vi "H2O_DIAL_NCAR_4CH_v4.10.vi"() -> ()   [LabVIEW 2012]
uses:
  C:/Users/H2ODial/Desktop/Shared Telescope WV DIAL Code/Libraries and VIs/PowerMeterCommands.dll
  Shared Telescope WV DIAL Code/Libraries and VIs/PowerMeterCommands.dll
  <vilib>/DAQmx/write.llb/DAQmx Write (Digital 1D Bool NChan 1Samp 1Line).vi
  <vilib>/DAQmx/miscellaneous.llb/DAQmx Fill In Error Info.vi
  <vilib>/Analysis/baseanly.llb/Mean (DBL).vi
  AMCS_Data.vi
  Libraries and VIs/Scalar_Data.vi
  <vilib>/Analysis/NI_AALBase.lvlib
  Libraries and VIs/Scalar_Data_2.vi
  Libraries and VIs/Scalar_Data_4.vi
  Libraries and VIs/Scalar_Data_3.vi
  Shared Telescope WV DIAL Code/bristol/CLDevIFace.dll
panel:
  out "FileHour":i32=21
  out "L_Count":i32=670
  out "sigma_off_total":dbl[](array[numeric])=[5.545093346002325e-25, 5.513698314781969e-25, 5.482392638165798e-25, 5.45117700346153e-25, 5.420052094490138e-25, 5.389018591101994e-25, 5.35807716859337e-25, 5.327228497243776e-25, 5.296473241817102e-25, 5.265812061058967e-25, 5.235245607190952e-25, 5.204774525540416e-25, 5.17439945396719e-25, 5.144121022534048e-25, 5.11393985302133e-25, 5.083856558516785e-25, 5.053871743064082e-25, 5.023986001219567e-25, 4.994199917728618e-25, 4.964514067155941e-25, 4.9349290135305775e-25, 4.90544531006438e-25, 4.876063498767343e-25, 4.846784110224529e-25, 4.817607663241581e-25, 4.788534664693006e-25, 4.759565609097595e-25, 4.730700978566929e-25, 4.70194124242593e-25, 4.673286857118099e-25, 4.644738265927707e-25, 4.616295898870687e-25, 4.587960172474658e-25, 4.5597314896431265e-25, 4.531610239560122e-25, 4.503596797514039e-25, 4.47569152481693e-25, 4.447894768684054e-25, 4.420206862206039e-25, 4.392628124203261e-25, 4.365158859275847e-25, 4.337799357659035e-25, 4.310549895246989e-25, 4.283410733576763e-25, 4.256382119799841e-25, 4.2294642867403195e-25, 4.202657452853169e-25, 4.175961822281299e-25, 4.149377584922389e-25, 4.1229049164465202e-25, 4.096543978372992e-25, 4.0702949181683236e-25, 4.0441578692843654e-25, 4.0181329512767607e-25, 3.992220269942415e-25, 3.96641991736463e-25, 3.9407319720804376e-25, 3.915156499210381e-25, 3.8896935505642936e-25, 3.8643431648416273e-25, 3.8391053677102475e-25, 3.813980172052376e-25, 3.788967578068652e-25, 3.764067573453576e-25, 3.7392801336269163e-25, 3.7146052218886312e-25, 3.6900427895717113e-25, 3.6655927763183676e-25, 3.6412551102130396e-25, 3.6170297080280375e-25, 3.592916475433481e-25, 3.568915307165587e-25, 3.5450260873191323e-25, 3.5212486894953557e-25, 3.49758297708119e-25, 3.4740288034404592e-25, 3.4505860121784583e-25, 3.427254437338488e-25, 3.4040339036361268e-25, 3.3809242267276765e-25, 3.3579252134124988e-25, 3.3350366619025945e-25, 3.312258362003964e-25, 3.2895900954264883e-25, 3.2670316359662337e-25, 3.2445827497597403e-25, 3.2222431955291055e-25, 3.2000127248258437e-25, 3.1778910822374647e-25, 3.155878005644869e-25, 3.133973226455684e-25, 3.1121764698225313e-25, 3.0904874548876633e-25, 3.0689058950047053e-25, 3.0474314979719436e-25, 3.0260639662437082e-25, 3.0048029971594525e-25, 2.9836482831758435e-25, 2.962599512058786e-25, 2.9416563671167466e-25, 2.9208185274060903e-25, 2.90008566793984e-25, 2.879457459893465e-25, 2.8589335708021117e-25, 2.8385136647823233e-25, 2.818197402689904e-25, 2.7979844423464204e-25, 2.7778744387231733e-25, 2.757867044107587e-25, 2.737961908312855e-25, 2.718158678842996e-25, 2.6984570010800424e-25, 2.6788565184392253e-25, 2.659356872568504e-25, 2.639957703488535e-25, 2.620658649780614e-25, 2.6014593487307293e-25, 2.582359436501918e-25, 2.5633585482778302e-25, 2.5444563184328377e-25, 2.5256523806624473e-25, 2.506946368147788e-25, 2.488337913696908e-25, 2.4698266498768704e-25, 2.4514122091801807e-25, 2.4330942241302343e-25, 2.4148723274426624e-25, 2.396746152144881e-25, 2.3787153317177266e-25, 2.360779500217858e-25, 2.3429382923989676e-25, 2.3251913438553717e-25, 2.30753829112614e-25, 2.289978771825043e-25, 2.272512424756057e-25, 2.25513889003242e-25, 2.2378578091878363e-25, 2.220668825283397e-25, 2.2035715830323156e-25, 2.1865657288915057e-25, 2.169650911171393e-25, 2.1528267801378837e-25, 2.1360929881158006e-25, 2.1194491895763e-25, 2.102895041236874e-25, 2.0864302021492868e-25, 2.070054333784623e-25, 2.0537671001224436e-25, 2.0375681677230244e-25, 2.0214572058106931e-25, 2.0054338863372052e-25, 1.989497884059814e-25, 1.9736488765949925e-25, 1.9578865444868876e-25, 1.9422105712539158e-25, 1.9266206434388185e-25, 1.9111164506623173e-25, 1.8956976856478284e-25, 1.8803640442671668e-25, 1.8651152255647924e-25, 1.8499509317774677e-25, 1.8348708683587619e-25, 1.8198747439799888e-25, 1.8049622705463732e-25, 1.7901331631884819e-25, 1.775387140257627e-25, 1.7607239233152573e-25, 1.7461432371095203e-25, 1.7316448095559218e-25, 1.717228371700267e-25, 1.7028936576867277e-25, 1.6886404047118466e-25, 1.6744683529761906e-25, 1.660377245632093e-25, 1.6463668287207736e-25, 1.632436851109196e-25, 1.618587064418851e-25, 1.604817222950476e-25, 1.5911270836042792e-25, 1.5775164057945997e-25, 1.56398495136209e-25, 1.5505324844802238e-25, 1.5371587715593366e-25, 1.5238635811467746e-25, 1.510646683824263e-25, 1.4975078521023343e-25, 1.4844468603128529e-25, 1.4714634844992623e-25, 1.4585575023049792e-25, 1.4457286928608944e-25, 1.4329768366725881e-25, 1.4203017155042415e-25, 1.407703112267118e-25, 1.3951808109034195e-25, 1.3827345962734493e-25, 1.3703642540430184e-25, 1.3580695705732947e-25, 1.3458503328084848e-25, 1.3337063281714564e-25, 1.3216373444562365e-25, 1.3096431697251984e-25, 1.2977235922113967e-25, 1.2858784002202707e-25, 1.2741073820391008e-25, 1.262410325845275e-25, 1.2507870196238964e-25, 1.2392372510878126e-25, 1.2277608076014726e-25, 1.2163574761105352e-25, 1.2050270430775917e-25, 1.193769294421569e-25, 1.182584015463539e-25, 1.1714709908803334e-25, 1.1604300046571814e-25, 1.1494608400603252e-25, 1.1385632795946503e-25, 1.1277371049919547e-25, 1.1169820971849576e-25, 1.1062980362989263e-25, 1.0956847016453476e-25, 1.0851418717240022e-25, 1.0746693242300533e-25, 1.0642668360671284e-25, 1.0539341833638053e-25, 1.0436711415027306e-25, 1.0334774851444859e-25, 1.0233529882683514e-25, 1.01329742420825e-25, 1.0033105656977957e-25, 9.93392184918038e-26, 9.835420535448986e-26, 9.737599428132508e-26, 9.640456235622354e-26, 9.543988662985507e-26, 9.44819441258607e-26, 9.353071184649082e-26, 9.258616677861991e-26, 9.164828590007729e-26, 9.071704618481929e-26, 8.979242460918443e-26, 8.887439815711605e-26, 8.79629438247936e-26, 8.705803862565375e-26, 8.615965959431582e-26, 8.526778379078846e-26, 8.438238830295678e-26, 8.350345024925896e-26, 8.263094678112063e-26, 8.176485508356415e-26, 8.090515237617101e-26, 8.0051815912957e-26, 7.920482298141068e-26, 7.836415090070007e-26, 7.752977702020669e-26, 7.67016787158364e-26, 7.587983338670006e-26, 7.506421845116342e-26, 7.425481134179741e-26, 7.345158949991444e-26, 7.265453037023949e-26, 7.186361139388167e-26, 7.107881000268466e-26, 7.030010361112887e-26, 6.95274696098591e-26, 6.876088535839326e-26, 6.800032817697419e-26, 6.724577533923724e-26, 6.64972040650064e-26, 6.575459151231174e-26, 6.501791477027899e-26, 6.428715085196855e-26, 6.356227668734542e-26, 6.284326911690598e-26, 6.213010488505251e-26, 6.142276063456507e-26, 6.072121290089713e-26, 6.002543810738931e-26]
  out "sigma_on_total":dbl[](array[numeric])=[3.742206868641341e-23, 3.7429612618018996e-23, 3.7434726015285955e-23, 3.743740073660256e-23, 3.743762939303223e-23, 3.7435405357585175e-23, 3.743072276917427e-23, 3.742357654081436e-23, 3.7413962365246194e-23, 3.7401876719276805e-23, 3.738731686678352e-23, 3.737028086692236e-23, 3.735076757163706e-23, 3.732877663344878e-23, 3.7304308504649446e-23, 3.7277364438773654e-23, 3.724794649375737e-23, 3.721605752921234e-23, 3.7181701208374216e-23, 3.7144881996422916e-23, 3.710560515815649e-23, 3.70638767581906e-23, 3.70197036542659e-23, 3.6973093497816675e-23, 3.6924054726011473e-23, 3.6872596563618015e-23, 3.681872900813485e-23, 3.67624628345753e-23, 3.67038095801539e-23, 3.664278154392267e-23, 3.6579391774321e-23, 3.6513654065279726e-23, 3.6445582944273624e-23, 3.637519366398915e-23, 3.6302502195208586e-23, 3.622752521321382e-23, 3.6150280088780594e-23, 3.6070784875244904e-23, 3.598905830029354e-23, 3.590511974858799e-23, 3.581898925616457e-23, 3.573068749038446e-23, 3.5640235739972726e-23, 3.5547655901165024e-23, 3.54529704616676e-23, 3.5356202489615237e-23, 3.525737561411073e-23, 3.515651401168645e-23, 3.505364239248806e-23, 3.494878598162465e-23, 3.4841970503851443e-23, 3.473322216892923e-23, 3.462256765124002e-23, 3.4510034074664904e-23, 3.4395648998215893e-23, 3.427944039316459e-23, 3.416143662923538e-23, 3.404166645697518e-23, 3.3920158987192733e-23, 3.37969436777507e-23, 3.367205030906827e-23, 3.354550897358153e-23, 3.3417350052058163e-23, 3.328760419548489e-23, 3.315630231166496e-23, 3.302347554430607e-23, 3.2889155251170917e-23, 3.27533729936037e-23, 3.261616051196446e-23, 3.247754971153086e-23, 3.23375726447253e-23, 3.2196261488718373e-23, 3.205364853547713e-23, 3.19097661668077e-23, 3.176464684282408e-23, 3.1618323081121953e-23, 3.1470827443725446e-23, 3.1322192516661925e-23, 3.117245089355038e-23, 3.102163516320947e-23, 3.086977788993837e-23, 3.071691160162447e-23, 3.0563068767728277e-23, 3.0408281792659305e-23, 3.0252582994336664e-23, 3.009600459155118e-23, 2.9938578690686444e-23, 2.9780337272750084e-23, 2.962131217604643e-23, 2.946153508575282e-23, 2.930103752101369e-23, 2.9139850820520734e-23, 2.897800613217805e-23, 2.8815534400324565e-23, 2.865246635517646e-23, 2.848883249985849e-23, 2.8324663100586776e-23, 2.8159988178125756e-23, 2.799483749410663e-23, 2.782924054415838e-23, 2.7663226547735467e-23, 2.749682443924372e-23, 2.733006285954302e-23, 2.7162970146927096e-23, 2.6995574332980244e-23, 2.682790312890641e-23, 2.6659983923935745e-23, 2.649184377777944e-23, 2.632350941081864e-23, 2.6155007202662802e-23, 2.5986363183953e-23, 2.581760303295213e-23, 2.5648752067227738e-23, 2.5479835244432992e-23, 2.5310877152951883e-23, 2.5141902012463274e-23, 2.497293366703312e-23, 2.480399558458463e-23, 2.4635110851539856e-23, 2.446630217375111e-23, 2.4297591870097065e-23, 2.4129001874018873e-23, 2.3960553731103502e-23, 2.3792268595329617e-23, 2.362416723389737e-23, 2.3456270019069583e-23, 2.3288596933533007e-23, 2.312116756693998e-23, 2.295400111844486e-23, 2.2787116395407354e-23, 2.262053181239011e-23, 2.2454265396775957e-23, 2.2288334785005983e-23, 2.212275722623987e-23, 2.195754958303483e-23, 2.1792728333801465e-23, 2.1628309573890534e-23, 2.146430901613271e-23, 2.130074199768713e-23, 2.113762347784294e-23, 2.097496804215243e-23, 2.0812789905176965e-23, 2.0651102914863584e-23, 2.0489920552598092e-23, 2.0329255938621748e-23, 2.016912183458992e-23, 2.0009530646282707e-23, 1.985049442932356e-23, 1.969202488994444e-23, 1.9534133391617796e-23, 1.937683095535943e-23, 1.922012826792432e-23, 1.906403568161712e-23, 1.890856322259072e-23, 1.8753720591546555e-23, 1.859951716803023e-23, 1.844596201948617e-23, 1.8293063898166304e-23, 1.81408312516416e-23, 1.7989272225213907e-23, 1.7838394664456345e-23, 1.7688206124341635e-23, 1.7538713867286325e-23, 1.7389924874884766e-23, 1.7241845847336097e-23, 1.7094483209391532e-23, 1.6947843116875922e-23, 1.6801931457577e-23, 1.6656753860882517e-23, 1.6512315696862732e-23, 1.6368622085850145e-23, 1.622567790001357e-23, 1.6083487768030452e-23, 1.594205608268292e-23, 1.580138700130045e-23, 1.566148445332034e-23, 1.5522352143670054e-23, 1.5383993557319484e-23, 1.5246411964932193e-23, 1.5109610424520557e-23, 1.4973591789856755e-23, 1.483835871096439e-23, 1.470391364184852e-23, 1.457025884208284e-23, 1.44373963827773e-23, 1.4305328150829033e-23, 1.4174055852080033e-23, 1.4043581016048575e-23, 1.3913905000586885e-23, 1.3785028995441017e-23, 1.3656954025283766e-23, 1.3529680956771185e-23, 1.3403210498416435e-23, 1.3277543207535687e-23, 1.3152679493069243e-23, 1.3028619619372588e-23, 1.2905363708994922e-23, 1.2782911748783776e-23, 1.2661263590622749e-23, 1.2540418956938074e-23, 1.242037744419567e-23, 1.2301138524969977e-23, 1.2182701552755436e-23, 1.2065065763949493e-23, 1.1948230282970344e-23, 1.1832194124132028e-23, 1.171695619484919e-23, 1.1602515299217322e-23, 1.1488870141083616e-23, 1.1376019326638179e-23, 1.1263961367813471e-23, 1.1152694685187567e-23, 1.1042217610009625e-23, 1.0932528389069634e-23, 1.0823625183746822e-23, 1.0715506077604429e-23, 1.0608169074156257e-23, 1.0501612102692001e-23, 1.039583301959786e-23, 1.0290829611229029e-23, 1.018659959594753e-23, 1.0083140626506824e-23, 9.9804502923851e-24, 9.878526122803352e-24, 9.777365587462413e-24, 9.676966100565002e-24, 9.577325021108697e-24, 9.478439656066443e-24, 9.380307262054806e-24, 9.282925047322609e-24, 9.186290174719204e-24, 9.090399760827992e-24, 8.99525088092127e-24, 8.900840569368358e-24, 8.807165820741605e-24, 8.714223592542418e-24, 8.622010806858814e-24, 8.530524351028378e-24, 8.43976108083452e-24, 8.349717820452325e-24, 8.260391364300474e-24, 8.17177847944076e-24, 8.083875906074953e-24, 7.996680359550302e-24, 7.910188530523382e-24, 7.82439708778345e-24, 7.739302679216129e-24, 7.654901931897875e-24, 7.571191454764531e-24, 7.488167838924493e-24, 7.405827658820855e-24, 7.324167473632377e-24, 7.243183828892898e-24, 7.162873255914744e-24, 7.08323227444656e-24, 7.004257393111837e-24, 6.92594510985425e-24, 6.84829191340583e-24, 6.771294284440056e-24, 6.694948695438127e-24, 6.61925161305231e-24, 6.5441994969420865e-24, 6.4697888027984255e-24, 6.396015981633993e-24, 6.322877480321177e-24, 6.250369743511404e-24, 6.178489213846078e-24, 6.107232331951147e-24, 6.036595538022163e-24, 5.9665752719973e-24, 5.897167974177331e-24, 5.828370086040087e-24, 5.760178050379199e-24, 5.692588312506595e-24, 5.625597320140846e-24, 5.559201524349974e-24, 5.493397379632804e-24]
  out "background start":u32=254
  in  "Tab Control 2":enum32{"WV ND narrow", "WV ND wide"}(tab)
  out "Water Vapor Number Density":dbl[][](graph)=[[1.2680479768439454, 1.3202516042203751, 1.2466197496175317, 1.2280093642600212, 1.215511773831901, 1.2105348281548287, 1.1395916012495166, 1.1067305037507909, 1.211680908117416, 1.1150520225241658, 0.9028509210070665, 0.999626740977495, 1.112519764094604, 1.0830051168590646, 1.1051016673343605, 1.0340014362362413, 0.9563318394019998, 0.8749899424248817, 0.6569427688166435, 0.6911306332585765, 0.9740975157789693, 0.8232451423116774, 0.4613358705650464, 0.5860350146191723, 0.7679146881331571, 0.6131055096448335, 0.5406940297681296, 0.5910374292314619, 0.6029116153592544, 0.6723771780478576, 0.5630576348126207, 0.27607446961895976, -0.01749521453207282, 0.05134104113894712, 0.38351694299457634, 0.31210340997150815, 0.5192660615667869, 0.3207502256246291, -0.5590638052858358, -0.19697175770808104, 0.290357801039229, 0.16997930227003574, 0.000565181425378715, 0.0777213720937388, 0.274413165706268, 0.22510786287864673, -0.03845493871274266, -0.01605108282141462, 0.20633781823881467, 0.04881741410965022, -0.04443222318813732, -0.1089065022769752, -0.13825380158949244, -0.195301928265506, -0.22841320864777703, -0.08789814039251888, -0.04911045471784868, -0.072053321499755, -0.1968438465853121, -0.1998200071916392, -0.34986328825729346, -0.07010646858360935, 0.004304911523472427, 0.09052944764014838, 0.6215372104587141, 0.2941766634729199, 0.13991908499406433, -0.09203647571773214, -0.43227440566149583, -0.18040901758326136, 0.1782000737791896, 0.28005188575082535, 0.8108049724719859, 0.9886103743450474, -0.30450896593774773, -0.456648818442852, -0.34182283513136774, -0.18537698516526777, 0.13525439428794223, 0.6719346065503385, 0.3369271024917734, -0.8212424706652944, -0.9185562874058523, -1.1507398852810957, -0.3049493711015754, 0.3698350068691422, 1.1772451365022465, 0.8428766659407354, 0.12818206437996593, -0.07094223815860062, 0.00805112352099952, 1.9525104698991527, 1.8576939577738627, -0.20658341078205697, -1.0904217576731, -0.5956468415233594, -0.5361531690334466, 0.5065001034620401, 2.9223505977863335, -0.1590587924697388, -0.6977580324857603, -1.150962383264831, -1.2170741124511153, 0.34690530103660205, 0.1733156353344592, 0.7684461900098062, -0.35416839232868624, -1.7263646552930005, 0.3621897789864032, 3.911100862551616, 0.8827863232756602, -1.017863455538243, -1.568063599658714, -0.22143032701187537, 1.242140967336172, -1.7268635429439803, 4.318958272485017, 2.064266232491873, -5.138194943835686, -5.40050193955499, -0.8895907950074605, -0.0162589252743628, 1.2642304881281694, 0.7410742796899519, 1.2285669310528016, 1.4331306918159583, -5.255004500798236, -1.954853692912569, 2.836859970643854, -0.3825909568082915, -2.428808674724871, -0.6206490502008231, -3.072824589959584, -3.0156166810939213, 5.376685838015374, 1.8132825198697586, 3.199752163267548, 3.5982866207249726, 1.4372215750905868, 3.60159507262911, 2.4435493248522477, 5.732224101200824, -0.24267757376801943, 0.6995422479855475, -0.21941327361205695, 11.621368511899782, -0.469972836003239, -5.804494817088179, -3.9716503700697317, -1.6398902133792508, -0.9586761554681651, -6.53457831663424, 2.772826250479864, 8.285755900638716, -11.086655577826983, -20.179919389211467, -8.368187418155868, -6.187458659564273, -3.1495433870624834, -1.6880188755098007, -2.41353736064144, 0.01477257735327296, 1.6274176320141638, -12.373453685636173, -0.37762438880298493, 3.3941243963967023, 6.728621633863314, 5.231280947377627, -3.2144676126386447, -10.093015424640182, -4.715847190164767, -3.527085021913163, -9.029971019551189, -1.0775786965773437, -0.2819156559857283, 0.8887576511862656, 1.499231811180272, 5.751283944699657, 6.186996432812196, 8.277394619269115, 3.5769758637090696, 8.744771202825868, 29.120235453359292, 3.114770818118839, 12.472711004967778, -0.6782934808279238, -8.581919813701292, 0.06596070683683264, 7.143821402458832, 2.1122302652281464, -1.2518869274439604, -5.918847062855048, -20.91762678432696, -11.572753850675706, -16.107993427906084, -22.021331252948098, -18.855175785746727, -28.35127359851436, -23.789277328398402, -7.38066480445351, -6.141605428675346, -1.7494212965347764, -21.137182078484393, 8.438381904160616, -0.8668390473239731, 11.829857128415734, 0.6826069125989869, 19.390806237590642, 7.969851920856497, 3.6613743164352948, 5.272661567115853, -0.41839368418776063, 14.868408915627047, 2.6767649073664153, 27.194917292609798, 5.294936128814359, 39.159305766395754, 11.475877642573526, 10.784829043961636, -7.5493135625502665, -7.289818504429609, 3.045057720742738, 12.434231506844423, -1.3677186641655195, -55.84861365452638, -10.099313020245248, -23.661623534891607, 2.59830573667955, -6.047291442635215, 10.15408041486899, 7.942595814581642, -5.915727747545152, -21.440412560127914, 4.551305232194775, 31.58931023941637, 6.061070485298637, 14.768953740359345, 1.853148102107566, -2.9222857829048805, -13.592186426951734, -21.423927313606022, -7.557110869802428, -6.16054913360661, -15.048295573119812, -26.837852249947648, -5.038109934424471, -16.65592286915807, -16.111921389113977, -2.787680794471786, 12.424779838783403, 24.879798152296868, 5.217385569325811, -1.1912340210717631, 32.712750276387524, 17.557582831701776, 18.022182963633615, -0.672807757576144, -7.671489186294683, -7.180011210333791, 3.8262308661908904, -19.548083734662818, -25.27246595618939, 15.881625911713707, -33.320141524743505, 1.3645434721760537, -48.34566107163499, 31.284470159209235, 9.768200503630595, 46.20057355060547, 37.57677416116322, 1.7480979349121049, 14.933958458615255, -14.305607378854123, -3.847555802912635, -6.126399007920727, 26.579745674967977, 0.0, 0.0, 0.0, 0.0]]
  out "Water Vapor Number Density 2":dbl[][](graph)=[[nan, nan, nan, nan, nan, nan, nan, nan, nan, nan, nan, nan, nan, nan, nan, nan, nan, nan, nan, nan, nan, nan, nan, nan, nan, nan, nan, nan, nan, nan, nan, nan, nan, nan, nan, nan, nan, nan, nan, nan, nan, nan, nan, nan, nan, nan, nan, nan, nan, nan, nan, nan, nan, nan, nan, nan, nan, nan, nan, nan, nan, nan, nan, nan, nan, nan, nan, nan, nan, nan, nan, nan, nan, nan, nan, nan, nan, nan, nan, nan, nan, nan, nan, nan, nan, nan, nan, nan, nan, nan, nan, nan, nan, nan, nan, nan, nan, nan, nan, nan, nan, nan, nan, nan, nan, nan, nan, nan, nan, nan, nan, nan, nan, nan, nan, nan, nan, nan, nan, nan, nan, nan, nan, nan, nan, nan, nan, nan, nan, nan, nan, nan, nan, nan, nan, nan, nan, nan, nan, nan, nan, nan, nan, nan, nan, nan, nan, nan, nan, nan, nan, nan, nan, nan, nan, nan, nan, nan, nan, nan, nan, nan, nan, nan, nan, nan, nan, nan, nan, nan, nan, nan, nan, nan, nan, nan, nan, nan, nan, nan, nan, nan, nan, nan, nan, nan, nan, nan, nan, nan, nan, nan, nan, nan, nan, nan, nan, nan, nan, nan, nan, nan, nan, nan, nan, nan, nan, nan, nan, nan, nan, nan, nan, nan, nan, nan, nan, nan, nan, nan, nan, nan, nan, nan, nan, nan, nan, nan, nan, nan, nan, nan, nan, nan, nan, nan, nan, nan, nan, nan, nan, nan, nan, nan, nan, nan, nan, nan, nan, nan, nan, nan, nan, nan, nan, nan, nan, nan, nan, nan, nan, nan, nan, nan, nan, nan, nan, nan, nan, nan, nan, nan, nan, nan, nan, nan, 0.0, 0.0, 0.0, 0.0]] caption="Water Vapor Number Density"
  out "RingBuffer offline near":dbl[][](array[numeric])
  out "RingBuffer aerosol near":dbl[][](array[numeric])
  in  "?":T1(tab)
  out "NRB":dbl[][](graph)=[[9.51278879590776e-05, 0.00036736222385929344, 0.0009696039747746865, 0.0021843657130871177, 0.004359654548929603, 0.007802864741874353, 0.013014703836101467, 0.02060533051224256, 0.03146060795429024, 0.046959030807481726, 0.0678048687499723, 0.09342168584581641, 0.12281616662413099, 0.1575367235865086, 0.2014933941807303, 0.2548433715326564, 0.3015968571725113, 0.3193646395873207, 0.3004191432597648, 0.26013290449992643, 0.22798346806755207, 0.21943400296813875, 0.2275771783765998, 0.2372234376509649, 0.24429560064081607, 0.24512412482417928, 0.24536717125801213, 0.24762951835386865, 0.2498067954541109, 0.25738204608441556, 0.2650184438269311, 0.266505665307847, 0.25954174788940604, 0.25147217747349476, 0.24866712029890656, 0.25203609405791444, 0.2574262780526806, 0.2577333879318053, 0.2620666032227746, 0.26635167704466667, 0.2674145941970921, 0.26990645707287164, 0.26911303199251146, 0.2604148011286556, 0.23669053453564673, 0.2179862244041704, 0.2066933370358258, 0.19576119211317636, 0.19133101650711362, 0.18485294608172922, 0.18128198319409594, 0.17576664659048485, 0.165238972396633, 0.17136897606019946, 0.17953548683561496, 0.17334622829639615, 0.17648140922465796, 0.17420168410020678, 0.16803952854530627, 0.1576993176913969, 0.15475730101058932, 0.1595121046589469, 0.15709966319713814, 0.1595123603337601, 0.15779489746433006, 0.1485422555586342, 0.15130820351537683, 0.1549906493075145, 0.156097548274157, 0.16231039870313946, 0.15326148073543255, 0.13990101196195603, 0.1274117713860531, 0.12753497683743673, 0.12593798393644068, 0.12986071621501788, 0.1378627148502252, 0.14671916993215134, 0.14277488070748326, 0.13199922308008497, 0.11931334905407015, 0.10006969869077414, 0.10885979306717863, 0.10223011044380045, 0.08868056856494021, 0.11118102471153075, 0.11889495211014338, 0.10682138087472741, 0.10792519144207921, 0.10413226475778514, 0.10490525589365854, 0.1089706144353422, 0.0922016249640525, 0.10845418738267291, 0.12364482791870392, 0.10239643656944038, 0.09871453530122709, 0.10616675750936692, 0.09234449068084331, 0.08483751630681531, 0.09228504737773939, 0.07381893444587825, 0.09677235292828874, 0.12342089685181161, 0.09911888479643274, 0.08436035978343479, 0.095841515137535, 0.07641212555367932, 0.08429861208683964, 0.11400554405042382, 0.06152825263759745, 0.0718210215497355, 0.09946406686193539, 0.08586974505477675, 0.07572010602640725, 0.07022587117206305, 0.08454111862274616, 0.07580339899918805, 0.0654027741936649, 0.06407494109068737, 0.03630357753414599, 0.028528411599848726, 0.07838940518302631, 0.05630101319037285, 0.02349922835465965, 0.06379145345992414, 0.0796366522569814, 0.06306598691540219, 0.04625832484110327, 0.04856370830629811, 0.03546859566700341, 0.017705206303777293, 0.03456856936898238, 0.039133076923510444, 0.04826789097673306, 0.08715921764673557, 0.08633272667273073, 0.05508200085803232, 0.016007835132029746, 0.014032597012615059, 0.035868185285051514, 0.06399632015792558, 0.07257433906314756, 0.052972856864475094, 0.06436207197855372, 0.05525441837763387, 0.05114870967825508, 0.03664121279090114, 0.008813753598525542, 0.03890464836677183, 0.024880149196757902, 6.935515359034072e-05, 0.05848376936627277, 0.08327911093385978, 0.05821969500268925, 0.0183365076503128, 0.03013390699399059, 0.04129163228994843, -0.015576404175476122, 0.006801043432157407, 0.029257308744871542, 0.02765232858871801, 0.051922229609615726, 0.027834695886394725, -0.009112412120185228, -0.031453841311389535, -0.0020092571921666888, -0.03168680942222466, -0.023491631287369676, -0.009673047209305898, 0.0017336085630241021, -0.011567115235992173, -0.07178334421930371, 0.01713180099525608, 0.0023902384135706914, -0.017341798105605398, 0.04182710983456895, 0.04586780207586087, 0.017529386436691215, 0.0712200416507646, 0.11627013164691559, 0.0007208956386353457, 0.015180007111357833, 0.03313199560294472, 0.003955451555402569, 0.02671622124135212, 0.03487727978386048, -0.0012201268762939408, -0.016647362604973827, 0.02516844995689965, 0.042545403079511025, -0.009572147374501794, -0.046710987385968024, -0.003417591357927953, -0.012727253291828954, 0.0022775659709700045, -0.05376402241926917, -0.03151005181564948, 0.06550191997733727, -0.021643389359619365, 0.016039118018739265, 0.05524267519564321, -0.018431836946977913, -0.03110635327998249, 0.09158874792328617, 0.03277053892351768, -0.06739986672528231, -0.001493536927794845, 0.003409240951614078, 0.05474055580423485, 0.0260276884957026, 0.04482611634893263, 0.006094585634350449, -0.06602103908536458, 0.04957283704791029, 0.17521330970544094, 0.09202325530080904, 0.0010342906753564236, 0.033437784719746934, 0.07188312690625626, -0.006267752708116765, -0.06642628935118662, 0.039335453238188586, 0.07922784529542683, 0.060940273775269865, -0.01613725395431167, -0.011446543232621436, -0.02422654734349428, -0.08937474017950266, 0.040851199666653, 0.0031636088550846117, 0.018338523155800972, 0.16619036982847582, 0.18713975921775372, 0.1255373780157112, -0.03954072939155353, -0.06095277001319983, -0.13798346059336897, -0.1820112578708726, -0.0960058821617835, -0.08264182808569707, -0.004219231173654489, 0.08991465995387495, -0.09364789062420142, -0.08428174273311403, 0.07284664904265148, -0.0639157506852364, -0.10597462419587435, -0.08705626540934279, -0.0279548110652071, -0.018722909667535502, 0.009722170841312864, 0.0482290235942173, 0.05950500732234233, 0.05509450497193836, 0.013721964583500218, 0.017546957720725162, -0.12718149187333866, -0.04888191803092092, 0.10927695246621658, -0.04069339630537961, -0.14660977899121705, -0.07895306828521932, 0.04989876945873567, 0.14514201565848814, 0.06791537793275075, 0.03766415714739259, 0.04468455712188757, -0.13282729576268232, -0.027135617164868838, 0.13249813367131774, -0.01643464950847608, 0.10509635757812334, 0.1058677044041271, -0.16435741370453516, -0.0769470368819275, 0.014625993003182968, 0.0, 0.0, 0.0]] caption="Water Vapor Number Density"
  out "NRB 2":dbl[][](graph) caption="Water Vapor Number Density"
  out "raw counts":dbl[][](graph)=[[82.92, 64.92, 95.92, 112.92, 117.92, 189.92000000000002, 214.92000000000002, 260.92, 300.92, 381.92, 437.92, 522.92, 596.92, 721.92, 743.92, 839.92, 938.92, 945.92, 900.92, 728.92, 486.92, 466.92, 421.92, 423.92, 382.92, 406.92, 325.92, 325.92, 279.92, 255.92000000000002, 258.92, 232.92000000000002, 258.92, 234.92000000000002, 198.92000000000002, 164.92000000000002, 174.92000000000002, 153.92000000000002, 172.92000000000002, 165.92000000000002, 148.92000000000002, 132.92000000000002, 158.92000000000002, 131.92000000000002, 120.92, 105.92, 111.92, 55.92, 51.92, 66.92, 68.92, 67.92, 41.92, 62.92, 57.92, 51.92, 32.92, 66.92, 22.92, 40.92, 37.92, 62.92, 21.92, 33.92, 15.920000000000002, 28.92, 20.92, 31.92, 25.92, 26.92, 30.92, 19.92, 10.920000000000002, 32.92, 8.920000000000002, 9.920000000000002, 20.92, 14.920000000000002, 31.92, 28.92, 23.92, 6.920000000000002, 9.920000000000002, 6.920000000000002, 24.92, 14.920000000000002, 10.920000000000002, 8.920000000000002, 7.920000000000002, -2.0799999999999983, 10.920000000000002, -10.079999999999998, -3.0799999999999983, -0.0799999999999983, 22.92, -2.0799999999999983, 18.92, 22.92, 10.920000000000002, 36.92, -9.079999999999998, 24.92, 8.920000000000002, 14.920000000000002, 13.920000000000002, 19.92, 3.9200000000000017, 5.920000000000002, -3.0799999999999983, 13.920000000000002, 12.920000000000002, -12.079999999999998, 6.920000000000002, 5.920000000000002, 5.920000000000002, -3.0799999999999983, 11.920000000000002, 19.92, -7.079999999999998, 23.92, -13.079999999999998, -1.0799999999999983, -7.079999999999998, -8.079999999999998, 5.920000000000002, -5.079999999999998, 7.920000000000002, -3.0799999999999983, 9.920000000000002, 1.9200000000000017, 18.92, -8.079999999999998, 7.920000000000002, -2.0799999999999983, 13.920000000000002, -9.079999999999998, 5.920000000000002, -5.079999999999998, -6.079999999999998, -1.0799999999999983, -3.0799999999999983, -0.0799999999999983, -4.079999999999998, 12.920000000000002, -1.0799999999999983, 20.92, -17.08, -0.0799999999999983, 2.9200000000000017, 5.920000000000002, 12.920000000000002, 9.920000000000002, -5.079999999999998, 0.9200000000000017, -9.079999999999998, 1.9200000000000017, -11.079999999999998, 1.9200000000000017, -7.079999999999998, -15.079999999999998, -1.0799999999999983, -1.0799999999999983, -5.079999999999998, 9.920000000000002, 18.92, 1.9200000000000017, -2.0799999999999983, -4.079999999999998, 14.920000000000002, -5.079999999999998, 7.920000000000002, -10.079999999999998, -7.079999999999998, -14.079999999999998, 8.920000000000002, 7.920000000000002, -6.079999999999998, 1.9200000000000017, 10.920000000000002, -5.079999999999998, 1.9200000000000017, -0.0799999999999983, -19.08, -0.0799999999999983, 13.920000000000002, -0.0799999999999983, 13.920000000000002, 9.920000000000002, -7.079999999999998, -12.079999999999998, 4.920000000000002, 17.92, -2.0799999999999983, -9.079999999999998, 8.920000000000002, 5.920000000000002, 7.920000000000002, -10.079999999999998, 3.9200000000000017, 15.920000000000002, 2.9200000000000017, -0.0799999999999983, 10.920000000000002, 2.9200000000000017, -6.079999999999998, -1.0799999999999983, -10.079999999999998, -2.0799999999999983, 4.920000000000002, -3.0799999999999983, -1.0799999999999983, 2.9200000000000017, 1.9200000000000017, -11.079999999999998, 7.920000000000002, 8.920000000000002, 11.920000000000002, 5.920000000000002, -1.0799999999999983, -9.079999999999998, 12.920000000000002, 7.920000000000002, 4.920000000000002, 8.920000000000002, -2.0799999999999983, -1.0799999999999983, -7.079999999999998, -3.0799999999999983, -5.079999999999998, -6.079999999999998, -7.079999999999998, -16.08, -8.079999999999998, 7.920000000000002, -0.0799999999999983, 11.920000000000002, 1.9200000000000017, 2.9200000000000017, -7.079999999999998, 0.9200000000000017, 0.9200000000000017, -2.0799999999999983, 1.9200000000000017, 12.920000000000002, -11.079999999999998, -12.079999999999998, -0.0799999999999983, -19.08, 1.9200000000000017, -20.08, -11.079999999999998, -14.079999999999998, 12.920000000000002, -10.079999999999998, 8.920000000000002, 1.9200000000000017, -1.0799999999999983, 3.9200000000000017, -14.079999999999998, -8.079999999999998, 6.920000000000002, -5.079999999999998, -4.079999999999998, -0.0799999999999983, 4.920000000000002, -6.079999999999998, 10.920000000000002, 9.920000000000002, -7.079999999999998, -9.079999999999998, 16.92, 8.920000000000002, 8.920000000000002, -1.0799999999999983, -6.079999999999998, -14.079999999999998, 0.9200000000000017, -6.079999999999998, -1.0799999999999983, 0.0]] caption="Water Vapor Number Density"
  out "raw counts near":dbl[][](graph) caption="Water Vapor Number Density"
  out "Aerosol Smoothed 2":dbl[](array[numeric])
  out "Off-Line Smoothed 2":dbl[](array[numeric])
  out "Off-Line Bin Readings 2":dbl[](array[numeric])
  out "On-Line Smoothed 2":dbl[](array[numeric])
  out "On-Line Bin Readings 2":dbl[](array[numeric])
  in  "stop":bool
  in  "Reset Average":bool=TRUE
  in  "Save Data?":bool=TRUE
  in  "Collect Data?":bool=TRUE
  in  "ILX Address":i32=6 min=0 step=1
  in  "Lambda On DBR Current":dbl=171.13999999999868
  in  "Lambda Off DBR Current":dbl=172.9499999999997
  in  "Tab Control":T2(tab)=enum."NRB"
  out "Water Vapor Number Density  2":cluster{"Y":dbl[], "Y":dbl[]}[](graph)=[{"Y"=array[276 elements], "Y"=array[280 elements]}, {"Y"=[nan, nan, nan, nan, nan, nan, nan, nan, nan, nan, nan, nan, nan, nan, nan, nan, nan, nan, nan, nan, nan, nan, nan, nan, nan, nan, nan, nan, nan, nan, nan, nan, nan, nan, nan, nan, nan, nan, nan, nan, nan, nan, nan, nan, nan, nan, nan, nan, nan, nan, nan, nan, nan, nan, nan, nan, nan, nan, nan, nan, nan, nan, nan, nan, nan, nan, nan, nan, nan, nan, nan, nan, nan, nan, nan, nan, nan, nan, nan, nan, nan, nan, nan, nan, nan, nan, nan, nan, nan, nan, nan, nan, nan, nan, nan, nan, nan, nan, nan, nan, nan, nan, nan, nan, nan, nan, nan, nan, nan, nan, nan, nan, nan, nan, nan, nan, nan, nan, nan, nan, nan, nan, nan, nan, nan, nan, nan, nan, nan, nan, nan, nan, nan, nan, nan, nan, nan, nan, nan, nan, nan, nan, nan, nan, nan, nan, nan, nan, nan, nan, nan, nan, nan, nan, nan, nan, nan, nan, nan, nan, nan, nan, nan, nan, nan, nan, nan, nan, nan, nan, nan, nan, nan, nan, nan, nan, nan, nan, nan, nan, nan, nan, nan, nan, nan, nan, nan, nan, nan, nan, nan, nan, nan, nan, nan, nan, nan, nan, nan, nan, nan, nan, nan, nan, nan, nan, nan, nan, nan, nan, nan, nan, nan, nan, nan, nan, nan, nan, nan, nan, nan, nan, nan, nan, nan, nan, nan, nan, nan, nan, nan, nan, nan, nan, nan, nan, nan, nan, nan, nan, nan, nan, nan, nan, nan, nan, nan, nan, nan, nan, nan, nan, nan, nan, nan, nan, nan, nan, nan, nan, nan, nan, nan, nan, nan, nan, nan, nan, nan, nan, nan, nan, nan, nan, nan, nan], "Y"=array[280 elements]}]
  out "Absolute Humidity":cluster{"Y":dbl[], "Y":dbl[]}[](graph)=[{"Y"=array[276 elements], "Y"=array[280 elements]}, {"Y"=[nan, nan, nan, nan, nan, nan, nan, nan, nan, nan, nan, nan, nan, nan, nan, nan, nan, nan, nan, nan, nan, nan, nan, nan, nan, nan, nan, nan, nan, nan, nan, nan, nan, nan, nan, nan, nan, nan, nan, nan, nan, nan, nan, nan, nan, nan, nan, nan, nan, nan, nan, nan, nan, nan, nan, nan, nan, nan, nan, nan, nan, nan, nan, nan, nan, nan, nan, nan, nan, nan, nan, nan, nan, nan, nan, nan, nan, nan, nan, nan, nan, nan, nan, nan, nan, nan, nan, nan, nan, nan, nan, nan, nan, nan, nan, nan, nan, nan, nan, nan, nan, nan, nan, nan, nan, nan, nan, nan, nan, nan, nan, nan, nan, nan, nan, nan, nan, nan, nan, nan, nan, nan, nan, nan, nan, nan, nan, nan, nan, nan, nan, nan, nan, nan, nan, nan, nan, nan, nan, nan, nan, nan, nan, nan, nan, nan, nan, nan, nan, nan, nan, nan, nan, nan, nan, nan, nan, nan, nan, nan, nan, nan, nan, nan, nan, nan, nan, nan, nan, nan, nan, nan, nan, nan, nan, nan, nan, nan, nan, nan, nan, nan, nan, nan, nan, nan, nan, nan, nan, nan, nan, nan, nan, nan, nan, nan, nan, nan, nan, nan, nan, nan, nan, nan, nan, nan, nan, nan, nan, nan, nan, nan, nan, nan, nan, nan, nan, nan, nan, nan, nan, nan, nan, nan, nan, nan, nan, nan, nan, nan, nan, nan, nan, nan, nan, nan, nan, nan, nan, nan, nan, nan, nan, nan, nan, nan, nan, nan, nan, nan, nan, nan, nan, nan, nan, nan, nan, nan, nan, nan, nan, nan, nan, nan, nan, nan, nan, nan, nan, nan, nan, nan, nan, nan, nan, nan], "Y"=array[280 elements]}]
  out "NRB plot":cluster{"Y":dbl[], "Y":dbl[]}[](graph)
  in  "background length":i32=25
  out "Correction":cluster{"Y":dbl[], "Y":dbl[]}[](graph)=[{"Y"=array[277 elements], "Y"=array[280 elements]}, {"Y"=[1.0, 1.0, 1.0, 1.0, 1.0, 1.0, 1.0, 1.0, 1.0, 1.0, 1.0, 1.0, 1.0, 1.0, 1.0, 1.0, 1.0, 1.0, 1.0, 1.0, 1.0, 1.0, 1.0, 1.0, 1.0, 1.0, 1.0, 1.0, 1.0, 1.0, 1.0, 1.0, 1.0, 1.0, 1.0, 1.0, 1.0, 1.0, 1.0, 1.0, 1.0, 1.0, 1.0, 1.0, 1.0, 1.0, 1.0, 1.0, 1.0, 1.0, 1.0, 1.0, 1.0, 1.0, 1.0, 1.0, 1.0, 1.0, 1.0, 1.0, 1.0, 1.0, 1.0, 1.0, 1.0, 1.0, 1.0, 1.0, 1.0, 1.0, 1.0, 1.0, 1.0, 1.0, 1.0, 1.0, 1.0, 1.0, 1.0, 1.0, 1.0, 1.0, 1.0, 1.0, 1.0, 1.0, 1.0, 1.0, 1.0, 1.0, 1.0, 1.0, 1.0, 1.0, 1.0, 1.0, 1.0, 1.0, 1.0, 1.0, 1.0, 1.0, 1.0, 1.0, 1.0, 1.0, 1.0, 1.0, 1.0, 1.0, 1.0, 1.0, 1.0, 1.0, 1.0, 1.0, 1.0, 1.0, 1.0, 1.0, 1.0, 1.0, 1.0, 1.0, 1.0, 1.0, 1.0, 1.0, 1.0, 1.0, 1.0, 1.0, 1.0, 1.0, 1.0, 1.0, 1.0, 1.0, 1.0, 1.0, 1.0, 1.0, 1.0, 1.0, 1.0, 1.0, 1.0, 1.0, 1.0, 1.0, 1.0, 1.0, 1.0, 1.0, 1.0, 1.0, 1.0, 1.0, 1.0, 1.0, 1.0, 1.0, 1.0, 1.0, 1.0, 1.0, 1.0, 1.0, 1.0, 1.0, 1.0, 1.0, 1.0, 1.0, 1.0, 1.0, 1.0, 1.0, 1.0, 1.0, 1.0, 1.0, 1.0, 1.0, 1.0, 1.0, 1.0, 1.0, 1.0, 1.0, 1.0, 1.0, 1.0, 1.0, 1.0, 1.0, 1.0, 1.0, 1.0, 1.0, 1.0, 1.0, 1.0, 1.0, 1.0, 1.0, 1.0, 1.0, 1.0, 1.0, 1.0, 1.0, 1.0, 1.0, 1.0, 1.0, 1.0, 1.0, 1.0, 1.0, 1.0, 1.0, 1.0, 1.0, 1.0, 1.0, 1.0, 1.0, 1.0, 1.0, 1.0, 1.0, 1.0, 1.0, 1.0, 1.0, 1.0, 1.0, 1.0, 1.0, 1.0, 1.0, 1.0, 1.0, 1.0, 1.0, 1.0, 1.0, 1.0, 1.0, 1.0, 1.0, 1.0, 1.0, 1.0, 1.0, 1.0, 1.0, 1.0, 1.0, 1.0, 1.0, 1.0, 1.0, 1.0, 1.0, 1.0, 1.0, 1.0, 1.0, 1.0, 1.0, 1.0, 1.0, 1.0, 1.0, 1.0], "Y"=array[280 elements]}]
  in  "dead time":dbl=3.7e-08
  out "Optical Depth":cluster{"Y":dbl[], "Y":dbl[]}[](graph) caption="XY Graph"
  out "RingBuffer offline far":dbl[][](array[numeric])
  out "RingBuffer aerosol far":dbl[][](array[numeric])
  in  "Weather":T3(tab)=enum."Pulse Energy (Micro Joule)"
  out "Temperature (C)":dbl(graph)=15.103479853479854
  out "Pressure (mb)":dbl(graph)=844.848901098901
  out "Relative Humdity (%)":dbl(graph)=39.287240537240535
  out "Pulse Energy (Micro Joule)":T4(graph)={"Online Pulse Energy"=4.393014285714285, "Pulse Energy Offline"=4.401922857142857}
  out "?":cluster{"mean":dbl, "mean":dbl}(graph)={"mean"=16816.0, "mean"=0.0}
  out "Index":i32=141
  out "Aerosol Smoothed":dbl[](array[numeric])=[84.45266666666667, 81.536, 95.63600000000001, 121.16933333333333, 154.736, 192.26933333333335, 235.536, 285.4026666666666, 344.1526666666666, 415.8693333333334, 495.96933333333345, 573.8693333333335, 642.5026666666668, 710.2526666666668, 790.8693333333334, 878.5693333333334, 920.7360000000001, 869.9860000000001, 735.2360000000001, 575.2526666666668, 457.68600000000004, 401.55266666666665, 381.086, 364.8693333333333, 346.33599999999996, 321.3526666666666, 298.336, 280.00266666666664, 263.35266666666666, 253.56933333333336, 244.53600000000003, 230.8026666666667, 211.38600000000002, 192.96933333333337, 180.086, 172.536, 166.836, 158.36933333333332, 152.88599999999997, 147.71933333333334, 141.1693333333333, 135.78599999999997, 129.16933333333333, 119.386, 103.75266666666667, 91.45266666666669, 83.06933333333333, 75.436, 70.75266666666667, 65.65266666666666, 61.885999999999996, 57.71933333333333, 52.236, 52.186, 52.702666666666666, 49.086, 48.236, 45.98599999999999, 42.86933333333333, 38.90266666666666, 36.93599999999999, 36.852666666666664, 35.15266666666666, 34.586, 33.16933333333333, 30.285999999999994, 29.935999999999996, 29.76933333333333, 29.11933333333333, 29.419333333333334, 27.002666666666663, 23.969333333333324, 21.23599999999999, 20.685999999999993, 19.885999999999996, 19.96933333333333, 20.65266666666666, 21.419333333333327, 20.319333333333333, 18.319333333333333, 16.152666666666665, 13.219333333333333, 14.036, 12.869333333333332, 10.902666666666665, 13.352666666666664, 13.952666666666666, 12.252666666666666, 12.102666666666664, 11.419333333333332, 11.252666666666666, 11.436, 9.469333333333331, 10.902666666666665, 12.169333333333332, 9.86933333333333, 9.319333333333333, 9.819333333333333, 8.369333333333332, 7.535999999999998, 8.035999999999998, 6.302666666666665, 8.102666666666664, 10.135999999999997, 7.985999999999999, 6.6693333333333324, 7.435999999999998, 5.819333333333332, 6.302666666666665, 8.36933333333333, 4.435999999999999, 5.0859999999999985, 6.919333333333332, 5.8693333333333335, 5.086, 4.636, 5.485999999999999, 4.836, 4.102666666666667, 3.9526666666666674, 2.2026666666666674, 1.702666666666667, 4.602666666666667, 3.252666666666667, 1.3360000000000003, 3.5693333333333337, 4.386, 3.419333333333334, 2.469333333333334, 2.552666666666667, 1.8360000000000003, 0.9026666666666672, 1.7360000000000007, 1.9360000000000004, 2.352666666666667, 4.186, 4.086, 2.5693333333333337, 0.7360000000000005, 0.6360000000000005, 1.6026666666666671, 2.8193333333333337, 3.1526666666666667, 2.269333333333334, 2.7193333333333336, 2.302666666666667, 2.102666666666667, 1.4860000000000004, 0.3526666666666671, 1.5360000000000005, 0.9693333333333338, 0.002666666666667039, 2.2193333333333336, 3.1193333333333335, 2.152666666666667, 0.6693333333333338, 1.0860000000000005, 1.4693333333333338, -0.5473333333333329, 0.23600000000000054, 1.0026666666666673, 0.9360000000000003, 1.7360000000000002, 0.9193333333333338, -0.2973333333333329, -1.0139999999999996, -0.06399999999999956, -0.997333333333333, -0.7306666666666662, -0.2973333333333329, 0.052666666666667084, -0.3473333333333328, -2.130666666666666, 0.5026666666666672, 0.06933333333333391, -0.49733333333333285, 1.1860000000000004, 1.2860000000000005, 0.4860000000000004, 1.9526666666666666, 3.1526666666666667, 0.019333333333333758, 0.40266666666666706, 0.8693333333333337, 0.10266666666666707, 0.6860000000000004, 0.8860000000000005, -0.030666666666666287, -0.41399999999999965, 0.6193333333333337, 1.0360000000000005, -0.23066666666666624, -1.1139999999999997, -0.08066666666666626, -0.2973333333333329, 0.052666666666667084, -1.2306666666666664, -0.7139999999999996, 1.4693333333333338, -0.4806666666666663, 0.35266666666666713, 1.2026666666666672, -0.3973333333333329, -0.6639999999999996, 1.9360000000000004, 0.6859999999999999, -1.3973333333333333, -0.03066666666666626, 0.06933333333333375, 1.1026666666666671, 0.5193333333333338, 0.8860000000000005, 0.11933333333333374, -1.2806666666666664, 0.952666666666667, 3.3360000000000003, 1.7360000000000007, 0.019333333333333758, 0.6193333333333337, 1.3193333333333337, -0.11399999999999966, -1.197333333333333, 0.7026666666666671, 1.4026666666666672, 1.0693333333333337, -0.28066666666666623, -0.19733333333333292, -0.4139999999999996, -1.5139999999999996, 0.6860000000000004, 0.052666666666667084, 0.3026666666666671, 2.7193333333333336, 3.0359999999999996, 2.0193333333333334, -0.6306666666666663, -0.9639999999999995, -2.1639999999999997, -2.830666666666666, -1.4806666666666661, -1.2639999999999996, -0.06399999999999961, 1.3526666666666671, -1.397333333333333, -1.2473333333333332, 1.0693333333333337, -0.9306666666666662, -1.5306666666666662, -1.2473333333333327, -0.39733333333333287, -0.26399999999999957, 0.13600000000000045, 0.6693333333333338, 0.8193333333333338, 0.7526666666666672, 0.18600000000000042, 0.2360000000000004, -1.697333333333333, -0.647333333333333, 1.4360000000000004, -0.5306666666666663, -1.8973333333333329, -1.0139999999999996, 0.6360000000000003, 1.8360000000000003, 0.8526666666666671, 0.4693333333333337, 0.5526666666666671, -1.6306666666666663, -0.3306666666666662, 1.6026666666666671, -0.19733333333333286, 1.252666666666667, 1.252666666666667, -1.9306666666666663, -0.8973333333333331, 0.16933333333333372]
  out "Off-Line  Bin Readings":dbl[](array[numeric])=[167.0, 149.0, 180.0, 197.0, 202.0, 274.0, 299.0, 345.0, 385.0, 466.0, 522.0, 607.0, 681.0, 806.0, 828.0, 924.0, 1023.0, 1030.0, 985.0, 813.0, 571.0, 551.0, 506.0, 508.0, 467.0, 491.0, 410.0, 410.0, 364.0, 340.0, 343.0, 317.0, 343.0, 319.0, 283.0, 249.0, 259.0, 238.0, 257.0, 250.0, 233.0, 217.0, 243.0, 216.0, 205.0, 190.0, 196.0, 140.0, 136.0, 151.0, 153.0, 152.0, 126.0, 147.0, 142.0, 136.0, 117.0, 151.0, 107.0, 125.0, 122.0, 147.0, 106.0, 118.0, 100.0, 113.0, 105.0, 116.0, 110.0, 111.0, 115.0, 104.0, 95.0, 117.0, 93.0, 94.0, 105.0, 99.0, 116.0, 113.0, 108.0, 91.0, 94.0, 91.0, 109.0, 99.0, 95.0, 93.0, 92.0, 82.0, 95.0, 74.0, 81.0, 84.0, 107.0, 82.0, 103.0, 107.0, 95.0, 121.0, 75.0, 109.0, 93.0, 99.0, 98.0, 104.0, 88.0, 90.0, 81.0, 98.0, 97.0, 72.0, 91.0, 90.0, 90.0, 81.0, 96.0, 104.0, 77.0, 108.0, 71.0, 83.0, 77.0, 76.0, 90.0, 79.0, 92.0, 81.0, 94.0, 86.0, 103.0, 76.0, 92.0, 82.0, 98.0, 75.0, 90.0, 79.0, 78.0, 83.0, 81.0, 84.0, 80.0, 97.0, 83.0, 105.0, 67.0, 84.0, 87.0, 90.0, 97.0, 94.0, 79.0, 85.0, 75.0, 86.0, 73.0, 86.0, 77.0, 69.0, 83.0, 83.0, 79.0, 94.0, 103.0, 86.0, 82.0, 80.0, 99.0, 79.0, 92.0, 74.0, 77.0, 70.0, 93.0, 92.0, 78.0, 86.0, 95.0, 79.0, 86.0, 84.0, 65.0, 84.0, 98.0, 84.0, 98.0, 94.0, 77.0, 72.0, 89.0, 102.0, 82.0, 75.0, 93.0, 90.0, 92.0, 74.0, 88.0, 100.0, 87.0, 84.0, 95.0, 87.0, 78.0, 83.0, 74.0, 82.0, 89.0, 81.0, 83.0, 87.0, 86.0, 73.0, 92.0, 93.0, 96.0, 90.0, 83.0, 75.0, 97.0, 92.0, 89.0, 93.0, 82.0, 83.0, 77.0, 81.0, 79.0, 78.0, 77.0, 68.0, 76.0, 92.0, 84.0, 96.0, 86.0, 87.0, 77.0, 85.0, 85.0, 82.0, 86.0, 97.0, 73.0, 72.0, 84.0, 65.0, 86.0, 64.0, 73.0, 70.0, 97.0, 74.0, 93.0, 86.0, 83.0, 88.0, 70.0, 76.0, 91.0, 79.0, 80.0, 84.0, 89.0, 78.0, 95.0, 94.0, 77.0, 75.0, 101.0, 93.0, 93.0, 83.0, 78.0, 70.0, 85.0, 78.0, 83.0]
  out "Off-Line Smoothed":dbl[](array[numeric])=[82.75690140845076, 81.55971830985922, 94.35901408450708, 116.56323943661974, 145.31676056338029, 180.99633802816902, 224.20760563380284, 276.24281690140845, 337.3730985915492, 406.00338028168994, 485.929436619718, 567.1160563380279, 638.4752112676053, 706.7428169014082, 767.3167605633801, 815.1547887323942, 819.5878873239435, 748.6407042253519, 624.7392957746476, 502.59140845070397, 423.1935211267604, 387.91887323943644, 374.90830985915477, 363.697042253521, 347.32028169014075, 326.01746478873235, 304.03507042253517, 285.04563380281684, 268.64774647887316, 255.55619718309862, 245.5597183098592, 232.48225352112678, 215.77450704225356, 200.05619718309862, 184.57028169014086, 172.20056338028166, 164.93295774647885, 159.60549295774643, 154.51042253521126, 147.50338028169017, 140.75338028169017, 136.2604225352113, 129.81323943661974, 119.82028169014086, 106.11605633802819, 92.86957746478876, 83.69704225352118, 77.96816901408455, 72.78154929577468, 66.42591549295777, 62.49633802816902, 58.947042253521126, 54.302676056338015, 52.31676056338027, 51.425915492957735, 49.30971830985914, 48.214647887323935, 46.42239436619717, 43.48577464788731, 40.74985915492957, 39.08788732394365, 37.07380281690139, 35.242816901408425, 35.34492957746477, 34.41183098591547, 31.950563380281675, 30.394225352112667, 30.006901408450698, 29.665352112676054, 28.88718309859155, 27.19352112676056, 25.228732394366197, 22.644225352112677, 21.415352112676054, 20.598450704225353, 19.99985915492958, 19.76042253521127, 19.13366197183099, 18.186478873239437, 17.05619718309859, 15.915352112676054, 15.503380281690138, 16.274507042253514, 15.813239436619712, 14.211126760563381, 13.651267605633805, 13.422394366197185, 13.182957746478875, 12.978732394366201, 11.749859154929577, 12.151267605633805, 12.28154929577465, 11.020985915492957, 11.207605633802817, 11.267464788732394, 9.848450704225352, 9.14774647887324, 9.809718309859155, 9.351971830985915, 8.65830985915493, 9.05267605633803, 8.616056338028171, 8.443521126760565, 8.665352112676057, 7.690000000000003, 7.337887323943664, 7.943521126760567, 6.475211267605637, 6.063239436619721, 6.799154929577467, 5.718169014084507, 6.190000000000001, 6.013943661971831, 4.869577464788733, 5.123098591549297, 5.848450704225353, 5.859014084507044, 4.989295774647888, 4.3061971830985915, 4.4540845070422534, 4.1336619718309855, 4.4857746478873235, 5.2569014084507035, 4.028028169014083, 3.7005633802816895, 4.154788732394366, 4.658309859154931, 4.489295774647888, 3.9716901408450704, 4.087887323943662, 3.5843661971830976, 3.3695774647887315, 3.9681690140845065, 3.3026760563380275, 3.1583098591549295, 3.8871830985915485, 2.901267605633801, 2.9928169014084487, 3.049154929577463, 2.3907042253521116, 2.5385915492957736, 2.9822535211267596, 2.587887323943661, 2.2780281690140836, 2.302676056338027, 2.9892957746478874, 3.218169014084507, 2.0808450704225345, 1.788591549295774, 1.894225352112675, 1.394225352112675, 0.7850704225352113, 1.0773239436619721, 0.9505633802816902, 1.1723943661971827, 1.5033802816901396, 1.3907042253521118, 2.0350704225352105, 1.964647887323943, 1.4576056338028163, 1.4892957746478865, 1.2146478873239435, 0.6371830985915494, 0.6794366197183093, 1.0632394366197175, 0.5385915492957744, 0.7533802816901405, 0.9540845070422534, 1.207605633802817, 1.6407042253521118, 1.3026760563380273, 0.6970422535211267, 0.3590140845070423, 0.8167605633802817, 0.968169014084507, 0.6301408450704226, 0.904788732394366, 1.0280281690140842, 0.7146478873239438, 0.9012676056338029, 0.8942253521126763, 0.9611267605633799, 1.1371830985915488, 0.5209859154929579, 0.5033802816901406, 1.133661971830985, 0.9892957746478871, 0.978732394366197, 1.0738028169014078, 0.7076056338028167, 1.0597183098591547, 1.2252112676056333, 0.7111267605633802, 0.7885915492957749, 0.6301408450704229, 0.8695774647887318, 0.5421126760563375, 0.792112676056338, 1.0984507042253522, 0.07732394366197216, 0.2569014084507045, 0.0033802816901409294, -0.01422535211267606, -0.02830985915492945, 0.1723943661971833, 0.6442253521126764, 0.3061971830985919, -0.4930985915492958, 0.042112676056337395, 1.2498591549295768, 0.6230985915492957, -0.17971830985915477, 0.013943661971830779, -0.40154929577464865, -0.6797183098591554, 0.4435211267605636, 0.4611267605633806, -0.1797183098591546, 0.3695774647887322, 1.1477464788732392, 1.0245070422535207, 0.3273239436619714, 0.4998591549295772, 1.0843661971830985, 0.43647887323943696, -0.3381690140845067, 0.27098591549295753, 0.3132394366197181, -0.23957746478873204, 0.7181690140845072, 0.0033802816901404853, -0.3769014084507043, 0.6900000000000002, 0.6407042253521129, 0.2850704225352114, -0.5564788732394367, -0.8980281690140846, -0.38042253521126745, -0.2607042253521126, -1.003661971830986, -0.8804225352112678, 0.46464788732394363, 0.9857746478873239, -0.31000000000000005, -0.7149295774647888, 0.16887323943661997, -0.09521126760563357, -0.18676056338028152, 0.15830985915493, 0.24985915492957794, -0.014225352112675824, 0.24985915492957775, 0.37661971830985946, -0.41915492957746514, -0.2747887323943666, 0.6794366197183099, 0.29563380281690155, -0.6233802816901406, 0.1371830985915493, 0.8378873239436619, 0.3026760563380284, -0.36633802816901384, -0.39450704225352085, 0.1371830985915496, 0.38366197183098616, 0.4223943661971833, 0.045633802816901575, -0.038873239436619536, -0.5283098591549295, -0.3733802816901407, 0.6266197183098594, -0.021267605633802533, -0.5388732394366197, -0.4966197183098592, -0.34169014084507027, -0.23957746478873215, 0.17239436619718307]
  out "On-Line  Smoothed":dbl[](array[numeric])=[70.56915492957748, 65.24169014084511, 69.9318309859155, 80.56915492957745, 93.81915492957748, 109.20647887323943, 126.53042253521124, 145.7733802816901, 167.8332394366197, 189.55154929577463, 211.40718309859156, 234.04802816901412, 251.38253521126774, 261.16422535211285, 267.17126760563394, 267.27690140845084, 252.61140845070435, 219.016338028169, 173.29802816901406, 133.53042253521124, 109.20647887323945, 95.5269014084507, 86.93535211267606, 81.82971830985915, 76.56915492957745, 68.79802816901409, 61.63253521126762, 56.25929577464788, 51.343802816901416, 47.29802816901409, 43.95647887323945, 40.002253521126775, 36.340281690140856, 33.41070422535211, 31.143098591549297, 28.60084507042254, 26.70647887323944, 25.63605633802817, 23.66774647887324, 22.893098591549297, 22.88253521126761, 21.597323943661973, 20.12549295774648, 17.660704225352113, 15.357887323943661, 13.403661971830985, 11.62549295774648, 11.442394366197185, 11.139577464788735, 9.893098591549299, 8.794507042253525, 8.301549295774649, 8.572676056338029, 7.773380281690141, 6.699436619718311, 6.942394366197185, 6.857887323943663, 7.195915492957749, 7.12549295774648, 6.692394366197185, 6.178309859154931, 5.467042253521125, 5.692394366197182, 5.445915492957745, 4.967042253521125, 4.977605633802815, 5.146619718309859, 4.815633802816902, 4.843802816901409, 4.533943661971831, 3.185352112676056, 3.234647887323943, 3.4107042253521125, 3.442394366197183, 3.653661971830986, 3.3895774647887316, 3.0656338028169, 2.688873239436619, 2.030422535211267, 1.688873239436619, 2.160704225352111, 2.459999999999999, 2.8578873239436615, 2.75225352112676, 2.350845070422535, 1.6994366197183095, 1.78394366197183, 2.667746478873238, 2.2029577464788725, 1.97056338028169, 1.9001408450704225, 1.6607042253521123, 1.1571830985915486, 1.3473239436619717, 1.7522535211267605, 1.2733802816901405, 1.2170422535211263, 0.8578873239436615, 0.7205633802816898, 1.5550704225352106, 2.192394366197182, 1.484647887323943, 1.1184507042253515, 0.854366197183098, 0.3649295774647884, 1.0057746478873242, 1.3860563380281692, 0.9107042253521123, 0.776901408450704, 1.048028169014084, 1.2487323943661965, 0.7804225352112671, 0.9107042253521123, 0.9423943661971828, -0.2266197183098595, -0.184366197183099, 0.7170422535211262, 1.0092957746478868, 0.9776056338028167, 0.7346478873239435, 0.555070422535211, 1.0515492957746475, 0.16774647887323924, -0.3604225352112679, 1.0621126760563375, 0.9529577464788728, 0.7874647887323939, 0.8966197183098586, 0.5691549295774644, 0.5198591549295771, 0.31915492957746444, 0.47056338028168976, 0.8050704225352108, 0.5867605633802813, 0.343802816901408, 0.9811267605633798, 1.0691549295774643, 0.7205633802816898, 1.1783098591549293, 0.8121126760563376, 0.04450704225352073, -0.2407042253521131, 0.1923943661971826, 0.13253521126760515, 0.16422535211267586, 0.2416901408450702, -0.5223943661971835, -0.0857746478873243, 0.6642253521126757, 0.47408450704225313, -0.02943661971831026, 0.0022535211267601662, 0.09028169014084472, 0.287464788732394, 0.25577464788732357, 0.19239436619718267, 0.28042253521126725, 0.5339436619718307, 0.31211267605633786, -0.03647887323943691, 0.6747887323943658, 0.9740845070422529, 0.5128169014084502, 1.0092957746478866, 0.5339436619718301, -0.1139436619718314, 0.2909859154929573, -0.25478873239436667, 0.13605633802816863, 1.0797183098591545, 0.6466197183098586, -0.23366197183098641, -0.05408450704225401, 0.30859154929577426, 0.9987323943661965, 1.4776056338028165, 1.0550704225352112, 0.6501408450704222, 0.7205633802816899, 0.7557746478873236, 0.48464788732394315, 0.2804225352112671, 0.13957746478873195, 0.0585915492957741, 0.1290140845070417, 0.3930985915492954, 0.49169014084507, 0.09380281690140801, 0.0022535211267601107, 0.269859154929577, -0.040000000000000424, -0.3780281690140849, -0.4871830985915497, -0.08929577464788782, 0.03746478873239388, 0.18183098591549218, 0.301549295774647, -0.24070422535211314, -0.17732394366197224, 0.2452112676056334, 0.23112676056337994, -0.061126760563380664, 0.298028169014084, 0.6430985915492953, 0.9635211267605631, 0.6149295774647885, -0.5716901408450707, -0.24774647887323983, -0.33577464788732414, -0.9590140845070425, -0.7336619718309862, -0.38507042253521157, -0.21605633802816943, 0.3121126760563376, 0.945915492957746, 0.2487323943661967, -0.3674647887323948, -0.10690140845070463, -0.24774647887323975, -0.6069014084507046, -0.01887323943662017, 0.2839436619718306, 0.016338028169013682, 0.14309859154929536, 0.10788732394366163, -0.5259154929577468, -0.5576056338028172, -0.11394366197183144, -0.02591549295774695, 0.4283098591549292, -0.17732394366197202, -1.2477464788732395, -0.740704225352113, 0.07267605633802769, 0.17830985915492906, -0.21957746478873302, -0.606901408450705, -0.31816901408450765, -0.5223943661971837, -0.36042253521126827, 0.621971830985915, 0.6254929577464784, 0.16774647887323899, -0.03295774647887369, -0.6209859154929581, -0.33929577464788774, 0.769859154929577, 0.371971830985915, -0.589295774647888, -0.5400000000000007, -0.20901408450704279, -0.5963380281690146, -0.49774647887323986, -0.34281690140845106, 0.3578873239436618, 0.3790140845070421, 0.15718309859154894, 0.713521126760563, 0.5269014084507038, 0.06563380281690101, -0.5928169014084512, -0.1350704225352118, 0.5269014084507038, -0.23366197183098636, -0.9449295774647892, -0.17380281690140897, 0.15718309859154886, -0.4484507042253525, -0.43084507042253556, 0.7769014084507038, 1.065633802816901, 0.6325352112676053, 0.05154929577464751, -0.3709859154929582, 0.01633802816901366, -0.004788732394366599, -0.43788732394366237]
  out "On-Line Bin Readings":dbl[](array[numeric])=[179.0, 138.0, 160.0, 161.0, 181.0, 186.0, 206.0, 221.0, 249.0, 254.0, 284.0, 295.0, 320.0, 360.0, 330.0, 383.0, 401.0, 404.0, 342.0, 265.0, 209.0, 164.0, 180.0, 174.0, 153.0, 149.0, 141.0, 144.0, 153.0, 154.0, 120.0, 135.0, 137.0, 117.0, 113.0, 118.0, 126.0, 115.0, 117.0, 95.0, 110.0, 128.0, 75.0, 104.0, 100.0, 95.0, 93.0, 101.0, 94.0, 93.0, 89.0, 90.0, 92.0, 85.0, 94.0, 87.0, 75.0, 81.0, 79.0, 118.0, 83.0, 97.0, 96.0, 91.0, 97.0, 83.0, 91.0, 78.0, 95.0, 100.0, 94.0, 69.0, 87.0, 93.0, 85.0, 100.0, 68.0, 88.0, 71.0, 85.0, 70.0, 84.0, 77.0, 100.0, 95.0, 87.0, 74.0, 99.0, 96.0, 76.0, 73.0, 84.0, 85.0, 81.0, 83.0, 89.0, 70.0, 86.0, 89.0, 91.0, 74.0, 97.0, 85.0, 81.0, 71.0, 70.0, 78.0, 80.0, 80.0, 89.0, 91.0, 84.0, 88.0, 85.0, 84.0, 76.0, 105.0, 88.0, 86.0, 93.0, 83.0, 78.0, 91.0, 97.0, 101.0, 86.0, 81.0, 84.0, 82.0, 88.0, 82.0, 85.0, 79.0, 77.0, 87.0, 87.0, 66.0, 99.0, 72.0, 80.0, 84.0, 93.0, 85.0, 80.0, 75.0, 67.0, 85.0, 76.0, 76.0, 93.0, 89.0, 80.0, 84.0, 81.0, 97.0, 85.0, 79.0, 74.0, 83.0, 99.0, 84.0, 75.0, 96.0, 96.0, 97.0, 101.0, 89.0, 89.0, 75.0, 85.0, 87.0, 77.0, 86.0, 79.0, 94.0, 76.0, 91.0, 80.0, 72.0, 92.0, 102.0, 104.0, 96.0, 84.0, 85.0, 94.0, 84.0, 88.0, 82.0, 64.0, 75.0, 79.0, 91.0, 97.0, 93.0, 77.0, 81.0, 81.0, 72.0, 80.0, 86.0, 76.0, 89.0, 95.0, 90.0, 82.0, 72.0, 72.0, 79.0, 93.0, 93.0, 88.0, 83.0, 70.0, 89.0, 92.0, 80.0, 84.0, 76.0, 96.0, 72.0, 64.0, 74.0, 88.0, 81.0, 77.0, 83.0, 80.0, 87.0, 84.0, 83.0, 85.0, 66.0, 90.0, 84.0, 82.0, 81.0, 88.0, 94.0, 89.0, 74.0, 82.0, 86.0, 88.0, 87.0, 88.0, 85.0, 91.0, 100.0, 77.0, 87.0, 88.0, 74.0, 83.0, 85.0, 90.0, 87.0, 73.0, 83.0, 67.0, 87.0, 95.0, 81.0, 81.0, 81.0, 86.0, 72.0, 82.0, 75.0, 76.0, 99.0, 63.0, 94.0, 91.0, 82.0, 83.0, 96.0, 90.0, 71.0]
  out "Range Corrected Altitude Array":dbl[](array[numeric])=[5625.0, 22500.0, 50625.0, 90000.0, 140625.0, 202500.0, 275625.0, 360000.0, 455625.0, 562500.0, 680625.0, 810000.0, 950625.0, 1102500.0, 1265625.0, 1440000.0, 1625625.0, 1822500.0, 2030625.0, 2250000.0, 2480625.0, 2722500.0, 2975625.0, 3240000.0, 3515625.0, 3802500.0, 4100625.0, 4410000.0, 4730625.0, 5062500.0, 5405625.0, 5760000.0, 6125625.0, 6502500.0, 6890625.0, 7290000.0, 7700625.0, 8122500.0, 8555625.0, 9000000.0, 9455625.0, 9922500.0, 10400625.0, 10890000.0, 11390625.0, 11902500.0, 12425625.0, 12960000.0, 13505625.0, 14062500.0, 14630625.0, 15210000.0, 15800625.0, 16402500.0, 17015625.0, 17640000.0, 18275625.0, 18922500.0, 19580625.0, 20250000.0, 20930625.0, 21622500.0, 22325625.0, 23040000.0, 23765625.0, 24502500.0, 25250625.0, 26010000.0, 26780625.0, 27562500.0, 28355625.0, 29160000.0, 29975625.0, 30802500.0, 31640625.0, 32490000.0, 33350625.0, 34222500.0, 35105625.0, 36000000.0, 36905625.0, 37822500.0, 38750625.0, 39690000.0, 40640625.0, 41602500.0, 42575625.0, 43560000.0, 44555625.0, 45562500.0, 46580625.0, 47610000.0, 48650625.0, 49702500.0, 50765625.0, 51840000.0, 52925625.0, 54022500.0, 55130625.0, 56250000.0, 57380625.0, 58522500.0, 59675625.0, 60840000.0, 62015625.0, 63202500.0, 64400625.0, 65610000.0, 66830625.0, 68062500.0, 69305625.0, 70560000.0, 71825625.0, 73102500.0, 74390625.0, 75690000.0, 77000625.0, 78322500.0, 79655625.0, 81000000.0, 82355625.0, 83722500.0, 85100625.0, 86490000.0, 87890625.0, 89302500.0, 90725625.0, 92160000.0, 93605625.0, 95062500.0, 96530625.0, 98010000.0, 99500625.0, 101002500.0, 102515625.0, 104040000.0, 105575625.0, 107122500.0, 108680625.0, 110250000.0, 111830625.0, 113422500.0, 115025625.0, 116640000.0, 118265625.0, 119902500.0, 121550625.0, 123210000.0, 124880625.0, 126562500.0, 128255625.0, 129960000.0, 131675625.0, 133402500.0, 135140625.0, 136890000.0, 138650625.0, 140422500.0, 142205625.0, 144000000.0, 145805625.0, 147622500.0, 149450625.0, 151290000.0, 153140625.0, 155002500.0, 156875625.0, 158760000.0, 160655625.0, 162562500.0, 164480625.0, 166410000.0, 168350625.0, 170302500.0, 172265625.0, 174240000.0, 176225625.0, 178222500.0, 180230625.0, 182250000.0, 184280625.0, 186322500.0, 188375625.0, 190440000.0, 192515625.0, 194602500.0, 196700625.0, 198810000.0, 200930625.0, 203062500.0, 205205625.0, 207360000.0, 209525625.0, 211702500.0, 213890625.0, 216090000.0, 218300625.0, 220522500.0, 222755625.0, 225000000.0, 227255625.0, 229522500.0, 231800625.0, 234090000.0, 236390625.0, 238702500.0, 241025625.0, 243360000.0, 245705625.0, 248062500.0, 250430625.0, 252810000.0, 255200625.0, 257602500.0, 260015625.0, 262440000.0, 264875625.0, 267322500.0, 269780625.0, 272250000.0, 274730625.0, 277222500.0, 279725625.0, 282240000.0, 284765625.0, 287302500.0, 289850625.0, 292410000.0, 294980625.0, 297562500.0, 300155625.0, 302760000.0, 305375625.0, 308002500.0, 310640625.0, 313290000.0, 315950625.0, 318622500.0, 321305625.0, 324000000.0, 326705625.0, 329422500.0, 332150625.0, 334890000.0, 337640625.0, 340402500.0, 343175625.0, 345960000.0, 348755625.0, 351562500.0, 354380625.0, 357210000.0, 360050625.0, 362902500.0, 365765625.0, 368640000.0, 371525625.0, 374422500.0, 377330625.0, 380250000.0, 383180625.0, 386122500.0, 389075625.0, 392040000.0, 395015625.0, 398002500.0, 401000625.0, 404010000.0, 407030625.0, 410062500.0, 413105625.0, 416160000.0, 419225625.0, 422302500.0, 425390625.0, 428490000.0, 431600625.0, 434722500.0, 437855625.0, 441000000.0]
  out "Altitude Array (km)":dbl[](array[numeric])=[0.075, 0.15, 0.22499999999999998, 0.3, 0.375, 0.45, 0.5249999999999999, 0.6, 0.6749999999999999, 0.7499999999999999, 0.825, 0.8999999999999999, 0.9749999999999999, 1.05, 1.125, 1.2, 1.275, 1.3499999999999999, 1.4249999999999998, 1.5, 1.575, 1.65, 1.7249999999999999, 1.7999999999999998, 1.8749999999999998, 1.95, 2.025, 2.1, 2.1750000000000003, 2.25, 2.325, 2.4, 2.475, 2.5500000000000003, 2.625, 2.7, 2.775, 2.85, 2.9250000000000003, 3.0, 3.075, 3.15, 3.225, 3.3000000000000003, 3.375, 3.45, 3.525, 3.6, 3.675, 3.75, 3.825, 3.9, 3.975, 4.05, 4.125, 4.2, 4.275, 4.35, 4.425, 4.5, 4.575, 4.65, 4.725, 4.8, 4.875, 4.95, 5.025, 5.1, 5.175, 5.25, 5.325, 5.4, 5.475, 5.55, 5.625, 5.7, 5.775, 5.85, 5.925, 6.0, 6.075, 6.15, 6.225, 6.3, 6.375, 6.45, 6.525, 6.6, 6.675, 6.75, 6.825, 6.9, 6.975, 7.05, 7.125, 7.2, 7.2749999999999995, 7.35, 7.425, 7.5, 7.575, 7.6499999999999995, 7.725, 7.8, 7.875, 7.95, 8.024999999999999, 8.1, 8.174999999999999, 8.249999999999998, 8.325, 8.399999999999999, 8.475, 8.549999999999999, 8.624999999999998, 8.7, 8.774999999999999, 8.85, 8.924999999999999, 8.999999999999998, 9.075, 9.149999999999999, 9.225, 9.299999999999999, 9.374999999999998, 9.45, 9.524999999999999, 9.6, 9.674999999999999, 9.749999999999998, 9.825, 9.899999999999999, 9.975, 10.049999999999999, 10.124999999999998, 10.2, 10.274999999999999, 10.35, 10.424999999999999, 10.499999999999998, 10.575, 10.649999999999999, 10.725, 10.799999999999999, 10.874999999999998, 10.95, 11.024999999999999, 11.1, 11.174999999999999, 11.249999999999998, 11.325, 11.399999999999999, 11.475, 11.549999999999999, 11.624999999999998, 11.7, 11.774999999999999, 11.85, 11.924999999999999, 11.999999999999998, 12.075, 12.149999999999999, 12.225, 12.299999999999999, 12.374999999999998, 12.45, 12.524999999999999, 12.6, 12.674999999999999, 12.749999999999998, 12.825, 12.899999999999999, 12.975, 13.049999999999999, 13.124999999999998, 13.2, 13.274999999999999, 13.35, 13.424999999999999, 13.499999999999998, 13.575, 13.649999999999999, 13.725, 13.799999999999999, 13.874999999999998, 13.95, 14.024999999999999, 14.1, 14.174999999999999, 14.249999999999998, 14.325, 14.399999999999999, 14.474999999999998, 14.549999999999999, 14.624999999999998, 14.7, 14.774999999999999, 14.849999999999998, 14.924999999999999, 14.999999999999998, 15.075, 15.149999999999999, 15.224999999999998, 15.299999999999999, 15.374999999999998, 15.45, 15.524999999999999, 15.599999999999998, 15.674999999999999, 15.749999999999998, 15.825, 15.899999999999999, 15.974999999999998, 16.05, 16.125, 16.2, 16.275, 16.349999999999998, 16.424999999999997, 16.5, 16.575, 16.65, 16.724999999999998, 16.799999999999997, 16.875, 16.95, 17.025, 17.099999999999998, 17.174999999999997, 17.25, 17.325, 17.4, 17.474999999999998, 17.549999999999997, 17.625, 17.7, 17.775, 17.849999999999998, 17.924999999999997, 18.0, 18.075, 18.15, 18.224999999999998, 18.299999999999997, 18.375, 18.45, 18.525, 18.599999999999998, 18.674999999999997, 18.75, 18.825, 18.9, 18.974999999999998, 19.049999999999997, 19.125, 19.2, 19.275, 19.349999999999998, 19.424999999999997, 19.5, 19.575, 19.65, 19.724999999999998, 19.799999999999997, 19.875, 19.95, 20.025, 20.099999999999998, 20.174999999999997, 20.25, 20.325, 20.4, 20.474999999999998, 20.549999999999997, 20.625, 20.7, 20.775, 20.849999999999998, 20.924999999999997, 21.0]
  out "Offline Pulse Energy":dbl=4.4057514285714285
  out "Online Pulse Energy":dbl=4.393014285714285
  in  "Instrument Control":T5(tab)
  out "Readings":T6={"OnLineTEC"=23.2349491, "OnLineLD"=0.172291026, "OffLineTEC"=29.5197392, "OffLineLD"=0.173082039, "EtalonTEC"=29.3232155, "TSOA-TEC"=19.0029545, "Pro8000"=TRUE, "OnLine TEC"=TRUE, "OnLine LD"=TRUE, "OffLine TEC"=TRUE, "OffLine LD"=TRUE, "Etalon TEC"=TRUE, "TSOA TEC"=TRUE} {"OffLineLD" format="%.4g"; "OnLineLD" format="%.4g"; "TSOA-TEC" format="%.3g"; "EtalonTEC" format="%.3g"; "OffLineTEC" format="%.3g"; "OnLineTEC" format="%.3g"}
  in  "Settings":T7={"Module"=enum."On Line TEC", "OnLineTEC"=23.228899999999935, "OnLineLD"=0.1722, "OffLineTEC"=29.506199999999676, "OffLineLD"=0.173, "EtalonTEC"=29.0, "TSOA-TEC"=19.0} {"OffLineLD" min=0.0 max=0.175 step=0.001 format="%.3p"; "OnLineLD" min=0.0 max=0.175 step=0.001 format="%.3p"; "TSOA-TEC" format="%.2g"; "EtalonTEC" format="%.2g"; "OffLineTEC" min=0.0 max=30.0 step=0.1 format="%.3g"; "OnLineTEC" min=0.0 max=30.0 step=0.1 format="%.3g"}
  in  "Device In":refnum<visa-resource-name>="Pro8000"
  in  "Pulse B Polarity":enum32{"Low", "High"}(ring)=enum."High"
  in  "Pulse A Delay(ns)":u32=1040 min=80 max=327600
  in  "Pulse B Delay(ns)":u32=170000 min=80 max=327600 step=1
  in  "Accumulation Delay(ns)":u32=10 min=10 max=1270 step=1
  in  "Sync Pulse Polarity":enum32{"Low", "High"}(ring)=enum."High"
  in  "Pulse A Polarity":enum32{"Low", "High"}(ring)=enum."High"
  in  "Number of Bins":u32=280 min=2 max=4095 step=1
  in  "Number of Accumulates":u32=10000 min=1 max=32767 step=1
  in  "Time Resolution Per Bin(ns)":u32=500 min=5 max=1063 step=1
  out "AMCS_Profile":i32=725
  in  "Lambda On Set (nm)":dbl=828.194 format="%.5f"
  out "Lambda On Read (nm)":dbl=828.1940001302195 format="%.5f"
  out "Lambda Off Read (nm)":dbl=828.2934849374717 format="%.5f"
  in  "Lambda Off Set (nm)":dbl=828.29345 format="%#.5f"
  in  "Bristol In":i32=5
  out "Bristol Out":i32
  out "WL_Difference":dbl=1.302195187236066e-07 format="%#_3e"
  out "WL Difference off":dbl=3.4937471696139255e-05 format="%#_3e"
  out "Wavelength Lock Online":bool=TRUE
  out "Wavelength Lock Offline":bool=TRUE
  in  "calculate absorption cross sections":bool
  in  "Online_Tol":dbl=5e-05 format="%#_15g"
  in  "Cancel online":bool
  in  "Offline_Tol":dbl=0.0001 format="%#_15g"
  in  "Cancel Offline":bool
  in  "y":dbl=0.00025 format="%#_6p"
  in  "Smoothing Range":dbl=150.0
  in  "Total DIAL Integration Time (Minutes)":i32=3
  in  "Data Reads (number of loops)":i32=1
  in  "Total Aerosol Integration Time (Minutes)":dbl=0.5
  in  "Scalar Wait Time":u32
  out "Smoothed Bins":dbl=2.0
  in  "NewportIn":string
  in  "logging":bool
  out "Newport Device Key":string="1918-R 15120"
  in  "SampleSize":i32=2
  out "NewportRef":refnum<k24>
  in  "Switch Comm Port":refnum<visa-resource-name>="COM3"
  out "FF_On_Ref":refnum<file>
  out "FF_On_Ptr":i64=164736 format="%.2p"
  out "FF_Off_Ref":refnum<file>
  out "FF_Off_Ptr":i64=164736 format="%.2p"
  out "NF_On_Ref":refnum<file>
  out "NF_On_Ptr":i64=164736 format="%.2p"
  out "NF_Off_Ref":refnum<file>
  out "NF_Off_Ptr":i64=164736 format="%.2p"
  out "DataOpen":bool=TRUE
  out "File Path_Far Field (out)":string="C:\\Users\\H2ODial\\Desktop\\SharedTeleWVData\\161102FF\\21"
  out "File Path_Near Field (out)":string="C:\\Users\\H2ODial\\Desktop\\SharedTeleWVData\\161102NF\\21"
  in  "Data File DIR (in)":string="C:\\Users\\H2ODial\\Desktop\\SharedTeleWVData\\"
  out "TRHP":T8={"Temp C"=15.103479853479854, "RelH %"=39.287240537240535, "Press hPa"=844.848901098901, "AbH g/m^3"=4.945054945054945}
  in  "WS visa":refnum<visa-resource-name>="LuftWS"
  in  "WS_On/Off":bool=TRUE
  in  "bins":u32=280 min=2 max=4095 step=1
  out "y offset":u32=10
  in  "ns scale":u32=500
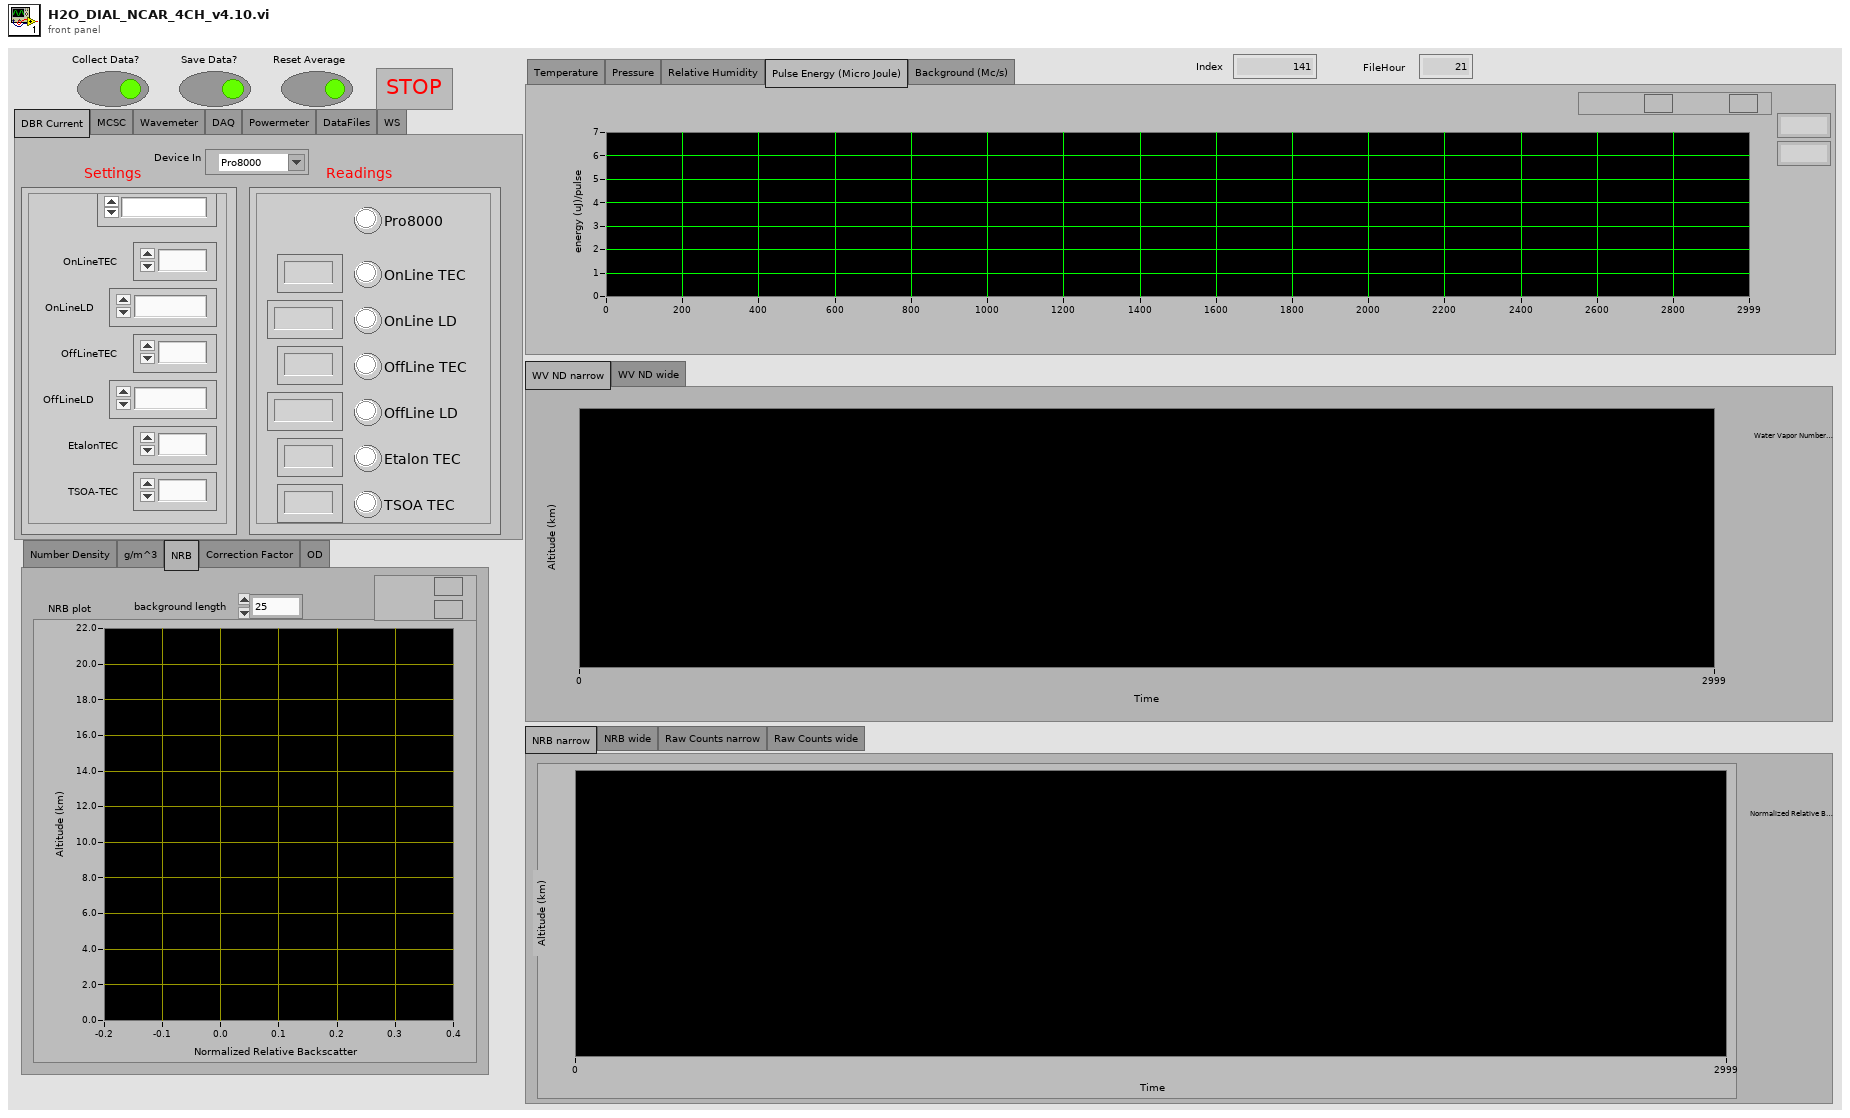
[diagram p1: front panel]
types:
  T1 = enum32{"NRB narrow", "NRB wide", "Raw Counts narrow", "Raw Counts wide"}
  T2 = enum32{"Number Density", "g/m^3", "NRB", "Correction Factor", "OD"}
  T3 = enum32{"Temperature", "Pressure", "Relative Humidity", "Pulse Energy (Micro Joule)", "Background (Mc/s)"}
  T4 = cluster{"Online Pulse Energy":dbl, "Pulse Energy Offline":dbl}
  T5 = enum32{"DBR Current", "MCSC", "Wavemeter", "DAQ", "Powermeter", "DataFiles", "WS"}
  T6 = cluster{"OnLineTEC":dbl, "OnLineLD":dbl, "OffLineTEC":dbl, "OffLineLD":dbl, "EtalonTEC":dbl, "TSOA-TEC":dbl, "Pro8000":bool, "OnLine TEC":bool, "OnLine LD":bool, "OffLine TEC":bool, "OffLine LD":bool, "Etalon TEC":bool, "TSOA TEC":bool}
  T7 = cluster{"Module":enum16{"On Line TEC", "On Line LD", "Off Line TEC", "Off Line LD", "Etalon TEC", "TSOA TEC"}, "OnLineTEC":dbl, "OnLineLD":dbl, "OffLineTEC":dbl, "OffLineLD":dbl, "EtalonTEC":dbl, "TSOA-TEC":dbl}
  T8 = cluster{"Temp C":dbl, "RelH %":dbl, "Press hPa":dbl, "AbH g/m^3":dbl}
  T9 = enum16{"Open_TL", "Close_TL", "Verify_ID", "TEC_Sensor", "SET", "READ", "ON", "OFF", "Set_Limits", "Read_Limits", "Enable_Status", "Read_Status"}
  T10 = enum16{"Initialize ILX", "Set ON T", "Set Off T", "Set ON I", "Set Off I", "Set On Lim", "Set Off Lim", "Read ILX", "TEC ON/OFF", "LASER ON/OFF", "Status?", "ILX OFF"}
  T11 = enum16{"open", "replace", "create", "open or create", "replace or create", "replace or create with confirmation"}
  T12 = enum16{"On Line TEC", "On Line LD", "Off Line TEC", "Off Line LD", "Etalon TEC", "TSOA TEC"}
  T13 = cluster{"Temp":dbl, "RelH":dbl, "Press":dbl, "AbH":dbl}
  T14 = typedef "LVDateTimeRec.ctl" = cluster{"fractional second":dbl, "second":i32, "minute":i32, "hour":i32, "day of month":i32, "month":i32, "year":i32, "day of week":i32, "day of year":i32, "DST":i32}
  T15 = cluster{"Online Pulse Energy":dbl, "Offline Pulse Energy":dbl}
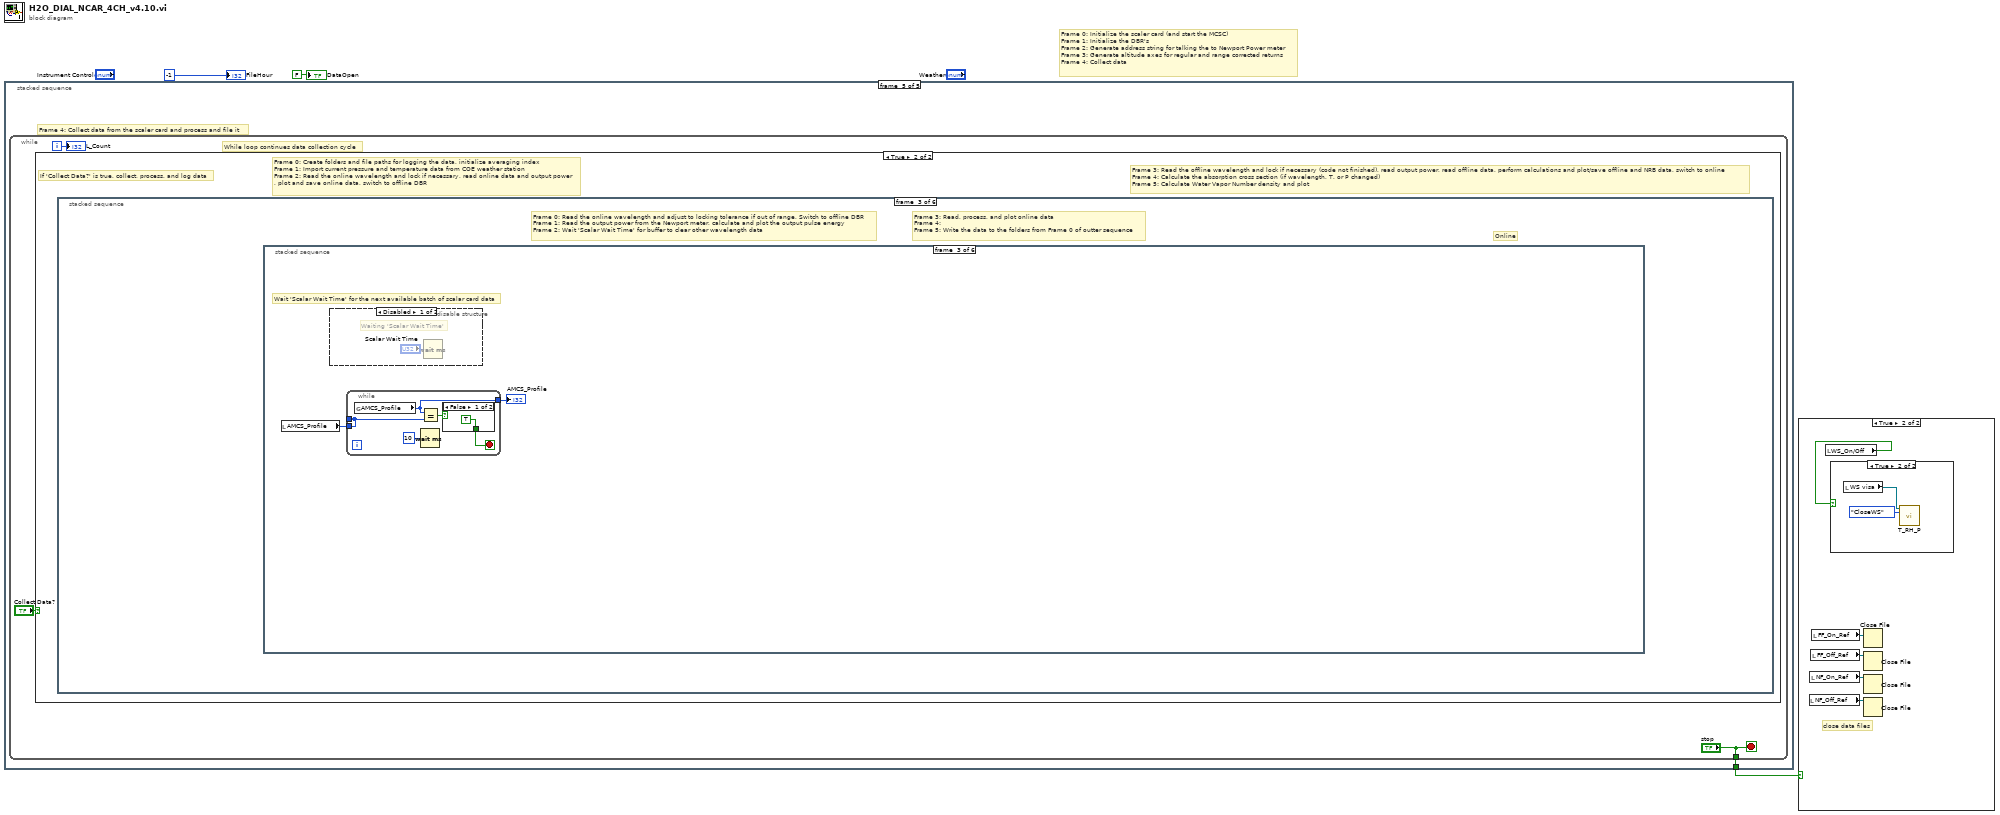
[diagram p0: block diagram]
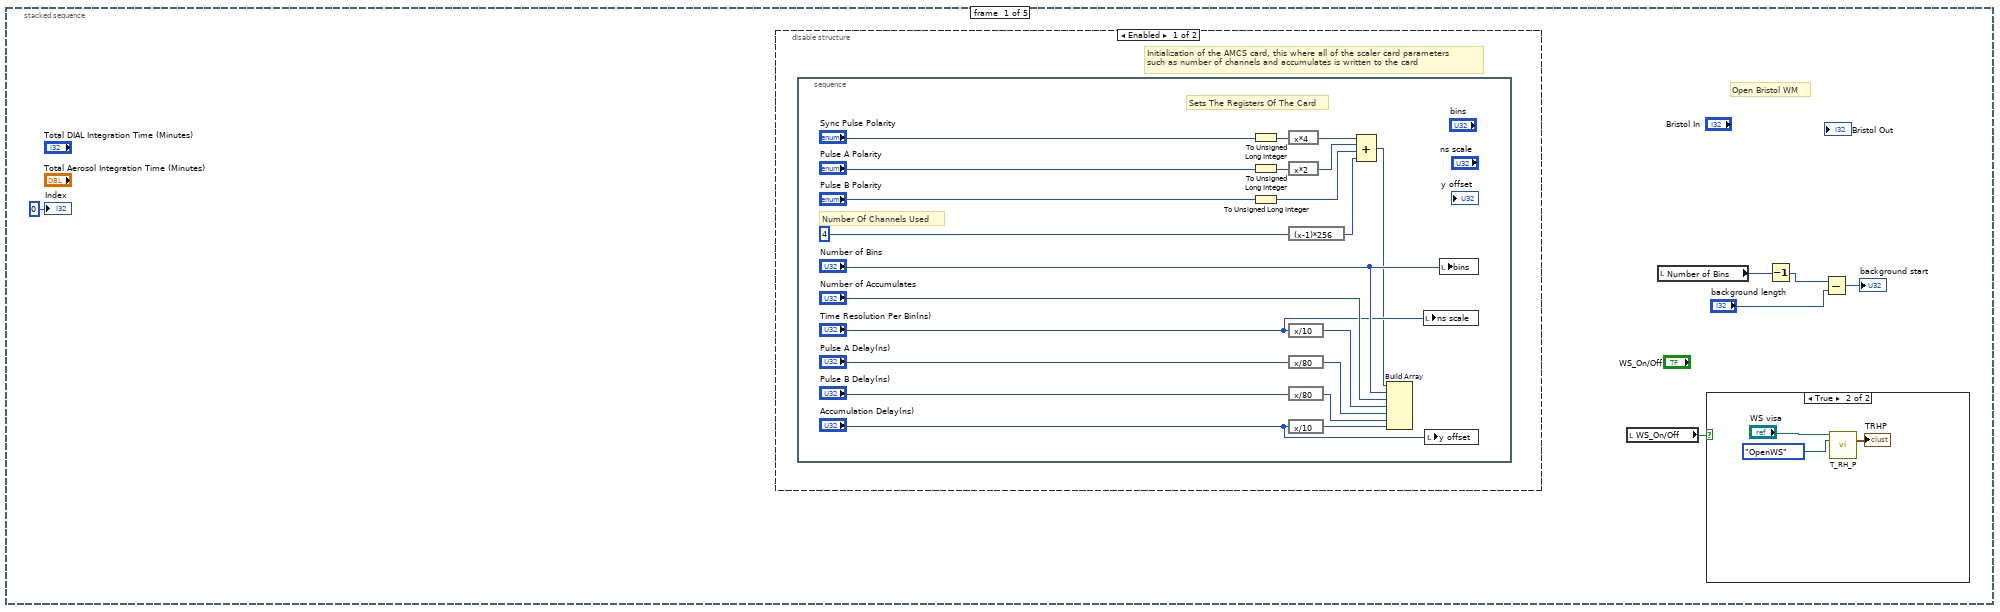
[diagram p4: hidden frame]
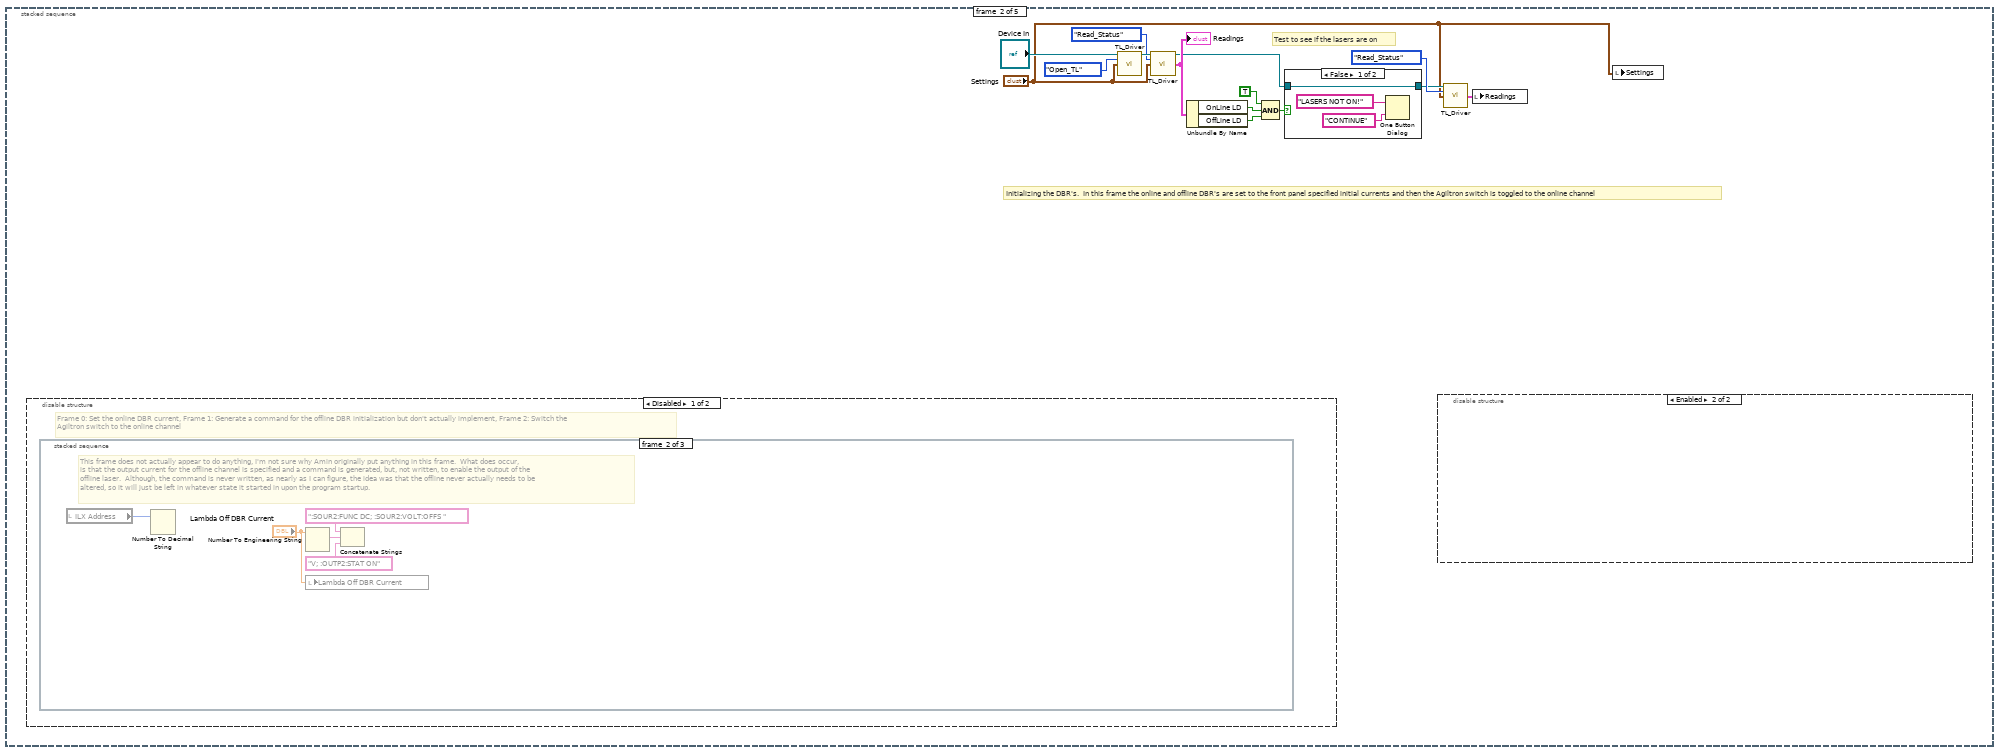
[diagram p7: hidden frame]
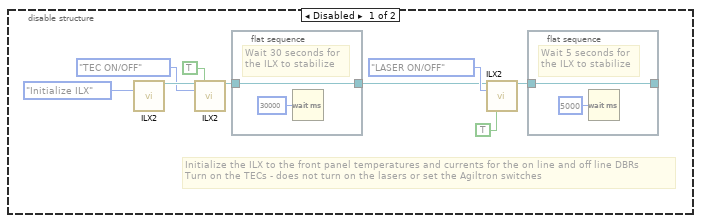
[diagram p9: hidden frame]
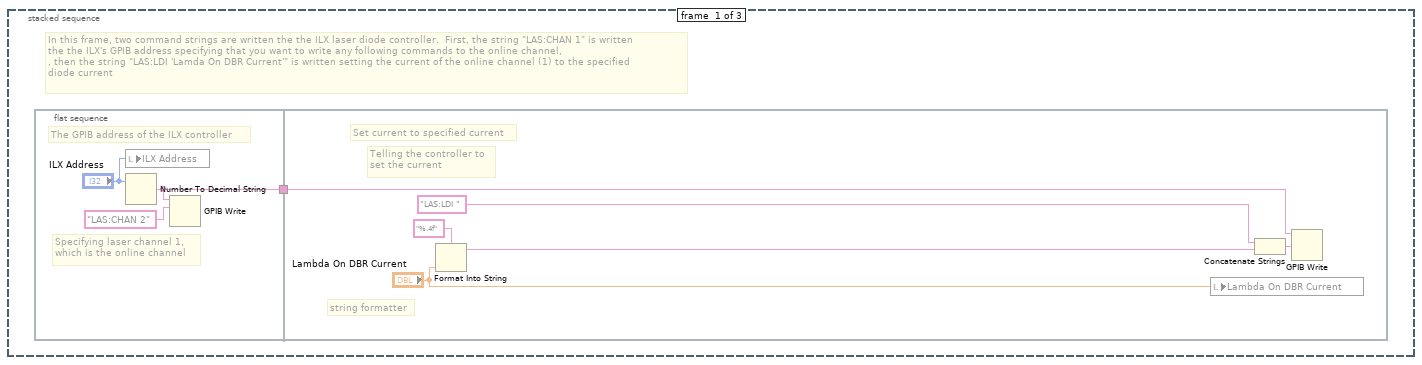
[diagram p10: hidden frame]
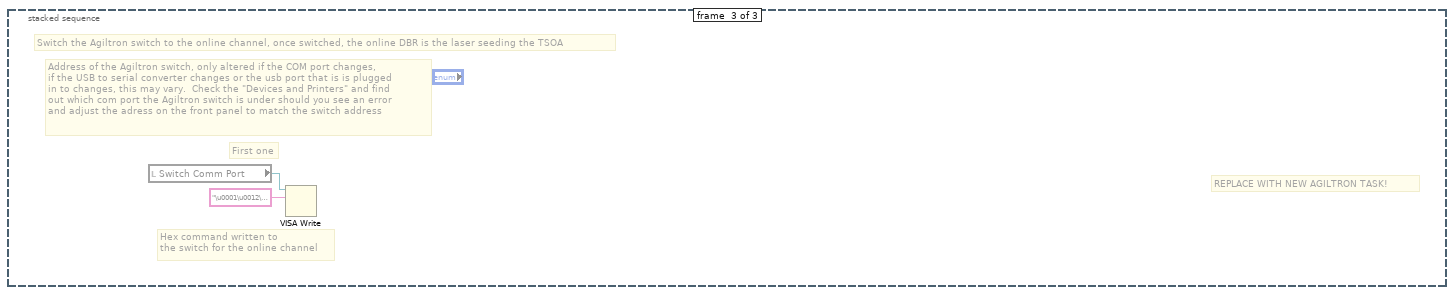
[diagram p11: hidden frame]
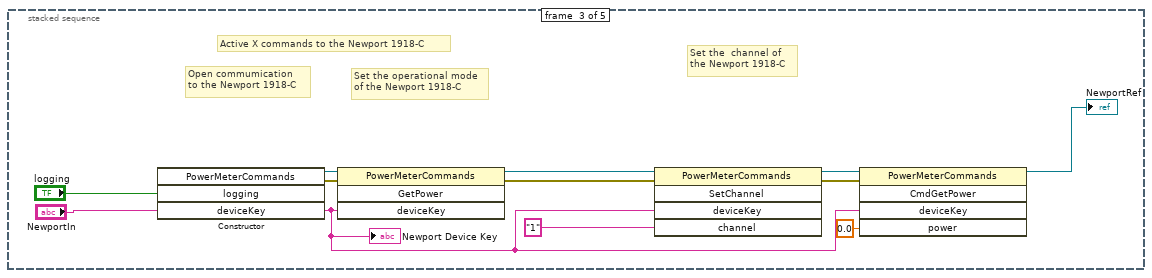
[diagram p13: hidden frame]
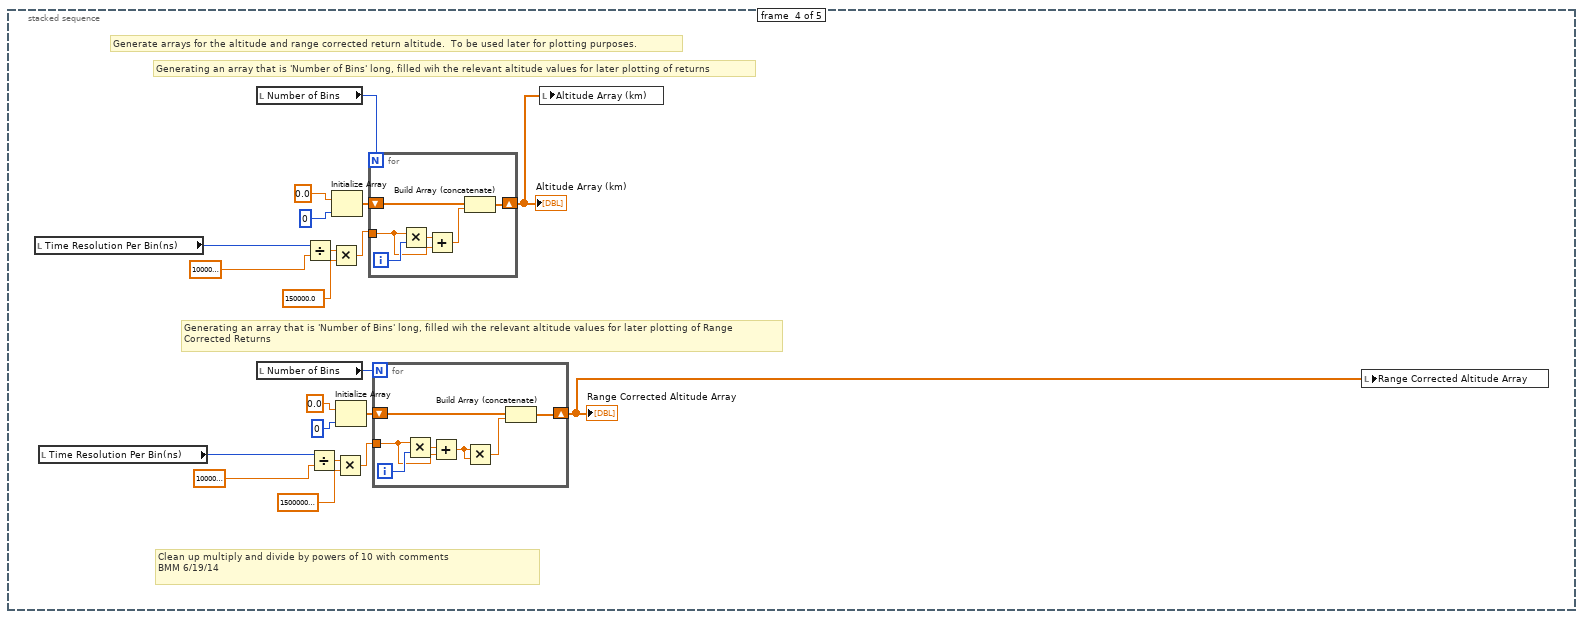
[diagram p14: hidden frame]
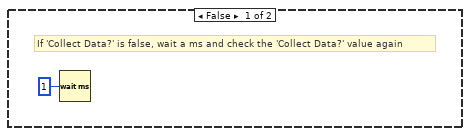
[diagram p15: hidden frame]
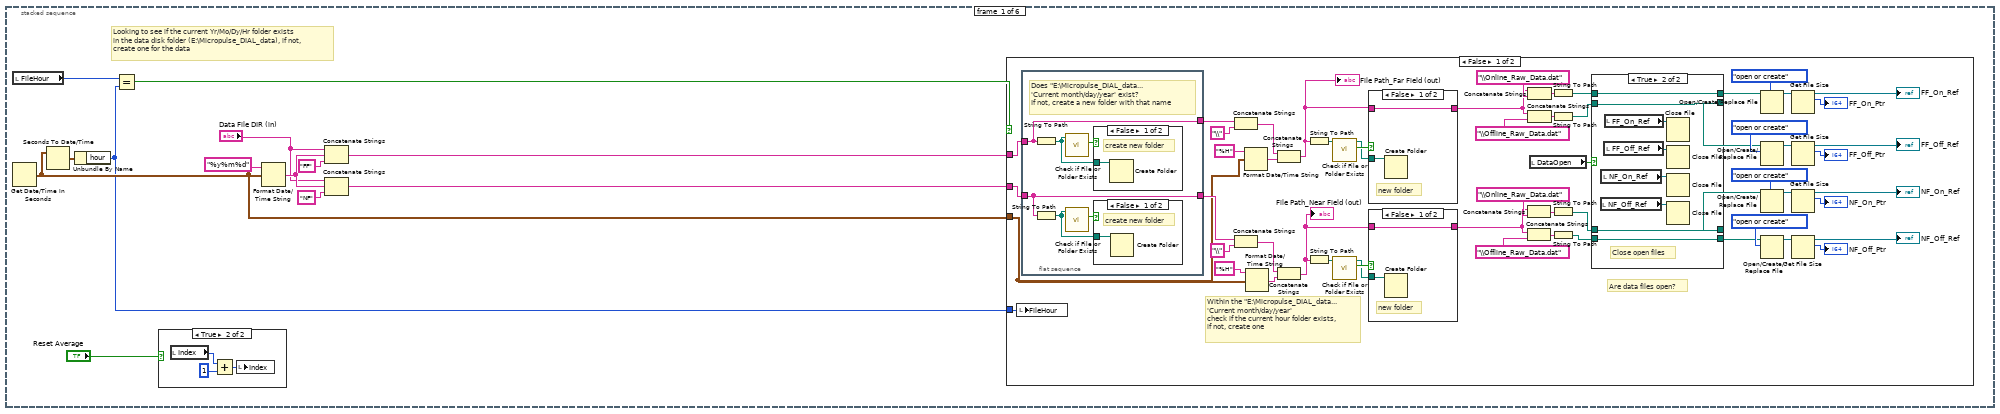
[diagram p16: hidden frame]
diagram:
  # "Frame 0: Initialize the scaler card (and start the MCSC)\nFrame 1: Initialize the DBR's\nFrame 2: Generate address string for talking the to Newport Power meter\nFrame 3: Generate altitude axes for regular and range corrected returns\nFrame 4: Collect data"
  n1 = stacked-sequence {
    tunnel: [_ _ _ _ w127] -> w3
    frame #0 {
      # "Open Bristol WM"
      n2 = disable-structure shown="Enabled" {
        frame Enabled {
          # "Initialization of the AMCS card, this where all of the scaler card parameters\nsuch as number of channels and accumulates is written to the card"
          n3 = stacked-sequence {
            frame #0 {
              # "Sets The Registers Of The Card"
              # "Number Of Channels Used"
              n4 = To Unsigned Long Integer(number="Sync Pulse Polarity") -> (unsigned 32bit integer=w13:u32)
              n5 = To Unsigned Long Integer(number="Pulse A Polarity") -> (unsigned 32bit integer=w17:u32)
              n6 = To Unsigned Long Integer(number="Pulse B Polarity") -> (unsigned 32bit integer=w15:u32)
              n7 = expression code="x*4"(w13) -> (w22:u32)
              n8 = expression code="x*2"(w17) -> (w21:u32)
              n9 = expression code="(x-1)*256"(u32 4 ("Number of Channels Used")) -> (w20:u32)
              n10 = expression code="x/10"("Time Resolution Per Bin(ns)") -> (w24:u32)
              n11 = expression code="x/80"("Pulse A Delay(ns)") -> (w31:u32)
              n12 = expression code="x/80"("Pulse B Delay(ns)") -> (w33:u32)
              n13 = expression code="x/10"("Accumulation Delay(ns)") -> (w32:u32)
              n14 = Compound Arithmetic op=ADD(w22, w21, w15, w20) -> (w19:u32)
              n15 = Build Array(w19, "Number of Bins", "Number of Accumulates", w24, w31, w33, w32) -> ()  [unwired: 1 out]
              n16 = local write "ns scale"("Time Resolution Per Bin(ns)") -> ()
              n17 = local write "y offset"("Accumulation Delay(ns)") -> ()
              n18 = local write "bins"("Number of Bins") -> ()
            }
          }
        }
        frame Disabled {
        }
      }
      n19 = local read "WS_On/Off"() -> (w4:bool)
      n20 = local read "Number of Bins"() -> (w8:u32)
      n21 = case shown="True" w4 {
        frame False {
        }
        frame True {
          n22 = call "T_RH_P.vi"("VISA in"="WS visa", "WS_Commands"=enum16{"OpenWS", "ReadTRHP", "CloseWS"}."OpenWS") -> ("TRHP"=→"TRHP":T13)  [unwired: 11 in, 2 out]
        }
      }
      n23 = Decrement(x=w8) -> (x-1=w7:u32)
      n24 = Subtract(x=w7, y="background length") -> (x-y=→"background start":u32)
      "Index" <- 0 ("Index")
    }
    frame #1 {
      # "Test to see if the lasers are on"
      # "Initializing the DBR's.  In this frame the online and offline DBR's are set to the front panel specified initial currents and then the Agiltron switch is toggled to the online channel"
      n25 = disable-structure shown="Disabled" {
        frame Disabled {
          # "Frame 0: Set the online DBR current, Frame 1: Generate a command for the offline DBR initialization but don't actually implement, Frame 2: Switch the \nAgiltron switch to the online channel"
          n26 = stacked-sequence {
            frame #0 {
              # "In this frame, two command strings are written the the ILX laser diode controller.  First, the string \"LAS:CHAN 1\" is written\nthe the ILX's GPIB address specifying that you want to write any following commands to the online channel,\n, then the string \"LAS:LDI 'Lamda On DBR Current'\" is written setting the current of the online channel (1) to the specified \ndiode current"
              n27 = flat-sequence {
                tunnel: [w67] -> w65
                tunnel: w65 -> [w69]
                frame #0 {
                  # "The GPIB address of the ILX controller"
                  # "Specifying laser channel 1,\nwhich is the online channel"
                  n28 = local write "ILX Address"("ILX Address") -> ()
                  n29 = Number To Decimal String(number="ILX Address") -> (decimal integer string=w67:string)  [unwired: 1 in]
                  n30 = GPIB Write(0:w67, 1:"LAS:CHAN 2") -> ()  [unwired: 3 in, 2 out]
                }
                frame #1 {
                  # "Telling the controller to\nset the current"
                  # "string formatter"
                  # "Set current to specified current"
                  n31 = Format Into String(format string="%.4f" ("Format String"), "Lambda On DBR Current") -> (resulting string=w72:string)  [unwired: 2 in, 1 out]
                  n32 = local write "Lambda On DBR Current"("Lambda On DBR Current") -> ()
                  n33 = Concatenate Strings("LAS:LDI ", w72) -> (w73:string)
                  n34 = GPIB Write(0:w69, 1:w73) -> ()  [unwired: 3 in, 2 out]
                }
              }
            }
            frame #1 {
              # "This frame does not actually appear to do anything, I'm not sure why Amin originally put anything in this frame.  What does occur, \nis that the output current for the offline channel is specified and a command is generated, but, not written, to enable the output of the\noffline laser.  Although, the command is never written, as nearly as I can figure, the idea was that the offline never actually needs to be \naltered, so it will just be left in whatever state it started in upon the program startup."
              n35 = local read "ILX Address"() -> (w75:i32)
              n36 = Number To Decimal String(number=w75) -> ()  [unwired: 1 in, 1 out]
              n37 = Number To Engineering String(4:"Lambda Off DBR Current") -> (0:w79:string)  [unwired: 3 in]
              n38 = local write "Lambda Off DBR Current"("Lambda Off DBR Current") -> ()
              n39 = Concatenate Strings(":SOUR2:FUNC DC; :SOUR2:VOLT:OFFS ", w79, "V; :OUTP2:STAT ON") -> ()  [unwired: 1 out]
            }
            frame #2 {
              # "REPLACE WITH NEW AGILTRON TASK!"
              # "First one"
              # "Address of the Agiltron switch, only altered if the COM port changes,\nif the USB to serial converter changes or the usb port that is is plugged\nin to changes, this may vary.  Check the \"Devices and Printers\" and find \nout which com port the Agiltron switch is under should you see an error \nand adjust the adress on the front panel to match the switch address"
              # "Hex command written to \nthe switch for the online channel"
              # "Switch the Agiltron switch to the online channel, once switched, the online DBR is the laser seeding the TSOA"
              n40 = local read "Switch Comm Port"() -> (w80:refnum<visa-resource-name>)
              n41 = VISA Write(VISA resource name=w80, write buffer="\u0001\u0012\u0000\u0002") -> ()  [unwired: 1 in, 3 out]
            }
          }
        }
        frame Enabled {
        }
      }
      n42 = call "TL_Driver.vi"("Device In"="Device In", "Commands"=T9."Open_TL", "Settings"="Settings") -> ("Device Out"=w45:refnum<visa-resource-name>)  [unwired: 9 in, 3 out]
      n43 = call "TL_Driver.vi"("Device In"=w45, "Commands"=T9."Read_Status", "Settings"="Settings") -> ("Device Out"=w42:refnum<visa-resource-name>, "Readings"=w43:T6)  [unwired: 9 in, 2 out]
      "Readings" <- w43
      n44 = Unbundle By Name(w43) -> ("OnLine LD"=w37:bool, "OffLine LD"=w38:bool)
      n45 = Compound Arithmetic op=AND(TRUE, w37, w38) -> (w36:bool)
      n46 = case shown="False" w36 {
        tunnel: w42 -> [w48 w51]
        tunnel: [w48 w51] -> w40
        frame False {
          n47 = One Button Dialog(message="LASERS NOT ON!", button name ("OK")="CONTINUE") -> ()  [unwired: 1 out]
        }
        frame True {
        }
      }
      n48 = disable-structure shown="Enabled" {
        frame Disabled {
          # "Initialize the ILX to the front panel temperatures and currents for the on line and off line DBRs\nTurn on the TECs - does not turn on the lasers or set the Agiltron switches"
          n49 = call "ILX2.vi"("ILX Command"=T10."Initialize ILX") -> ("Device Out"=w59:refnum<visa-resource-name>)  [unwired: 10 in, 4 out]
          n50 = call "ILX2.vi"("Device In"=w59, "TEC Control"=TRUE, "ILX Command"=T10."TEC ON/OFF") -> ("Device Out"=w56:refnum<visa-resource-name>)  [unwired: 8 in, 4 out]
          n51 = flat-sequence {
            tunnel: w56 -> [w63]
            tunnel: [w63] -> w53
            frame #0 {
              # "Wait 30 seconds for\nthe ILX to stabilize"
              n52 = Wait (ms)(milliseconds to wait=u32 30000) -> ()  [unwired: 1 out]
            }
          }
          n53 = call "ILX2.vi"("Device In"=w53, "ILX Command"=T10."LASER ON/OFF", "Laser Control"=TRUE ("TEC Control")) -> ("Device Out"=w52:refnum<visa-resource-name>)  [unwired: 8 in, 4 out]
          n54 = flat-sequence {
            tunnel: w52 -> [w61]
            tunnel: [w61] -> _
            frame #0 {
              # "Wait 5 seconds for\nthe ILX to stabilize"
              n55 = Wait (ms)(milliseconds to wait=u32 5000) -> ()  [unwired: 1 out]
            }
          }
        }
        frame Enabled {
        }
      }
      n56 = call "TL_Driver.vi"("Device In"=w40, "Commands"=T9."Read_Status", "Settings"="Settings") -> ("Readings"=w34:T6)  [unwired: 9 in, 3 out]
      n57 = local write "Readings"(w34) -> ()
      n58 = local write "Settings"("Settings") -> ()
    }
    frame #2 {
      # "Active X commands to the Newport 1918-C"
      # "Set the  channel of\nthe Newport 1918-C"
      # "Set the operational mode\nof the Newport 1918-C"
      # "Open commumication\nto the Newport 1918-C"
      n59 = constructor class="PowerMeterCommands"("logging"="logging", "deviceKey"="NewportIn") -> (reference out=w93:refnum<k24>, error out=w90:errorcluster, "deviceKey"=w85:string)  [unwired: 3 in, 2 out]
      "Newport Device Key" <- w85
      n60 = invoke class="PowerMeterCommands" method="GetPower"(reference=w93, error in=w90, "deviceKey"=w85) -> (reference out=w92:refnum<k24>, error out=w89:errorcluster)  [unwired: 1 in, 2 out]
      n61 = invoke class="PowerMeterCommands" method="SetChannel"(reference=w92, error in=w89, "deviceKey"=w85, "channel"="1") -> (reference out=w86:refnum<k24>, error out=w88:errorcluster)  [unwired: 1 in, 3 out]
      n62 = invoke class="PowerMeterCommands" method="CmdGetPower"(reference=w86, error in=w88, "deviceKey"=w85, "power"=sgl 0.0) -> (reference out=→"NewportRef":refnum<k24>)  [unwired: 1 in, 4 out]
    }
    frame #3 {
      # "Clean up multiply and divide by powers of 10 with comments\nBMM 6/19/14"
      # "Generating an array that is 'Number of Bins' long, filled wih the relevant altitude values for later plotting of Range \nCorrected Returns"
      # "Generating an array that is 'Number of Bins' long, filled wih the relevant altitude values for later plotting of returns"
      # "Generate arrays for the altitude and range corrected return altitude.  To be used later for plotting purposes."
      n63 = local read "Time Resolution Per Bin(ns)"() -> (w106:u32)
      n64 = local read "Time Resolution Per Bin(ns)"() -> (w96:u32)
      n65 = local read "Number of Bins"() -> (w109:u32)
      n66 = local read "Number of Bins"() -> (w99:u32)
      n67 = Divide(x=w106, y=1000000000.0) -> (x/y=w104:dbl)
      n68 = Divide(x=w96, y=1000000000.0) -> (x/y=w94:dbl)
      n69 = Multiply(x=w104, y=150000.0) -> (x*y=w107:dbl)
      n70 = Initialize Array(0.0, 0) -> (w112:dbl[])
      n71 = Multiply(x=w94, y=150000000.0) -> (x*y=w97:dbl)
      n72 = Initialize Array(0.0, 0) -> (w102:dbl[])
      n73 = for {
        N: w109 -> [_]
        shift-right: [w125] -> w110
        shift-left: w112 -> [w126]
        tunnel: w107 -> [w122]
        i -> [w124]
        n74 = Multiply(x=w122, y=w124) -> (x*y=w123:dbl)
        n75 = Add(x=w123, y=w122) -> (x+y=w121:dbl)
        n76 = Build Array (concatenate)(w126, w121) -> (w125:dbl[])
      }
      "Altitude Array (km)" <- w110
      n77 = for {
        N: w99 -> [_]
        shift-right: [w119] -> w100
        shift-left: w102 -> [w120]
        tunnel: w97 -> [w115]
        i -> [w118]
        n78 = Multiply(x=w115, y=w118) -> (x*y=w116:dbl)
        n79 = Add(x=w116, y=w115) -> (x+y=w114:dbl)
        n80 = Multiply(x=w114, y=w114) -> (x*y=w117:dbl)
        n81 = Build Array (concatenate)(w120, w117) -> (w119:dbl[])
      }
      "Range Corrected Altitude Array" <- w100
      n82 = local write "Altitude Array (km)"(w110) -> ()
      n83 = local write "Range Corrected Altitude Array"(w100) -> ()
    }
    frame #4 {
      # "Frame 4: Collect data from the scaler card and process and file it"
      n84 = while {
        tunnel: ["stop"] -> w127
        i -> [w128]
        stop <- "stop" stop-if-true
        # "While loop continues data collection cycle"
        n85 = case shown="True" "Collect Data?" {
          frame False {
            # "If 'Collect Data?' is false, wait a ms and check the 'Collect Data?' value again"
            n86 = Wait (ms)(milliseconds to wait=u32 1) -> ()  [unwired: 1 out]
          }
          frame True {
            # "Frame 3: Read the offline wavelength and lock if necessary (code not finished), read output power, read offline data, perform calculations and plot/save offline and NRB data, switch to online\nFrame 4: Calculate the absorption cross section (if wavelength, T, or P changed)\nFrame 5: Calculate Water Vapor Number density and plot"
            # "Frame 0: Create folders and file paths for logging the data, initialize averaging index\nFrame 1: Import current pressure and temperature data from COE weather station\nFrame 2: Read the online wavelength and lock if necessary, read online data and output power\n, plot and save online data, switch to offline DBR"
            # "If 'Collect Data?' is true, collect, process, and log data"
            n87 = stacked-sequence {
              frame #0 {
                # "Looking to see if the current Yr/Mo/Dy/Hr folder exists\nin the data disk folder (E:\\Micropulse_DIAL_data), if not,\ncreate one for the data"
                n88 = local read "FileHour"() -> (w141:i32)
                n89 = Get Date/Time In Seconds() -> (seconds since 1Jan1904=w133:timestamp)
                n90 = Seconds To Date/Time(time stamp (now)=w133) -> (date time rec=w143:T14)  [unwired: 1 in]
                n91 = Unbundle By Name(w143) -> ("hour"=w132:i32)
                n92 = Equal?(x=w141, y=w132) -> (x = y?=w142:bool)
                n93 = case shown="True" "Reset Average" {
                  frame False {
                    n94 = local write "Index"(0 ("Index")) -> ()
                  }
                  frame True {
                    n95 = local read "Index"() -> (w231:i32)
                    n96 = Add(x=w231, y=1) -> (x+y=w230:i32)
                    n97 = local write "Index"(w230) -> ()
                  }
                }
                n98 = Format Date/Time String(time format string (%c)="%y%m%d", seconds (now)=w133) -> (date/time string=w137:string)  [unwired: 1 in]
                n99 = Concatenate Strings("Data File DIR (in)", w137, "FF" ("string")) -> (w139:string)
                n100 = Concatenate Strings("Data File DIR (in)", w137, "NF" ("string")) -> (w134:string)
                n101 = case shown="False" w142 {
                  tunnel: w139 -> [w201 _]
                  tunnel: w134 -> [w200 _]
                  tunnel: w133 -> [w187 _]
                  tunnel: w132 -> [w163 _]
                  frame False {
                    # "Are data files open?"
                    # "Within the \"E:\\Micropulse_DIAL_data...\n'Current month/day/year' \ncheck if the current hour folder exists,\nif not, create one"
                    n102 = local write "FileHour"(w163) -> ()
                    n103 = flat-sequence {
                      tunnel: [w221] -> w188
                      tunnel: w201 -> [w220]
                      tunnel: w200 -> [w221]
                      tunnel: [w220] -> w189
                      frame #0 {
                        # "Does \"E:\\Micropulse_DIAL_data...\n'Current month/day/year' exist?\nIf not, create a new folder with that name"
                        n104 = String To Path(string=w220) -> (path=w225:path)
                        n105 = String To Path(string=w221) -> (path=w223:path)
                        n106 = call <vilib>:"Check if File or Folder Exists.vi"("path"=w225) -> ("file or folder exists?"=w224:bool)  [unwired: 8 in, 2 out]
                        n107 = call <vilib>:"Check if File or Folder Exists.vi"("path"=w223) -> ("file or folder exists?"=w222:bool)  [unwired: 8 in, 2 out]
                        n108 = case shown="False" w224 {
                          tunnel: w225 -> [w227 _]
                          frame False {
                            # "create new folder"
                            n109 = Create Folder(path (use dialog)=w227) -> ()  [unwired: 2 in, 3 out]
                          }
                          frame True {
                            # "Folder exists\ndo nothing"
                          }
                        }
                        n110 = case shown="False" w222 {
                          tunnel: w223 -> [w226 _]
                          frame False {
                            # "create new folder"
                            n111 = Create Folder(path (use dialog)=w226) -> ()  [unwired: 2 in, 3 out]
                          }
                          frame True {
                            # "Folder exists\ndo nothing"
                          }
                        }
                      }
                    }
                    n112 = Concatenate Strings(w189, "\\" ("string")) -> (w196:string)
                    n113 = Concatenate Strings(w188, "\\" ("string")) -> (w191:string)
                    n114 = Format Date/Time String(time format string (%c)="%H", seconds (now)=w187) -> (date/time string=w199:string)  [unwired: 1 in]
                    n115 = Format Date/Time String(time format string (%c)="%H", seconds (now)=w187) -> (date/time string=w194:string)  [unwired: 1 in]
                    n116 = Concatenate Strings(w196, w199) -> (w159:string)
                    "File Path_Far Field (out)" <- w159
                    n117 = Concatenate Strings(w191, w194) -> (w160:string)
                    "File Path_Near Field (out)" <- w160
                    n118 = String To Path(string=w159) -> (path=w197:path)
                    n119 = String To Path(string=w160) -> (path=w192:path)
                    n120 = call <vilib>:"Check if File or Folder Exists.vi"("path"=w197) -> ("file or folder exists?"=w186:bool, "dup path"=w184:path)  [unwired: 8 in, 1 out]
                    n121 = call <vilib>:"Check if File or Folder Exists.vi"("path"=w192) -> ("file or folder exists?"=w185:bool, "dup path"=w183:path)  [unwired: 8 in, 1 out]
                    n122 = case shown="False" w186 {
                      tunnel: w184 -> [w218 _]
                      tunnel: w159 -> [w217 w219]
                      tunnel: [w217 w219] -> w157
                      frame False {
                        # "new folder"
                        n123 = Create Folder(path (use dialog)=w218) -> ()  [unwired: 2 in, 3 out]
                      }
                      frame True {
                        # "Folder exists\ndo nothing"
                      }
                    }
                    n124 = case shown="False" w185 {
                      tunnel: w183 -> [w215 _]
                      tunnel: w160 -> [w214 w216]
                      tunnel: [w214 w216] -> w158
                      frame False {
                        # "new folder"
                        n125 = Create Folder(path (use dialog)=w215) -> ()  [unwired: 2 in, 3 out]
                      }
                      frame True {
                        # "Folder exists\ndo nothing"
                      }
                    }
                    n126 = Concatenate Strings(w158, "\\Online_Raw_Data.dat" ("string")) -> (w177:string)
                    n127 = Concatenate Strings(w158, "\\Offline_Raw_Data.dat" ("string")) -> (w176:string)
                    n128 = Concatenate Strings(w157, "\\Online_Raw_Data.dat" ("string")) -> (w182:string)
                    n129 = Concatenate Strings(w157, "\\Offline_Raw_Data.dat" ("string")) -> (w181:string)
                    n130 = local read "DataOpen"() -> (w174:bool)
                    n131 = String To Path(string=w182) -> (path=w173:path)
                    n132 = String To Path(string=w181) -> (path=w172:path)
                    n133 = String To Path(string=w177) -> (path=w171:path)
                    n134 = String To Path(string=w176) -> (path=w170:path)
                    n135 = case shown="True" w174 {
                      tunnel: w173 -> [w205 w209]
                      tunnel: [w205 w209] -> w167
                      tunnel: w172 -> [w204 w208]
                      tunnel: [w204 w208] -> w166
                      tunnel: w171 -> [w203 w207]
                      tunnel: [w203 w207] -> w165
                      tunnel: [w202 w206] -> w164
                      tunnel: w170 -> [w202 w206]
                      frame False {
                        # "No files open\ndo nothing"
                      }
                      frame True {
                        # "Close open files"
                        n136 = local read "NF_Off_Ref"() -> (w211:refnum<file>)
                        n137 = local read "NF_On_Ref"() -> (w210:refnum<file>)
                        n138 = local read "FF_Off_Ref"() -> (w213:refnum<file>)
                        n139 = local read "FF_On_Ref"() -> (w212:refnum<file>)
                        n140 = Close File(refnum=w212) -> ()  [unwired: 1 in, 2 out]
                        n141 = Close File(refnum=w213) -> ()  [unwired: 1 in, 2 out]
                        n142 = Close File(refnum=w210) -> ()  [unwired: 1 in, 2 out]
                        n143 = Close File(refnum=w211) -> ()  [unwired: 1 in, 2 out]
                      }
                    }
                    n144 = Open/Create/Replace File(file path (use dialog)=w167, operation (0:open)=T11."open or create") -> (refnum out=w153:refnum<file>)  [unwired: 4 in, 2 out]
                    n145 = Open/Create/Replace File(file path (use dialog)=w166, operation (0:open)=T11."open or create") -> (refnum out=w154:refnum<file>)  [unwired: 4 in, 2 out]
                    n146 = Open/Create/Replace File(file path (use dialog)=w165, operation (0:open)=T11."open or create") -> (refnum out=w155:refnum<file>)  [unwired: 4 in, 2 out]
                    n147 = Open/Create/Replace File(file path (use dialog)=w164, operation (0:open)=T11."open or create") -> (refnum out=w156:refnum<file>)  [unwired: 4 in, 2 out]
                    n148 = Get File Size(file=w153) -> (refnum out=→"FF_On_Ref":refnum<file>, size (in bytes)=→"FF_On_Ptr":i64)  [unwired: 1 in, 1 out]
                    n149 = Get File Size(file=w154) -> (refnum out=→"FF_Off_Ref":refnum<file>, size (in bytes)=→"FF_Off_Ptr":i64)  [unwired: 1 in, 1 out]
                    n150 = Get File Size(file=w155) -> (refnum out=→"NF_On_Ref":refnum<file>, size (in bytes)=→"NF_On_Ptr":i64)  [unwired: 1 in, 1 out]
                    n151 = Get File Size(file=w156) -> (refnum out=→"NF_Off_Ref":refnum<file>, size (in bytes)=→"NF_Off_Ptr":i64)  [unwired: 1 in, 1 out]
                  }
                  frame True {
                    # "Don't need to do anything!"
                  }
                }
              }
              frame #1 {
                # "Writing and plotting retrieved\nweather parameters"
                # "Matlab script goes online and retrieves most recent press, temp, and relative humidity data \nfrom the weather station on the roof of Cobleigh"
                # "Importing the current weather conditions from the COE weather station"
                n152 = disable-structure shown="Disabled" {
                  frame Disabled {
                    n153 = script code="%try\n%s=urlread('http://www.coe.montana.edu/ee/weather/mostCurrentCSV.php');\n%amin=textscan(s,'%s %s %s %s %s %s %s %s %s %s %s %s %s');\n%data=amin{1}{2};\n%[test remain]=strtok(data,',');\n%remain=str2num(remain);\n%press=remain(3)./1000;\n%temp=remain(5);\n%RH=remain(7);\n%catch\npress=.850;\ntemp=20;\nRH=40;\n%end"() -> ()  [unwired: 1 in, 4 out]
                  }
                  frame Enabled {
                  }
                }
                n154 = local read "WS_On/Off"() -> (w232:bool)
                n155 = case shown="True" w232 {
                  frame False {
                  }
                  frame True {
                    n156 = local read "WS visa"() -> (w237:refnum<visa-resource-name>)
                    n157 = call "T_RH_P.vi"("VISA in"=w237, "WS_Commands"=enum16{"OpenWS", "ReadTRHP", "CloseWS"}."ReadTRHP") -> ("TRHP"=w233:T13)  [unwired: 11 in, 2 out]
                    n158 = local write "TRHP"(w233) -> ()
                    n159 = Unbundle By Name(w233) -> ("Temp"=→"Temperature (C)":dbl, "RelH"=→"Relative Humdity (%)":dbl, "Press"=→"Pressure (mb)":dbl)
                  }
                }
              }
              frame #2 {
                # "Frame 3: Read, process, and plot online data\nFrame 4:\nFrame 5: Write the data to the folders from Frame 0 of outter sequence"
                # "Frame 0: Read the online wavelength and adjust to locking tolerance if out of range, Switch to offline DBR\nFrame 1: Read the output power from the Newport meter, calculate and plot the output pulse energy\nFrame 2: Wait 'Scalar Wait Time' for buffer to clear other wavelength data"
                # "Online"
                n160 = stacked-sequence {
                  frame #0 {
                    # "Read the online wavelength and continue adjusting the online DBR if outside the wavelength tolerance\nuntil it is within tolerance"
                    n161 = while {
                      i -> [w242]
                      stop <- w239 stop-if-true
                      # "Frame 2: Decrement DBR current if above tolerance\nFrame 3: Increment DBR current if below tolerance"
                      # "Frame 0: Read the current wavelength from the wavemeter\nFrame 1: Calculate the difference between desired and actual wavelength"
                      # "Continue reading and adjusting online DBR current until within locking tolerance"
                      n162 = stacked-sequence {
                        tunnel: w242 -> [w244 _ _ _ _]
                        tunnel: [_ _ w257 _ _] -> w240
                        frame #0 {
                          n163 = Equal To 0?(x=w244) -> (x = 0?=w243:bool)
                          n164 = case shown="True" w243 {
                            frame False {
                            }
                            frame True {
                              # "Set the TSOA switch to\namplify the ABSORBING\nwavelength"
                              n165 = Build Array(FALSE ("Boolean")) -> (w245:bool[])
                              n166 = call-poly <vilib>:"DAQmx Write.vi"("task/channels in"=refnum<k21> "BristolWM", "data"=w245) -> ()  [unwired: 11 in, 3 out]
                            }
                          }
                        }
                        frame #1 {
                          # "Reading the wavelength from the wavemeter"
                          n167 = flat-sequence {
                            tunnel: [w250] -> w249
                            tunnel: w249 -> [w253]
                            tunnel: [w252] -> w248
                            tunnel: w248 -> [w256]
                            frame #0 {
                              n168 = local read "Bristol In"() -> (w251:i32)
                              n169 = dll-call lib="C:/Users/H2ODial/Desktop/Shared Telescope WV DIAL Code/bristol/CLDevIface.dll" fn="CLOpenUSBSerialDevice"("commPort"=w251) -> ("return type"=w250:i32)  [unwired: 4 in, 2 out]
                            }
                            frame #1 {
                              n170 = dll-call lib="C:/Users/H2ODial/Desktop/Shared Telescope WV DIAL Code/bristol/CLDevIface.dll" fn="CLGetLambdaReading"("devHandle"=w253) -> ("return type"=→"Lambda On Read (nm)":dbl, "devHandle"=w252:i32)  [unwired: 3 in, 2 out]
                            }
                            frame #2 {
                              n171 = dll-call lib="C:/Users/H2ODial/Desktop/Shared Telescope WV DIAL Code/bristol/CLDevIface.dll" fn="CLCloseDevice"("commPort"=w256) -> ("return type"=w255:i32)  [unwired: 4 in, 2 out]
                              n172 = local write "Bristol Out"(w255) -> ()
                            }
                          }
                        }
                        frame #2 {
                          # "If WL difference is within tolerance, stop looping, and illuminate 'Wavelength Lock Online' indicator"
                          # "Calculating the difference between the actual and desired online wavelength"
                          n173 = local read "Lambda On Read (nm)"() -> (w265:dbl)
                          n174 = local read "Online_Tol"() -> (w262:dbl)
                          n175 = Multiply(x=-1.0, y=w262) -> (x*y=w263:dbl)
                          n176 = Subtract(x=w265, y="Lambda On Set (nm)") -> (x-y=w258:dbl)
                          "WL_Difference" <- w258
                          n177 = Greater?(x=w258, y=w263) -> (0:w259:bool)
                          n178 = Less?(x=w258, y=w262) -> (x < y?=w260:bool)
                          n179 = And(x=w259, y=w260) -> (x .and. y?=w257:bool)
                          "Wavelength Lock Online" <- w257
                        }
                        frame #3 {
                          # "If the wavelength difference is greater that 0.0002 nm, decrement the \nDBR current by 0.01 mA"
                          n180 = local read "WL_Difference"() -> (w268:dbl)
                          n181 = Greater Or Equal?(x=w268, y="Online_Tol") -> (x >= y?=w267:bool)
                          n182 = case shown="True" w267 {
                            frame False {
                              # "Wavelength difference is not greater than 0.0002 nm, do nothing"
                            }
                            frame True {
                              # "Generating a command string\nto decrement the current"
                              # "WL difference is greater than 0.0002 nm,\ndecrement the DBR current by 0.01 mA"
                              n183 = local read "Settings"() -> (w275:T7)
                              n184 = local read "y"() -> (w269:dbl)
                              n185 = Unbundle By Name(w275) -> ("OnLineTEC"=w273:dbl)
                              n186 = local read "Device In"() -> (w270:refnum<visa-resource-name>)
                              n187 = Subtract(x=w273, y=w269) -> (x-y=w272:dbl)
                              n188 = Bundle By Name(cluster=w275, "OnLineTEC"=w272, "Module"=T12."On Line TEC") -> (w277:T7)
                              n189 = call "TL_Driver.vi"("Device In"=w270, "Commands"=T9."SET", "Settings"=w277) -> ("Readings"=w276:T6)  [unwired: 9 in, 3 out]
                              n190 = local write "Settings"(w277) -> ()
                              n191 = local write "Readings"(w276) -> ()
                            }
                          }
                        }
                        frame #4 {
                          # "If WL difference is < 0.0002 nm, increment the DBR current"
                          n192 = local read "Online_Tol"() -> (w279:dbl)
                          n193 = local read "WL_Difference"() -> (w282:dbl)
                          n194 = Multiply(x=-1.0, y=w279) -> (x*y=w278:dbl)
                          n195 = Less Or Equal?(x=w282, y=w278) -> (x <= y?=w281:bool)
                          n196 = case shown="True" w281 {
                            frame False {
                              # "WL difference is no <= to -0.0002 nm, do nothing"
                            }
                            frame True {
                              # "WL difference is < -0.0002,\nincrement the DBR current by 0.01 mA"
                              # "Generating a command string\nto decrement the current"
                              n197 = local read "Settings"() -> (w291:T7)
                              n198 = Unbundle By Name(w291) -> ("OnLineTEC"=w287:dbl)
                              n199 = local read "y"() -> (w283:dbl)
                              n200 = local read "Device In"() -> (w284:refnum<visa-resource-name>)
                              n201 = Add(x=w287, y=w283) -> (x+y=w286:dbl)
                              n202 = Bundle By Name(cluster=w291, "OnLineTEC"=w286, "Module"=T12."On Line TEC") -> (w290:T7)
                              n203 = call "TL_Driver.vi"("Device In"=w284, "Commands"=T9."SET", "Settings"=w290) -> ("Readings"=w289:T6)  [unwired: 9 in, 3 out]
                              n204 = local write "Settings"(w290) -> ()
                              n205 = local write "Readings"(w289) -> ()
                            }
                          }
                        }
                      }
                      n206 = Or(x=w240, y="Cancel online") -> (x .or. y?=w239:bool)
                    }
                  }
                  frame #1 {
                    # "Converting to pulse energy, assumes 5 percent pickoff"
                    # "Reading the Newport Power meter"
                    # "Reading the output power of the laser transmitter from the Newport power meter, once read, convert to corresponding pulse energy and plot"
                    n207 = local read "Newport Device Key"() -> (w296:string)
                    n208 = local read "NewportRef"() -> (w292:refnum<k24>)
                    n209 = disable-structure shown="Disabled" {
                      frame Disabled {
                        # "Plotting the online and offling pulse energies"
                        n210 = local read "Online Pulse Energy"() -> (w307:dbl)
                        n211 = local read "Offline Pulse Energy"() -> (w306:dbl)
                        n212 = Bundle("Online Pulse Energy"=w307, "Offline Pulse Energy"=w306) -> (→"Pulse Energy (Micro Joule)":T15)  [unwired: 1 in]
                      }
                      frame Enabled {
                      }
                    }
                    n213 = Number To Decimal String(number="SampleSize") -> (decimal integer string=w294:string)  [unwired: 1 in]
                    n214 = invoke class="PowerMeterCommands" method="PerformDAQ"(reference=w292, "deviceKey"=w296, "interval"="1", "sampleSize"=w294) -> ("PerformDAQ"=w297:dbl[])  [unwired: 2 in, 5 out]
                    n215 = call-poly <vilib>:"Mean.vi"("X"=w297) -> ("mean"=w295:dbl)  [unwired: 1 out]
                    n216 = Multiply(x=w295, y=1000.0) -> (x*y=w303:dbl)
                    n217 = Divide(x=w303, y=0.05) -> (x/y=w301:dbl)
                    n218 = Divide(x=w301, y=7.0) -> (x/y=→"Online Pulse Energy":dbl)
                  }
                  frame #2 {
                    # "Wait 'Scalar Wait Time' for the next available batch of scalar card data"
                    n219 = local read "AMCS_Profile"() -> (w308:i32)
                    n220 = disable-structure shown="Disabled" {
                      frame Disabled {
                        # "Waiting 'Scalar Wait Time'"
                        n221 = Wait (ms)(milliseconds to wait="Scalar Wait Time") -> ()  [unwired: 1 out]
                      }
                      frame Enabled {
                      }
                    }
                    n222 = while {
                      tunnel: [w315] -> w309
                      tunnel: [w311] -> _
                      tunnel: w308 -> [w311]
                      stop <- w313 stop-if-true
                      n223 = global read "AMCS_Data.vi" "AMCS_Profile"() -> (w315:i32)
                      n224 = Wait (ms)(milliseconds to wait=u32 10) -> ()  [unwired: 1 out]
                      n225 = Equal?(x=w315, y=w311) -> (x = y?=w314:bool)
                      n226 = case shown="False" w314 {
                        tunnel: [TRUE FALSE] -> w313
                        frame False {
                        }
                        frame True {
                        }
                      }
                    }
                    "AMCS_Profile" <- w309
                  }
                  frame #3 {
                    # "convert time per range bin to meters\nand calculate smoothed bins using\nsmoothing range"
                    # "Plotting online cross section and smoothed online data"
                    # "Calculate the bin by bin mean of the data"
                    # "Collect 'Integration Period (Seconds)' number\nof scalar data"
                    # "Reading, processing, and plotting the online data"
                    n227 = local read "Data Reads (number of loops)"() -> (w343:i32)
                    n228 = for {
                      N: w343 -> [_]
                      tunnel: [w364] -> w355 mode=indexing
                      tunnel: [w363] -> w318 mode=indexing
                      # "Scalar Data is retrieved from Global \nVariable that scaler.vi is writing to,"
                      n229 = global read "AMCS_Data.vi" "AMCS_Data"() -> (w367:u16[][])
                      n230 = disable-structure shown="Disabled" {
                        frame Disabled {
                          n231 = global read "Scalar_Data_3.vi" "Scalar Data 3"() -> ()  [unwired: 1 out]
                          n232 = global read "Scalar_Data.vi" "Scalar Data"() -> ()  [unwired: 1 out]
                        }
                        frame Enabled {
                        }
                      }
                      n233 = Index Array(array=w367, index (row) #1=0 ("index (row)"), index (row) #2=2 ("index (row)")) -> (element #1=w364:u16[], element #2=w363:u16[])  [unwired: 2 in]
                    }
                    n234 = Transpose 2D Array(2D array=w355) -> (transposed array=w359:u16[][])
                    n235 = Transpose 2D Array(2D array=w318) -> (transposed array=w341:u16[][])
                    n236 = for {
                      tunnel: w359 -> [w369] mode=indexing
                      tunnel: [w368] -> w360 mode=indexing
                      n237 = call-poly <vilib>:"Mean.vi"("X"=w369) -> ("mean"=w368:dbl)  [unwired: 1 out]
                    }
                    n238 = for {
                      tunnel: w341 -> [w362] mode=indexing
                      tunnel: [w361] -> w342 mode=indexing
                      n239 = call-poly <vilib>:"Mean.vi"("X"=w362) -> ("mean"=w361:dbl)  [unwired: 1 out]
                    }
                    n240 = local read "bins"() -> (w335:u32)
                    n241 = Array Subset(array=w360, index=1 ("dimension size"), length=w335) -> (w347:dbl[])
                    n242 = Array Subset(array=w342, index=1 ("dimension size"), length=w335) -> (w339:dbl[])
                    n243 = local read "background length"() -> (w325:i32)
                    n244 = local read "background start"() -> (w326:u32)
                    n245 = Array Size(array=w347) -> (size(s)=w344:i32)
                    n246 = Array Size(array=w339) -> (size(s)=w336:i32)
                    n247 = Initialize Array(1.0 ("element"), w344) -> (w346:dbl[])
                    n248 = Initialize Array(1.0 ("element"), w336) -> (w338:dbl[])
                    n249 = Multiply(x=w347, y=w346) -> (x*y=w348:dbl[])
                    "On-Line Bin Readings" <- w348
                    n250 = Multiply(x=w339, y=w338) -> (x*y=w329:dbl[])
                    "On-Line Bin Readings 2" <- w329
                    n251 = local read "Total DIAL Integration Time (Minutes)"() -> (w351:i32)
                    n252 = local read "Time Resolution Per Bin(ns)"() -> (w321:u32)
                    n253 = Array Subset(array=w348, index=w326, length=w325) -> (w357:dbl[])
                    n254 = Array Subset(array=w329, index=w326, length=w325) -> (w331:dbl[])
                    n255 = call-poly <vilib>:"Mean.vi"("X"=w357) -> ("mean"=w356:dbl)  [unwired: 1 out]
                    n256 = call-poly <vilib>:"Mean.vi"("X"=w331) -> ("mean"=w332:dbl)  [unwired: 1 out]
                    n257 = Divide(x=w351, y=w343) -> (x/y=w349:dbl)
                    n258 = local read "Index"() -> (w330:i32)
                    n259 = Subtract(x=w348, y=w356) -> (x-y=w353:dbl[])
                    n260 = Subtract(x=w329, y=w332) -> (x-y=w333:dbl[])
                    n261 = To Double Precision Float(number=w321) -> (double precision float=w322:dbl)
                    n262 = Multiply(x=w349, y=60.0) -> (x*y=w327:dbl)
                    n263 = Multiply(x=w322, y=0.15) -> (x*y=w324:dbl)
                    n264 = call "Ring Buffer Online Far.vi"("Index"=w330, "Profiles to Average"=w327, "Input Array"=w353) -> ("AvgArray"=w352:dbl[])  [unwired: 7 in, 1 out]
                    n265 = call "Ring Buffer Online Near.vi"("Index"=w330, "Profiles to Average"=w327, "Input Array"=w333) -> ("AvgArray"=w334:dbl[])  [unwired: 7 in, 1 out]
                    n266 = Divide(x="Smoothing Range", y=w324) -> (x/y=w319:dbl)
                    "Smoothed Bins" <- w319
                    n267 = call "Smooth Arrray.vi"("smooth size"=w319, "Raw Array"=w352) -> ("Smoothed Array"=→"On-Line  Smoothed":dbl[])  [unwired: 9 in]
                    n268 = call "Smooth Arrray.vi"("smooth size"=w319, "Raw Array"=w334) -> ("Smoothed Array"=→"On-Line Smoothed 2":dbl[])  [unwired: 9 in]
                    n269 = disable-structure shown="Disabled" {
                      frame Disabled {
                        n270 = script code="format long;\ncounts=sum(Online);\nif counts >=0.5e6\ntime=time;\nelse\ntime=time\nend"() -> ()  [unwired: 3 in, 2 out]
                      }
                      frame Enabled {
                      }
                    }
                  }
                  frame #4 {
                    # "Toggling the Agiltron switch to the offline DBR seed laser"
                    n271 = disable-structure shown="Disabled" {
                      frame Disabled {
                        n272 = flat-sequence {
                          frame #0 {
                            # "Second one"
                            # "Command the switch to switch to position 2\ncorresponding to the offline DBR"
                            # "Hex string command \ncorrespond to offline"
                            n273 = VISA Write(VISA resource name="Switch Comm Port", write buffer="\u0001\u0012\u0000\u0001") -> ()  [unwired: 1 in, 3 out]
                          }
                        }
                      }
                      frame Enabled {
                      }
                    }
                  }
                  frame #5 {
                    # "Save the recently collected online data if 'Save Data?' is true"
                    n274 = case shown="True" "Save Data?" {
                      frame False {
                        # "'Save Data?' is false, do nothing"
                      }
                      frame True {
                        # "'Save Data?' is true, save onfline data to the Data Disk"
                        # "Write only one copy of data at this time"
                        # "Retrieve Julian Date"
                        n275 = local read "Time Resolution Per Bin(ns)"() -> (w378:u32)
                        n276 = local read "Number of Accumulates"() -> (w376:u32)
                        n277 = local read "Number of Bins"() -> (w377:u32)
                        n278 = local read "Lambda On DBR Current"() -> (w400:dbl)
                        n279 = local read "Lambda On Read (nm)"() -> (w401:dbl)
                        n280 = local read "On-Line Bin Readings 2"() -> (w398:dbl[])
                        n281 = local read "On-Line Bin Readings"() -> (w403:dbl[])
                        n282 = local read "Online Pulse Energy"() -> (w399:dbl)
                        n283 = To Double Precision Float(number=w378) -> (double precision float=w373:dbl)
                        n284 = To Double Precision Float(number=w377) -> (double precision float=w374:dbl)
                        n285 = To Double Precision Float(number=w376) -> (double precision float=w375:dbl)
                        n286 = call "Julian_Date_2.vi"() -> ("Julian Date"=w402:dbl)  [unwired: 11 in]
                        n287 = Build Array (concatenate)(w402, w401, w400, w399, w373, w374, w375, w403) -> (w393:dbl[])
                        n288 = Build Array (concatenate)(w402, w401, w400, w399, w373, w374, w375, w398) -> (w383:dbl[])
                        n289 = local write "DataOpen"(TRUE ("DataOpen")) -> ()
                        n290 = local read "NF_On_Ref"() -> (w381:refnum<file>)
                        n291 = local read "FF_On_Ref"() -> (w397:refnum<file>)
                        n292 = local read "NF_On_Ptr"() -> (w382:i64)
                        n293 = local read "FF_On_Ptr"() -> (w396:i64)
                        n294 = Set File Position(offset (in bytes) (0)=w396, refnum=w397) -> (refnum out=w394:refnum<file>, error out=w391:errorcluster)  [unwired: 2 in]
                        n295 = Set File Position(offset (in bytes) (0)=w382, refnum=w381) -> (refnum out=w387:refnum<file>, error out=w385:errorcluster)  [unwired: 2 in]
                        n296 = Write to Binary File(file (use dialog)=w387, data=w383, error in=w385, 5:FALSE ("prepend array or string size? (T)")) -> (refnum out=w386:refnum<file>, error out=w384:errorcluster)  [unwired: 2 in, 1 out]
                        n297 = Write to Binary File(file (use dialog)=w394, data=w393, error in=w391, 5:FALSE ("prepend array or string size? (T)")) -> (refnum out=w392:refnum<file>, error out=w390:errorcluster)  [unwired: 2 in, 1 out]
                        n298 = Get File Position(4:w384, 7:w386) -> (2:w380:i64)  [unwired: 2 out]
                        n299 = Get File Position(4:w390, 7:w392) -> (2:w389:i64)  [unwired: 2 out]
                        n300 = local write "NF_On_Ptr"(w380) -> ()
                        n301 = local write "FF_On_Ptr"(w389) -> ()
                      }
                    }
                  }
                }
              }
              frame #3 {
                # "Frame 3: Read offline data, calculate aerosol data, and plot offline and normalized relative backscatter\nFrame 4:\nFrame 5: Save the offline data and related information"
                # "Frame 0: Read the offline wavelength and lock if necessary, Switch to online DBR\nFrame 1: Read the output power from the Newport power meter\nFrame 2: Wait 'Scalar Wait Time' for buffers to clear of online contiminated data"
                # "offline"
                n302 = stacked-sequence {
                  frame #0 {
                    # "Every 60 data collection cycles, read the offline DBR wavelength, and if outside of wavelength tolerance, adjust DBR current until within tolerance"
                    n303 = local read "L_Count"() -> (w405:i32)
                    n304 = Quotient & Remainder(x=w405, y=60.0) -> (x-y*floor(x/y)=w406:dbl)  [unwired: 1 out]
                    n305 = Equal To 0?(x=w406) -> (x = 0?=w404:bool)
                    n306 = case shown="True" w404 {
                      frame False {
                      }
                      frame True {
                        n307 = while {
                          i -> [w411]
                          stop <- w409 stop-if-true
                          # "If WL difference is within tolerance, stop looping, and illuminate 'Wavelength Lock Offline' indicator"
                          # "Frame 2: Decrement DBR current if above tolerance\nFrame 3: Increment DBR current if below tolerance"
                          # "Frame 0: Read the current wavelength from the wavemeter\nFrame 1: Calculate the difference between desired and actual wavelength"
                          # "Continue reading and adjusting offline DBR current until within locking tolerance"
                          n308 = stacked-sequence {
                            tunnel: w411 -> [w413 _ _ _ _]
                            tunnel: [_ _ w427 _ _] -> w408
                            frame #0 {
                              n309 = Equal To 0?(x=w413) -> (x = 0?=w412:bool)
                              n310 = case shown="True" w412 {
                                frame False {
                                }
                                frame True {
                                # "Set the TSOA switch to\namplify the non ABSORBING\nwavelength"
                                n311 = Build Array(TRUE ("Boolean")) -> (w415:bool[])
                                n312 = call-poly <vilib>:"DAQmx Write.vi"("task/channels in"=refnum<k21> "BristolWM", "data"=w415) -> ()  [unwired: 11 in, 3 out]
                                n313 = Wait (ms)(milliseconds to wait=u32 3200) -> ()  [unwired: 1 out]
                                }
                              }
                            }
                            frame #1 {
                              # "Reading the wavelength from the wavemeter"
                              n314 = flat-sequence {
                                tunnel: [w420] -> w419
                                tunnel: w419 -> [w423]
                                tunnel: [w422] -> w418
                                tunnel: w418 -> [w426]
                                frame #0 {
                                n315 = local read "Bristol In"() -> (w421:i32)
                                n316 = dll-call lib="C:/Users/H2ODial/Desktop/Shared Telescope WV DIAL Code/bristol/CLDevIface.dll" fn="CLOpenUSBSerialDevice"("commPort"=w421) -> ("return type"=w420:i32)  [unwired: 4 in, 2 out]
                                }
                                frame #1 {
                                n317 = dll-call lib="C:/Users/H2ODial/Desktop/Shared Telescope WV DIAL Code/bristol/CLDevIface.dll" fn="CLGetLambdaReading"("devHandle"=w423) -> ("return type"=→"Lambda Off Read (nm)":dbl, "devHandle"=w422:i32)  [unwired: 3 in, 2 out]
                                }
                                frame #2 {
                                n318 = dll-call lib="C:/Users/H2ODial/Desktop/Shared Telescope WV DIAL Code/bristol/CLDevIface.dll" fn="CLCloseDevice"("commPort"=w426) -> ("return type"=w425:i32)  [unwired: 4 in, 2 out]
                                n319 = local write "Bristol Out"(w425) -> ()
                                }
                              }
                            }
                            frame #2 {
                              # "Calculating the difference between the actual and desired online wavelength"
                              n320 = local read "Offline_Tol"() -> (w429:dbl)
                              n321 = local read "Lambda Off Read (nm)"() -> (w435:dbl)
                              n322 = Multiply(x=-1.0, y=w429) -> (x*y=w428:dbl)
                              n323 = Subtract(x=w435, y="Lambda Off Set (nm)") -> (x-y=w431:dbl)
                              "WL Difference off" <- w431
                              n324 = Greater?(x=w431, y=w428) -> (0:w432:bool)
                              n325 = Less?(x=w431, y=w429) -> (x < y?=w433:bool)
                              n326 = And(x=w432, y=w433) -> (x .and. y?=w427:bool)
                              "Wavelength Lock Offline" <- w427
                              n327 = case shown="True" w427 {
                                frame False {
                                }
                                frame True {
                                # "Set the TSOA switch to\namplify the ABSORBING\nwavelength"
                                n328 = Build Array(FALSE ("Boolean")) -> (w437:bool[])
                                n329 = call-poly <vilib>:"DAQmx Write.vi"("task/channels in"=refnum<k21> "BristolWM", "data"=w437) -> ()  [unwired: 11 in, 3 out]
                                n330 = Wait (ms)(milliseconds to wait=u32 3200) -> ()  [unwired: 1 out]
                                }
                              }
                            }
                            frame #3 {
                              # "If the wavelength difference is greater that 0.0002 nm, decrement the \nDBR current by 0.01 mA"
                              n331 = local read "WL Difference off"() -> (w442:dbl)
                              n332 = Greater Or Equal?(x=w442, y="Offline_Tol") -> (x >= y?=w441:bool)
                              n333 = case shown="True" w441 {
                                frame False {
                                # "Wavelength difference is not greater than 0.0002 nm, do nothing"
                                }
                                frame True {
                                # "Generating a command string\nto decrement the current"
                                n334 = local read "Settings"() -> (w449:T7)
                                n335 = Unbundle By Name(w449) -> ("OffLineTEC"=w446:dbl)
                                n336 = Subtract(x=w446, y="y") -> (x-y=w445:dbl)
                                n337 = local read "Device In"() -> (w443:refnum<visa-resource-name>)
                                n338 = Bundle By Name(cluster=w449, "OffLineTEC"=w445, "Module"=T12."Off Line TEC") -> (w450:T7)
                                n339 = call "TL_Driver.vi"("Device In"=w443, "Commands"=T9."SET", "Settings"=w450) -> ("Readings"=w451:T6)  [unwired: 9 in, 3 out]
                                n340 = local write "Settings"(w450) -> ()
                                n341 = local write "Readings"(w451) -> ()
                                }
                              }
                            }
                            frame #4 {
                              # "If WL difference is < 0.0002 nm, increment the DBR current"
                              n342 = local read "WL Difference off"() -> (w454:dbl)
                              n343 = Less Or Equal?(x=w454, y=-0.0001) -> (x <= y?=w452:bool)
                              n344 = case shown="True" w452 {
                                frame False {
                                # "WL difference is no <= to -0.0002 nm, do nothing"
                                }
                                frame True {
                                # "Generating a command string\nto decrement the current"
                                # "WL difference is less than 0.0002 nm,\nincrement the DBR current by 0.01 mA"
                                n345 = local read "Settings"() -> (w462:T7)
                                n346 = Unbundle By Name(w462) -> ("OffLineTEC"=w459:dbl)
                                n347 = local read "y"() -> (w455:dbl)
                                n348 = Add(x=w459, y=w455) -> (x+y=w458:dbl)
                                n349 = local read "Device In"() -> (w456:refnum<visa-resource-name>)
                                n350 = Bundle By Name(cluster=w462, "OffLineTEC"=w458, "Module"=T12."Off Line TEC") -> (w463:T7)
                                n351 = call "TL_Driver.vi"("Device In"=w456, "Commands"=T9."SET", "Settings"=w463) -> ("Readings"=w461:T6)  [unwired: 9 in, 3 out]
                                n352 = local write "Settings"(w463) -> ()
                                n353 = local write "Readings"(w461) -> ()
                                }
                              }
                            }
                          }
                          n354 = Or(x=w408, y="Cancel Offline") -> (x .or. y?=w409:bool)
                        }
                      }
                    }
                  }
                  frame #1 {
                    # "Reading the power meter"
                    # "Updating the pulse energy plot"
                    # "Converting to pulse energy"
                    # "Reading the offline output power, converting to pulse energy,  and updating the Pulse energy plot"
                    n355 = local read "SampleSize"() -> (w466:i32)
                    n356 = local read "Newport Device Key"() -> (w467:string)
                    n357 = local read "Online Pulse Energy"() -> (w473:dbl)
                    n358 = local read "Offline Pulse Energy"() -> (w472:dbl)
                    n359 = local read "NewportRef"() -> (w464:refnum<k24>)
                    n360 = Number To Decimal String(number=w466) -> (decimal integer string=w468:string)  [unwired: 1 in]
                    n361 = invoke class="PowerMeterCommands" method="PerformDAQ"(reference=w464, "deviceKey"=w467, "interval"="1", "sampleSize"=w468) -> ("PerformDAQ"=w469:dbl[])  [unwired: 2 in, 5 out]
                    n362 = Bundle("Online Pulse Energy"=w473, "Offline Pulse Energy"=w472) -> (w471:T15)  [unwired: 1 in]
                    n363 = local write "Pulse Energy (Micro Joule)"(w471) -> ()
                    n364 = call-poly <vilib>:"Mean.vi"("X"=w469) -> ("mean"=w465:dbl)  [unwired: 1 out]
                    n365 = Multiply(x=w465, y=1000.0) -> (x*y=w478:dbl)
                    n366 = Divide(x=w478, y=0.05) -> (x/y=w476:dbl)
                    n367 = Divide(x=w476, y=7.0) -> (x/y=→"Offline Pulse Energy":dbl)
                  }
                  frame #2 {
                    # "Wait 'Scalar Wait Time' for buffers to clear of online contiminated offline data"
                    n368 = disable-structure shown="Disabled" {
                      frame Disabled {
                        # "Wait 'Scalar Wait Time'"
                        n369 = local read "Scalar Wait Time"() -> (w480:u32)
                        n370 = Wait (ms)(milliseconds to wait=w480) -> ()  [unwired: 1 out]
                      }
                      frame Enabled {
                      }
                    }
                  }
                  frame #3 {
                    w514 = 1 ("dimension size")
                    w518 = 1
                    # "Read in latest scalar card data from \n'Scalar Data' global variable that \nscaler.vi is writing to, then wait 1 sec\nfor next batch of data"
                    # "Plotting the normalized relative \nbackscatter"
                    # "Calculating the normalized relative backscatter"
                    # "Calculating/Plotting smoothed data,\ncross sections etc."
                    # "Pick off data with\nout header"
                    # "Calculate mean bin by bin mean"
                    # "Reading in 'Integration Period (Seconds)' of data"
                    # "Read the offline data from the scalar card, perform smoothing, calculate normalized relative backscatter, and plot"
                    # "File path in MATLAB script is of old dial is:\nF:\\Micropulse DIAL\\Micropulse DIAL Matlab\\\nFinal Overlap Function.mat')];"
                    # "Collects Data From Card,\nSends It To The Chart,\nAnd Saves A Copy As A\nFile If Option Selected On\nFront Panel"
                    n371 = for {
                      N: "Data Reads (number of loops)" -> [_]
                      tunnel: [w550] -> w482 mode=indexing
                      tunnel: [w549] -> w481 mode=indexing
                      n372 = global read "AMCS_Data.vi" "AMCS_Data"() -> (w551:u16[][])
                      n373 = disable-structure shown="Disabled" {
                        frame Disabled {
                          n374 = global read "Scalar_Data_4.vi" "Scalar Data 4"() -> ()  [unwired: 1 out]
                          n375 = global read "Scalar_Data_2.vi" "Scalar Data 2"() -> ()  [unwired: 1 out]
                        }
                        frame Enabled {
                        }
                      }
                      n376 = Index Array(array=w551, index (row) #1=1 ("index (row)"), index (row) #2=3 ("index (row)")) -> (element #1=w550:u16[], element #2=w549:u16[])  [unwired: 2 in]
                    }
                    n377 = local read "Total DIAL Integration Time (Minutes)"() -> (w539:i32)
                    n378 = Divide(x=w539, y="Data Reads (number of loops)") -> (x/y=w537:dbl)
                    n379 = local read "Total Aerosol Integration Time (Minutes)"() -> (w541:dbl)
                    n380 = local read "background length"() -> (w486:i32)
                    n381 = Multiply(x=w537, y=60.0) -> (x*y=w524:dbl)
                    n382 = local read "background start"() -> (w487:u32)
                    n383 = Transpose 2D Array(2D array=w482) -> (transposed array=w547:u16[][])
                    n384 = Transpose 2D Array(2D array=w481) -> (transposed array=w530:u16[][])
                    n385 = Divide(x=w541, y="Data Reads (number of loops)") -> (x/y=w542:dbl)
                    n386 = for {
                      tunnel: w547 -> [w557] mode=indexing
                      tunnel: [w556] -> w548 mode=indexing
                      tunnel: w530 -> [w555] mode=indexing
                      tunnel: [w554] -> _ mode=indexing
                      tunnel: [w554] -> w527 mode=indexing
                      n387 = call-poly <vilib>:"Mean.vi"("X"=w557) -> ("mean"=w556:dbl)  [unwired: 1 out]
                      n388 = call-poly <vilib>:"Mean.vi"("X"=w555) -> ("mean"=w554:dbl)  [unwired: 1 out]
                    }
                    n389 = local read "bins"() -> (w515:u32)
                    n390 = Multiply(x=w542, y=60.0) -> (x*y=w505:dbl)
                    n391 = Array Subset(array=w527, index=w514, length=w515) -> (w528:dbl[])
                    "Off-Line Bin Readings 2" <- w528
                    n392 = Array Subset(array=w548, index=w514, length=w515) -> (w526:dbl[])
                    "Off-Line  Bin Readings" <- w526
                    n393 = Array Subset(array=w528, index=w487, length=w486) -> (w529:dbl[])
                    n394 = Array Subset(array=w526, index=w487, length=w486) -> (w546:dbl[])
                    n395 = local read "Smoothed Bins"() -> (w483:dbl)
                    n396 = call-poly <vilib>:"Mean.vi"("X"=w529) -> ("mean"=w493:dbl)  [unwired: 1 out]
                    n397 = call-poly <vilib>:"Mean.vi"("X"=w546) -> ("mean"=w494:dbl)  [unwired: 1 out]
                    n398 = local read "Index"() -> (w504:i32)
                    n399 = Subtract(x=w528, y=w493) -> (x-y=w506:dbl[])
                    n400 = Subtract(x=w526, y=w494) -> (x-y=w522:dbl[])
                    n401 = call "Ring Buffer Offline Far.vi"("Index"=w504, "Profiles to Average"=w524, "Input Array"=w522) -> ("AvgArray"=w544:dbl[], "RingBufferOut"=→"RingBuffer offline far":dbl[][])  [unwired: 7 in]
                    n402 = call "Ring Buffer Aerosol Far.vi"("Index"=w504, "Profiles to Average"=w505, "Input Array"=w522) -> ("AvgArray"=w540:dbl[], "RingBufferOut"=→"RingBuffer aerosol far":dbl[][])  [unwired: 7 in]
                    n403 = call "Ring Buffer Offline Near.vi"("Index"=w504, "Profiles to Average"=w524, "Input Array"=w506) -> ("AvgArray"=w525:dbl[], "RingBufferOut"=→"RingBuffer offline near":dbl[][])  [unwired: 7 in]
                    n404 = call "Ring Buffer Aerosol Near.vi"("Index"=w504, "Profiles to Average"=w505, "Input Array"=w506) -> ("AvgArray"=w502:dbl[], "RingBufferOut"=→"RingBuffer aerosol near":dbl[][])  [unwired: 7 in]
                    n405 = Reshape Array(w522, w514, w515) -> (→"raw counts":dbl[][])
                    n406 = Reshape Array(w506, w514, w515) -> (→"raw counts near":dbl[][])
                    n407 = call "Smooth Arrray.vi"("smooth size"=w483, "Raw Array"=w544) -> ("Smoothed Array"=→"Off-Line Smoothed":dbl[])  [unwired: 9 in]
                    n408 = call "Smooth Arrray.vi"("smooth size"=w483, "Raw Array"=w540) -> ("Smoothed Array"=w513:dbl[])  [unwired: 9 in]
                    "Aerosol Smoothed" <- w513
                    n409 = call "Smooth Arrray.vi"("smooth size"=w483, "Raw Array"=w525) -> ("Smoothed Array"=→"Off-Line Smoothed 2":dbl[])  [unwired: 9 in]
                    n410 = call "Smooth Arrray.vi"("smooth size"=w483, "Raw Array"=w502) -> ("Smoothed Array"=w485:dbl[])  [unwired: 9 in]
                    "Aerosol Smoothed 2" <- w485
                    n411 = local read "Number of Accumulates"() -> (w489:u32)
                    n412 = local read "Temperature (C)"() -> (w536:dbl)
                    n413 = local read "Pressure (mb)"() -> (w535:dbl)
                    n414 = script code="%accum_num=10000;     % scaler card setting number of accumulations\nt_bin = 500e-9                 % scaler card setting time per bin\n%t_d = 37.3e-9;                % APD dead time from spec sheet\n\n% conversion from accumulated counts to count rate  (c/s)\nc_convert = 1./t_bin./accum_num;\nCR_far = p_raw_far.*c_convert;\nCR_near = p_raw_near.*c_convert;\nCR_total_far = (p_raw_far+b_far).*c_convert;\nCR_total_near = (p_raw_near+b_near).*c_convert;\nb_CR_far =b_far.*c_convert;\nb_CR_near =b_near.*c_convert;\n\n% create a range array\nsize_p =  size(p_raw_far,2);\nr = (75:75:size_p*75)./1e3; \n    \n%APD correction factor\n D_far = 1./(1-(t_d*CR_total_far));\n D_near = 1./(1-(t_d*CR_total_near));\n\n %Calculating normalize relative backscatter profile\n nrb_far = CR_far.*D_far.*r.^2.*1e-6;\n nrb_near = CR_near.*D_near.*r.^2.*1e-6;"("E"=6.0 ("Real"), "temp"=w536, "press"=w535, "p_raw_far"=w513, "b_far"=w494, "b_near"=w493, "p_raw_near"=w485, "accum_num"=w489, "t_d"="dead time") -> ("nrb_far"=w508:cdb[], "D_far"=w499:dbl[], "nrb_near"=w507:cdb[], "D_near"=w498:dbl[], "b_CR_far"=w491:dbl, "b_CR_near"=w490:dbl)  [unwired: 1 in, 1 out]
                    n415 = local read "bins"() -> (w517:u32)
                    n416 = local read "Altitude Array (km)"() -> (w510:dbl[])
                    n417 = Bundle(w491, w490) -> (→"?":cluster{dbl, dbl})  [unwired: 1 in]
                    n418 = Build Array(w508, w507) -> (w512:cdb[][])
                    n419 = Build Array(w499, w498) -> (w497:dbl[][])
                    n420 = Reshape Array(w507, w518, w517) -> (→"NRB 2":cdb[][])
                    n421 = Reshape Array(w508, w518, w517) -> (→"NRB":cdb[][])
                    n422 = Build Array(w510, w510) -> (w509:dbl[][])
                    n423 = call "Convert to Dynamic Data7"("2D Array"=w497) -> ("Dynamic Data Type"=w496:dynamicdata)  [unwired: 3 in]
                    n424 = call "Convert to Dynamic Data3"("2D Array"=w512) -> ("Dynamic Data Type"=w511:dynamicdata)  [unwired: 3 in]
                    n425 = call "Convert to Dynamic Data4"("2D Array"=w509) -> ("Dynamic Data Type"=w500:dynamicdata)  [unwired: 3 in]
                    n426 = call "Build XY Graph2"("Y Input"=w500, "X Input"=w511) -> ("XY Graph"=→"NRB plot":cluster{"Y":dbl[], "Y":dbl[]}[])  [unwired: 3 in, 6 out]
                    n427 = call "Build XY Graph4"("Y Input"=w500, "X Input"=w496) -> ("XY Graph"=→"Correction":cluster{"Y":dbl[], "Y":dbl[]}[])  [unwired: 3 in, 6 out]
                  }
                  frame #4 {
                    # "REPLACE WITH NEW AGILTRON TASK!"
                    # "Toggle Agiltron switch to online DBR"
                    n428 = disable-structure shown="Disabled" {
                      frame Disabled {
                        # "ABSORBING"
                        n429 = flat-sequence {
                          frame #0 {
                            # "Third one"
                            # "Command the switch to switch to position 1\ncorresponding to the online DBR"
                            # "Hex string command \ncorrespond to online"
                            n430 = local read "Switch Comm Port"() -> (w561:refnum<visa-resource-name>)
                            n431 = VISA Write(VISA resource name=w561, write buffer="\u0001\u0012\u0000\u0002") -> ()  [unwired: 1 in, 3 out]
                          }
                        }
                        n432 = Build Array(FALSE ("Boolean")) -> (w560:bool[])
                        n433 = call-poly <vilib>:"DAQmx Write.vi"("task/channels in"=refnum<k21> "AgiltronSwitch", "data"=w560) -> ()  [unwired: 11 in, 3 out]
                      }
                      frame Enabled {
                      }
                    }
                  }
                  frame #5 {
                    # "If 'Save Data?' is true, save all relavant offline info"
                    n434 = local read "Save Data?"() -> (w563:bool)
                    n435 = case shown="True" w563 {
                      frame False {
                        # "'Save Data?' is false, do nothing"
                      }
                      frame True {
                        # "Write only one data file at this time"
                        # "Retrive Julian Date"
                        # "'Save Data?' is true, save offline data to the Data Disk"
                        n436 = local read "Lambda Off DBR Current"() -> (w585:dbl)
                        n437 = local read "Off-Line Bin Readings 2"() -> (w582:dbl[])
                        n438 = local read "Lambda Off Read (nm)"() -> (w584:dbl)
                        n439 = local read "Off-Line  Bin Readings"() -> (w590:dbl[])
                        n440 = local read "Relative Humdity (%)"() -> (w589:dbl)
                        n441 = local read "Offline Pulse Energy"() -> (w586:dbl)
                        n442 = local read "Temperature (C)"() -> (w587:dbl)
                        n443 = local read "Pressure (mb)"() -> (w588:dbl)
                        n444 = call "Julian_Date_2.vi"() -> ("Julian Date"=w583:dbl)  [unwired: 11 in]
                        n445 = Build Array (concatenate)(w583, w584, w585, w586, w587, w588, w589, w590) -> (w568:dbl[])
                        n446 = Build Array (concatenate)(w583, w584, w585, w586, w587, w588, w589, w582) -> (w565:dbl[])
                        n447 = local read "FF_Off_Ref"() -> (w570:refnum<file>)
                        n448 = local read "NF_Off_Ref"() -> (w567:refnum<file>)
                        n449 = local read "FF_Off_Ptr"() -> (w569:i64)
                        n450 = local read "NF_Off_Ptr"() -> (w566:i64)
                        n451 = Set File Position(offset (in bytes) (0)=w569, refnum=w570) -> (refnum out=w581:refnum<file>, error out=w579:errorcluster)  [unwired: 2 in]
                        n452 = Set File Position(offset (in bytes) (0)=w566, refnum=w567) -> (refnum out=w577:refnum<file>, error out=w575:errorcluster)  [unwired: 2 in]
                        n453 = Write to Binary File(file (use dialog)=w581, data=w568, error in=w579, 5:FALSE ("prepend array or string size? (T)")) -> (refnum out=w580:refnum<file>, error out=w578:errorcluster)  [unwired: 2 in, 1 out]
                        n454 = Write to Binary File(file (use dialog)=w577, data=w565, error in=w575, 5:FALSE ("prepend array or string size? (T)")) -> (refnum out=w576:refnum<file>, error out=w574:errorcluster)  [unwired: 2 in, 1 out]
                        n455 = Get File Position(4:w578, 7:w580) -> (2:w571:i64)  [unwired: 2 out]
                        n456 = Get File Position(4:w574, 7:w576) -> (2:w564:i64)  [unwired: 2 out]
                        n457 = local write "FF_Off_Ptr"(w571) -> ()
                        n458 = local write "NF_Off_Ptr"(w564) -> ()
                      }
                    }
                  }
                }
              }
              frame #4 {
                n459 = First Call?() -> (First Call?: T/F=w593:bool)
                n460 = Or(x="calculate absorption cross sections", y=w593) -> (x .or. y?=w591:bool)
                n461 = case shown="True" w591 {
                  frame False {
                  }
                  frame True {
                    # "calculate absorption cross sections from HITRAN data base"
                    n462 = local read "Off-Line Smoothed"() -> (w594:dbl[])
                    n463 = local read "Lambda On Read (nm)"() -> (w597:dbl)
                    n464 = local read "Lambda Off Set (nm)"() -> (w600:dbl)
                    n465 = local read "Temperature (C)"() -> (w598:dbl)
                    n466 = local read "Pressure (mb)"() -> (w599:dbl)
                    n467 = script code="%Importing HITRAN data\n%hitran = dlmread('C:\\Users\\H2ODial\\Desktop\\Shared Telescope WV DIAL Code\\Libraries and VIs\\824nm_841nm_H2O.csv', ',',[0 1 352 7]);\nhitran = dlmread('C:\\Users\\H2ODial\\Desktop\\Shared Telescope WV DIAL Code\\Libraries and VIs\\824nm_841nm_H2O_Spectral_Calc.csv', ',',[1 1 1209 7]);\n\n%Range vector in meters\nrange = ([75:75:size(Online,2)*75]);\n\nif lambda< 828\nlambda=828.195;\nelse\nlambda=lambda;\nend;\n\n%%\n\n%Voigt profile calculation\nWNmin = 12070.0;\nWNmax = 12076.0;\n\n%Find lines from WNmin to WNmax to calculate voigt profile\nline_indices = find(hitran(1:size(hitran,1),1)>WNmin & hitran(1:size(hitran,1),1)<WNmax);\n\nline = (hitran(line_indices, 1:size(hitran,2)));\n\n%Calculate temperature and pressure profile\nT0 = 273+15.6;\nT0 = 273+T0_C;\n\nT = T0-0.005545.*range; \n\nP0  = 1.0;\nP0  = P0_mb/1000*0.986; %pressure in mb converted to atm\n\nP = P0.*(T0./T).^-5.21986;\n\n%linewidth temperature dependence factor\nalpha = line(:,7);        \n\n%initial Lorentz linewidth from HiTRAN [cm^-1]\ngammal0 = line(:,4);     \n\n%ground state transition energy [cm^-1]\nE = line(:,6);           \n\n%initial linestrength from HiTRAN [cm^-1/(mol*cm^-2)]\nS0 = line(:,2);      \n\n%absorption line center wavenumber from HiTRAN [cm^-1]\nnu0_0 = line(:,1);    \n\nnu_on = (1/(lambda)*1e7);\n\nnu_off = (1/(lambda_off)*1e7);\n\n\nfor i = 1:size(Online,2);\n\n    %Pressure shift\n    nu0 = nu0_0-.0428.*P(i);\n    \n    %Calculate Lorentz lineweidth at temperature T [cm^-1]\n    gammal = gammal0.*(P(i)./P0).*((T0./T(i)).^alpha);\n    \n    %Calculate Doppler linewidth at temperature T [cm^-1]\n    gammad = (nu0).*((2.0.*1.38E-23.*T(i).*log(2.0))./(0.018.*3.0E8.*3.0E8./6.022E23)).^(0.5);\n    \n    y = (gammal./gammad).*((log(2.0)).^(0.5));\n    \n    x_on = ((nu_on-nu0)./gammad).*(log(2.0)).^(0.5);\n    \n    x_off = ((nu_off-nu0)./gammad).*(log(2.0)).^(0.5);\n    \n    %setting up Voigt convolution\n    stepsize = 1;\n    \n    t = [-200:1:199].*stepsize;\n    \n    t = repmat(t',1,length(x_on))';\n    \n    x_on = repmat(x_on,1,length(t));\n    \n    x_off = repmat(x_off,1,length(t));\n    \n    y = repmat(y,1,length(t));\n    \n    f_on = (exp(-t.^2.0))./(y.^2.0+(x_on-t).^2.0);\n    \n    f_off = (exp(-t.^2.0))./(y.^2.0+(x_off-t).^2.0);\n    \n    %Set the integration sum to zero to start\n    integral_on = 0.0;\n    \n    integral_off = 0.0;\n    \n    %Voigt integration\n    z_on = trapz(t(1,:),f_on,2);\n    \n    z_off =  trapz(t(1,:),f_off,2);\n    \n    integral_on = z_on;\n    \n    integral_off = z_off;\n    \n    %Calculate linestrength at temperature T\n    S = S0.*((T0./T(i)).^(1.5)).*exp(1.439.*E.*((1./T0)-(1./T(i))));\n    \n    %Calculate Doppler line-center cross section [cm^2]\n    K = (S./gammad).*(((log(2.0))./pi).^(0.5));\n    \n    %Calculate the Voigt profile\n    V_on = (y(1)/pi).*integral_on;\n    \n    V_off = (y(1)./pi).*integral_off;\n    \n    %Calculate the Voigt profile absorption cross section [cm^2]\n    sigmav_on = K.*V_on;\n    \n    sigmav_off = K.*V_off;\n    \n    %Sum contributions from all of the surrounding lines\n    sigma_on_total(i) = sum(sigmav_on);\n    \n    sigma_off_total(i) = sum(sigmav_off);\n    \nend;"("lambda"=w597, "lambda_off"=w600, "P0_mb"=w599, "T0_C"=w598, "Online"=w594) -> ("sigma_on_total"=→"sigma_on_total":dbl[], "sigma_off_total"=→"sigma_off_total":dbl[])  [unwired: 1 in, 1 out]
                  }
                }
              }
              frame #5 {
                w611 = 1
                # "normalization factor\nfrom 300 to 450m"
                # "OPTICAL DEPTH PLOT"
                # "new rainbow color bar display"
                # "Data Processing Far Channel"
                # "new rainbow color bar display"
                # "Calculating the range resolved water vapor number density and plotting"
                n468 = local read "sigma_off_total"() -> (w634:dbl[])
                n469 = local read "sigma_on_total"() -> (w631:dbl[])
                n470 = local read "On-Line  Smoothed"() -> (w609:dbl[])
                n471 = local read "Off-Line Smoothed"() -> (w608:dbl[])
                n472 = local read "Off-Line Smoothed 2"() -> (w632:dbl[])
                n473 = local read "On-Line Smoothed 2"() -> (w633:dbl[])
                n474 = script code="%Time averaging in seconds.  600 Seconds =10 minutes\ntemporal_average = 600;\n\n%Spatial averaging in bins.  2 bins = 150 meters\nspatial_average = 2;\n\n%Creating r and r+deltar vectors..this can also be acsomplished using the\n%diff command\np_oni = Online(:,1:size(Online,2)-1);\n\np_onii = Online(:,2:size(Online,2));\n\np_offi = Offline(:,1:size(Offline,2)-1);\n\np_offii = Offline(:,2:size(Offline,2));\n\nInside = (p_oni.*p_offii)./(p_onii.*p_offi);\n\ndel_cross = 1./(2.*(sigma_on_total(1:size(Online,2)-1)-sigma_off_total(1:size(Offline,2)-1)).*75*100);\n\ndel_cross(isinf(del_cross)) = 0;\n\n%Calculating Number density\nN = del_cross.*log(Inside);\n\n%Spatial smoothing of the profiles\nfilter1 = ones(1,2)./2;\n\nN_1 = N;\n\nN_1_avg = filter2(filter1,N_1);\n\nfilter1 = ones(1,10)./10;\n\nN_2 = N;\n\nN_2_avg = filter2(filter1,N_2);\n\nN_new = zeros(size(N,1),size(N,2));\n \n%Using different averaging windows for different altitudes \nN_avg=[N_1_avg(:,1:40)';N_2_avg(:,41:size(N,2))']';\n\n\nw = N_avg.*1e6.*18.015./6.022e23"("Online"=w633, "Offline"=w632, "sigma_on_total"=w631, "sigma_off_total"=w634) -> ("N_avg"=w635:cdb[], "w"=w644:cdb[])  [unwired: 1 in, 1 out]
                n475 = script code="%Time averaging in seconds.  600 Seconds = 10 minutes\ntemporal_average = 600;\n\n%Spatial averaging in bins.  2 bins = 150 meters\nspatial_average = 2;\n\n%Creating r and r+deltar vectors..this can also be acsomplished using the\n%diff command\np_oni = Online(:,1:size(Online,2)-1);\n\np_onii = Online(:,2:size(Online,2));\n\np_offi = Offline(:,1:size(Offline,2)-1);\n\np_offii = Offline(:,2:size(Offline,2));\n\nInside = (p_oni.*p_offii)./(p_onii.*p_offi);\n\ndel_cross = 1./(2.*(sigma_on_total(1:size(Online,2)-1)-sigma_off_total(1:size(Offline,2)-1)).*75*100);\n\ndel_cross(isinf(del_cross)) = 0;\n\n%Calculating Number density\nN = del_cross.*log(Inside);\n\n%Spatial smoothing of the profiles\nfilter1 = ones(1,2)./2;\n\nN_1 = N;\n\nN_1_avg = filter2(filter1,N_1);\n\nfilter1 = ones(1,10)./10;\n\nN_2 = N;\n\nN_2_avg = filter2(filter1,N_2);\n\nN_new = zeros(size(N,1),size(N,2));\n \n%Using different averaging windows for different altitudes \nN_avg=[N_1_avg(:,1:40)';N_2_avg(:,41:size(N,2))']';\n\n \nw = N_avg.*1e6.*18.015./6.022e23"("Online"=w609, "Offline"=w608, "sigma_on_total"=w631, "sigma_off_total"=w634) -> ("N_avg"=w640:cdb[], "w"=w641:cdb[])  [unwired: 1 in, 1 out]
                n476 = local read "Time Resolution Per Bin(ns)"() -> (w610:u32)
                n477 = local read "bins"() -> (w636:u32)
                n478 = local read "Altitude Array (km)"() -> (w606:dbl[])
                n479 = Build Array(w641, w644) -> (w647:cdb[][])
                n480 = To Double Precision Float(number=w610) -> (double precision float=w629:dbl)
                n481 = Reshape Array(w640, w611, w636) -> (w651:cdb[][])
                n482 = Reshape Array(w635, w611, w636) -> (w638:cdb[][])
                n483 = Multiply(x=0.15, y=w629) -> (x*y=w627:dbl)
                n484 = Build Array(w640, w635) -> (w645:cdb[][])
                n485 = Divide(x=300.0, y=w627) -> (x/y=w624:dbl)
                n486 = Divide(x=450.0, y=w627) -> (x/y=w623:dbl)
                n487 = Build Array(w606, w606) -> (w630:dbl[][])
                n488 = call "Convert to Dynamic Data5"("2D Array"=w647) -> ("Dynamic Data Type"=w646:dynamicdata)  [unwired: 3 in]
                n489 = call "Convert to Dynamic Data2"("2D Array"=w645) -> ("Dynamic Data Type"=w642:dynamicdata)  [unwired: 3 in]
                n490 = Divide(x=w651, y=1e+17) -> (x/y=→"Water Vapor Number Density":cdb[][])
                n491 = Divide(x=w638, y=1e+17) -> (x/y=→"Water Vapor Number Density 2":cdb[][])
                n492 = call "Convert to Dynamic Data6"("Array"=w606) -> ("Dynamic Data Type"=w607:dynamicdata)  [unwired: 3 in]
                n493 = To Long Integer(number=w624) -> (32bit integer=w622:i32)
                n494 = To Long Integer(number=w623) -> (32bit integer=w621:i32)
                n495 = call "Convert to Dynamic Data"("2D Array"=w630) -> ("Dynamic Data Type"=w643:dynamicdata)  [unwired: 3 in]
                n496 = call "Convert to Dynamic Data8"("2D Array"=w630) -> ("Dynamic Data Type"=w648:dynamicdata)  [unwired: 3 in]
                n497 = Decrement(x=w622) -> (x-1=w619:i32)
                n498 = Decrement(x=w621) -> (x-1=w620:i32)
                n499 = call "Build XY Graph"("Y Input"=w643, "X Input"=w642) -> ("XY Graph"=→"Water Vapor Number Density  2":cluster{"Y":dbl[], "Y":dbl[]}[])  [unwired: 3 in, 6 out]
                n500 = call "Build XY Graph3"("Y Input"=w648, "X Input"=w646) -> ("XY Graph"=→"Absolute Humidity":cluster{"Y":dbl[], "Y":dbl[]}[])  [unwired: 3 in, 6 out]
                n501 = Array Subset(array=w609, index=w619, length=w620) -> (w618:dbl[])
                n502 = Array Subset(array=w608, index=w619, length=w620) -> (w617:dbl[])
                n503 = call-poly <vilib>:"Mean.vi"("X"=w618) -> ("mean"=w616:dbl)  [unwired: 1 out]
                n504 = call-poly <vilib>:"Mean.vi"("X"=w617) -> ("mean"=w615:dbl)  [unwired: 1 out]
                n505 = Divide(x=w616, y=w615) -> (x/y=w614:dbl)
                n506 = Multiply(x=w608, y=w614) -> (x*y=w613:dbl[])
                n507 = Divide(x=w609, y=w613) -> (x/y=w612:dbl[])
                n508 = Natural Logarithm(1:w612) -> (0:w603:dbl[])
                n509 = Multiply(x=-1.0, y=w603) -> (x*y=w602:dbl[])
                n510 = call "Convert to Dynamic Data9"("Array"=w602) -> ("Dynamic Data Type"=w605:dynamicdata)  [unwired: 3 in]
                n511 = call "Build OD Plot"("Y Input"=w607, "X Input"=w605) -> ("XY Graph"=→"Optical Depth":cluster{"Y":dbl[], "Y":dbl[]}[])  [unwired: 3 in, 6 out]
              }
            }
          }
        }
        "L_Count" <- w128
      }
    }
  }
  n512 = case shown="True" w3 {
    frame False {
    }
    frame True {
      # "close data files"
      n513 = local read "NF_Off_Ref"() -> (w655:refnum<file>)
      n514 = local read "NF_On_Ref"() -> (w656:refnum<file>)
      n515 = local read "FF_Off_Ref"() -> (w657:refnum<file>)
      n516 = local read "FF_On_Ref"() -> (w658:refnum<file>)
      n517 = local read "WS_On/Off"() -> (w654:bool)
      n518 = case shown="True" w654 {
        frame False {
        }
        frame True {
          n519 = local read "WS visa"() -> (w659:refnum<visa-resource-name>)
          n520 = call "T_RH_P.vi"("VISA in"=w659, "WS_Commands"=enum16{"OpenWS", "ReadTRHP", "CloseWS"}."CloseWS") -> ()  [unwired: 11 in, 3 out]
        }
      }
      n521 = Close File(refnum=w658) -> ()  [unwired: 1 in, 2 out]
      n522 = Close File(refnum=w657) -> ()  [unwired: 1 in, 2 out]
      n523 = Close File(refnum=w656) -> ()  [unwired: 1 in, 2 out]
      n524 = Close File(refnum=w655) -> ()  [unwired: 1 in, 2 out]
    }
  }
  "FileHour" <- -1 ("FileHour")
  "DataOpen" <- FALSE
